vi "Text control 2 v7.4_pump-specific.vi"() -> ()   [LabVIEW 2019]
panel:
  in  "Tab Control":enum32{"Main", "Other parameters"}(tab)
  out "Vdg vs time (Bias Stress)":cluster{"Y data in":dbl[], "X data in":dbl[]}[](graph)
  out "Vp vs Vg (FPP)":cluster{"Y data in":dbl[], "X data in":dbl[]}[](graph)
  out "Vp vs time (FPP Bias Stress)":cluster{"Y data in":dbl[], "X data in":dbl[]}[](graph)
  out "Line running":i32
  out "Total lines":i32
  out "Path":path=path "C:/users/rlp38/09Apr2009LTtesting/test2.txt"
  out "I vs Vg":cluster{"Y data in":dbl[], "X data in":dbl[]}[](graph)
  out "Is max":dbl format="%.2e"
  out "Id max":dbl format="%.2e"
  out "Ig max":dbl format="%.2e"
  out "Imax vs time":cluster{"Y data in":dbl[], "X data in":dbl[]}[](graph)
  out "Imin vs time":cluster{"Y data in":dbl[], "X data in":dbl[]}[](graph)
  out "I vs Vd":cluster{"Y data in":dbl[], "X data in":dbl[]}[](graph)
  in  "Script":string
  out "Command running:":string
  out "Serial port data":string
  out "Elapsed Time":dbl caption="Elapsed Time (s)"
  in  "Time Units":u16(ring)=1 items=["Seconds", "Minutes", "Hours"]
  in  "Time Offset":dbl caption="Set Start Time (s)"
  in  "Reset":bool
  in  "Auto Reset":bool
  in  "integration time":u32(slide) max=2 step=1 scale=0.0..2.0
  in  "Interrupt scan":bool
  out "Absolute plunger position vs time":cluster{"Y data in":dbl[], "X data in":dbl[]}[](graph)
  out "Valve position vs time":cluster{"Y data in":dbl[], "X data in":dbl[]}[](graph)
  out "Is on":dbl format="%.2e"
  out "Id on":dbl format="%.2e"
  out "Ig on":dbl format="%.2e"
  out "Ion vs time":cluster{"Y data in":dbl[], "X data in":dbl[]}[](graph)
  out "Ioff vs time":cluster{"Y data in":dbl[], "X data in":dbl[]}[](graph)
  out "Ig min":dbl format="%.2e"
  out "Id min":dbl format="%.2e"
  out "Is min":dbl format="%.2e"
  out "Is off":dbl format="%.2e"
  out "Id off":dbl format="%.2e"
  out "Ig off":dbl format="%.2e"
  in  "Integration time (long)":dbl=0.32 min=0.04 max=2.0 step=0.02 format="%.2f"
  in  "Integration time (short)":dbl=0.0019 min=8e-05 max=0.0019 step=8e-05 format="%^.0e"
  in  "Gate: Compliance":dbl=0.001 format="%.8f"
  in  "Drain: Compliance":dbl=0.001 format="%.8f"
  in  "Hard stop pump":bool
  in  "Halt pump":bool
  in  "Interrupt program":bool
  in  "Suffix (script)":string="step_1_up-H2O_initial_script.txt"
  in  "Filename (variable part)":string="step_1_up-H2O_initial_"
  in  "Plot output curve extrema vs time":bool
  in  "Plot transfer curve extrema vs time":bool=TRUE
  in  "Plot sample extrema vs time":bool
  out "I vs time (Bias Stress)":cluster{"Y data in":dbl[], "X data in":dbl[]}[](graph)
  out "Vp1":dbl format="%.2e"
  out "Vp2":dbl format="%.2e"
  in  "Sample I - Probe 4 (Disabled)":u32(ring)=3 items=["SMU1  ", "SMU2  ", "SMU3  ", "SMU4  ", "SMU5  ", "SMU6  ", "VSU1  ", "VSU2  "]
  in  "Sample I - Source/Common":u32(ring) items=["SMU1  ", "SMU2  ", "SMU3  ", "SMU4  ", "SMU5  ", "SMU6  ", "VSU1  ", "VSU2  "]
  in  "Sample I - Probe 3 (Disabled)":u32(ring)=2 items=["SMU1  ", "SMU2  ", "SMU3  ", "SMU4  ", "SMU5  ", "SMU6  ", "VSU1  ", "VSU2  "]
  in  "Sample I - Drain/Gate":u32(ring)=1 items=["SMU1  ", "SMU2  ", "SMU3  ", "SMU4  ", "SMU5  ", "SMU6  ", "VSU1  ", "VSU2  "]
  in  "Sample - Probe 4":u32(ring)=3 items=["SMU1  ", "SMU2  ", "SMU3  ", "SMU4  ", "SMU5  ", "SMU6  ", "VSU1  ", "VSU2  "]
  in  "Sample - Source/Common":u32(ring) items=["SMU1  ", "SMU2  ", "SMU3  ", "SMU4  ", "SMU5  ", "SMU6  ", "VSU1  ", "VSU2  "]
  in  "Sample - Gate":u32(ring)=2 items=["SMU1  ", "SMU2  ", "SMU3  ", "SMU4  ", "SMU5  ", "SMU6  ", "VSU1  ", "VSU2  "]
  in  "Sample - Drain":u32(ring)=1 items=["SMU1  ", "SMU2  ", "SMU3  ", "SMU4  ", "SMU5  ", "SMU6  ", "VSU1  ", "VSU2  "]
  in  "VSU2 Stress - Source/Common":u32(ring) items=["SMU1  ", "SMU2  ", "SMU3  ", "SMU4  ", "SMU5  ", "SMU6  ", "VSU1  "]
  in  "Stress I - Source/Common":u32(ring) items=["SMU1  ", "SMU2  ", "SMU3  ", "SMU4  ", "SMU5  ", "SMU6  ", "VSU1  ", "VSU2  "]
  in  "Stress I - Drain/Gate":u32(ring)=1 items=["SMU1  ", "SMU2  ", "SMU3  ", "SMU4  ", "SMU5  ", "SMU6  ", "VSU1  ", "VSU2  "]
  in  "Stress V - Source/Common":u32(ring) items=["SMU1  ", "SMU2  ", "SMU3  ", "SMU4  ", "SMU5  ", "SMU6  ", "VSU1  ", "VSU2  "]
  in  "Stress V - Gate":u32(ring)=2 items=["SMU1  ", "SMU2  ", "SMU3  ", "SMU4  ", "SMU5  ", "SMU6  ", "VSU1  ", "VSU2  "]
  in  "Stress V - Drain":u32(ring)=1 items=["SMU1  ", "SMU2  ", "SMU3  ", "SMU4  ", "SMU5  ", "SMU6  ", "VSU1  ", "VSU2  "]
  in  "FPP - Source":u32(ring)=6 items=["SMU1  ", "SMU2  ", "SMU3  ", "SMU4  ", "SMU5  ", "SMU6  ", "VSU1  ", "VSU2  "]
  in  "FPP - Probe 2":u32(ring)=3 items=["SMU1  ", "SMU2  ", "SMU3  ", "SMU4  ", "SMU5  ", "SMU6  ", "VSU1  ", "VSU2  "]
  in  "FPP - Probe 1":u32(ring) items=["SMU1  ", "SMU2  ", "SMU3  ", "SMU4  ", "SMU5  ", "SMU6  ", "VSU1  ", "VSU2  "]
  in  "FPP - Gate":u32(ring)=2 items=["SMU1  ", "SMU2  ", "SMU3  ", "SMU4  ", "SMU5  ", "SMU6  ", "VSU1  ", "VSU2  "]
  in  "FPP - Drain":u32(ring)=1 items=["SMU1  ", "SMU2  ", "SMU3  ", "SMU4  ", "SMU5  ", "SMU6  ", "VSU1  ", "VSU2  "]
  in  "Pulsed Stress V - Vextra":u32(ring)=6 items=["SMU1  ", "SMU2  ", "SMU3  ", "SMU4  ", "SMU5  ", "SMU6  ", "VSU1  ", "VSU2  "]
  in  "Pulsed Stress V - Probe 4":u32(ring)=3 items=["SMU1  ", "SMU2  ", "SMU3  ", "SMU4  ", "SMU5  ", "SMU6  ", "VSU1  ", "VSU2  "]
  in  "Pulsed Stress V - Source/Common":u32(ring) items=["SMU1  ", "SMU2  ", "SMU3  ", "SMU4  ", "SMU5  ", "SMU6  ", "VSU1  ", "VSU2  "]
  in  "Pulsed Stress V - Gate":u32(ring)=2 items=["SMU1  ", "SMU2  ", "SMU3  ", "SMU4  ", "SMU5  ", "SMU6  ", "VSU1  ", "VSU2  "]
  in  "Pulsed Stress V - Drain":u32(ring)=1 items=["SMU1  ", "SMU2  ", "SMU3  ", "SMU4  ", "SMU5  ", "SMU6  ", "VSU1  ", "VSU2  "]
  in  "Transfer/Output - Probe 4":u32(ring)=3 items=["SMU1  ", "SMU2  ", "SMU3  ", "SMU4  ", "SMU5  ", "SMU6  ", "VSU1  ", "VSU2  "]
  in  "Transfer/Output - Source/Common":u32(ring) items=["SMU1  ", "SMU2  ", "SMU3  ", "SMU4  ", "SMU5  ", "SMU6  ", "VSU1  ", "VSU2  "]
  in  "Transfer/Output - Gate":u32(ring)=2 items=["SMU1  ", "SMU2  ", "SMU3  ", "SMU4  ", "SMU5  ", "SMU6  ", "VSU1  ", "VSU2  "]
  in  "Transfer/Output - Drain":u32(ring)=1 items=["SMU1  ", "SMU2  ", "SMU3  ", "SMU4  ", "SMU5  ", "SMU6  ", "VSU1  ", "VSU2  "]
  in  "Gate Range\nmode":u16(ring) items=["Auto", "Limited", "Fixed"]
  in  "Gate Range":u8(slide)=3 max=11 scale=0.0..11.0
  in  "Source/Drain\nRange mode":u16(ring) items=["Auto", "Limited", "Fixed"]
  in  "Source/Drain Range":u8(slide)=3 max=11 scale=0.0..11.0
  in  "Panel Controls":T1={"Emergency Stop"=refnum, "TransGraph Max"=1e-05, "Text/Graph (text=false)"=TRUE} {"TransGraph Max" format="%.2e"}
  in  "Panel Controls 2":T2={"Emergency Stop"=refnum, "TransGraph Max"=1e-05, "Text/Graph (text=false)"=TRUE, "TransGraph Min"=1e-11} {"TransGraph Min" format="%.2e"; "TransGraph Max" format="%.2e"}
  in  "Probe 4":cluster{"on/off":bool, "Voltage":dbl} {"Voltage" min=-100.0 max=100.0 format="%.2f"}
  in  "Full Reset":bool
  in  "Standby":T3
  out "error out":errorcluster
  in  "Delay before read (ms)":u32=1000
  in  "byte count":u32=64
  in  "Serial End Mode for Reads":u16(ring)=2 items=["None", "LastBit", "TermChar"]
  in  "Timeout (ms)":u32=10000
  in  "Enable Termination\nChar (T)":bool=TRUE
  in  "Termination char\n(0xA = '\\n' = LF)\n(0xD = '\\r' = CR)":u8=13 format="%.0x"
  in  "flow control":u16(ring) items=["None"=0, "XON/XOFF"=1, "RTS/CTS"=2, "DTR/DSR"=4]
  in  "stop bits":u16(ring)=10 items=["1.0"=10, "1.5"=15, "2.0"=20]
  in  "parity":u16(ring) items=["None", "Odd", "Even", "Mark", "Space"]
  in  "data bits":u16=8 min=5 max=8 step=1
  in  "VISA resource name":refnum<visa-resource-name>="COM6"
  in  "baud rate":u32=9600
  out "Timings Indicator":T4 {"integration time" scale=0.0..2.0}
  in  "Timings (overwritten by the Front Panel)":T5={"integration time"=0, "Short/Long integration time"=0.00064, "hold time (sec)"=0.0, "delay time (sec)"=0.0, "Step Time (0 disables)"=0.0, "sweep method"=0, "Pulse period"=0.005, "Base voltage"=0.0, "Pulse width"=0.0005} {"Pulse width" min=0.0005 max=0.1 step=0.0001 format="%.4f"; "Base voltage" format="%^.4e"; "Pulse period" min=0.005 max=1.0 step=0.0001 format="%.4f"; "sweep method" items=["Continuous", "Pulsed"]; "Step Time (0 disables)" format="%.2f"; "delay time (sec)" format="%.4f"; "hold time (sec)" format="%.4f"; "Short/Long integration time" format="%^.0e"; "integration time" scale=0.0..2.0}
  out "Probe 4 Indicator":cluster{"on/off":bool, "Voltage":dbl} {"Voltage" min=-100.0 max=100.0 format="%.2f"}
  in  "VISA resource name in":refnum<visa-resource-name>="GPIB0::14::INSTR"
  in  "Gate":T6={"Gate Start"=0.0, "Gate Stop"=2.0, "Gate Step (linear only)"=1.0, "Gate Compliance"=0.0001, "Gate PComp"=0.0, "Range mode"=0, "Range"=6} {"Range" max=11 scale=0.0..11.0; "Range mode" items=["Auto", "Limited", "Fixed"]; "Gate PComp" format="%^.2e"; "Gate Compliance" format="%^.2e"; "Gate Step (linear only)" format="%^.4e"; "Gate Stop" format="%^.4e"; "Gate Start" format="%^.4e"}
  in  "Drain 2":T7={"Drain Start"=0.0, "Drain Stop"=2.0, "Drain Compliance"=0.0001, "Drain Step"=1.0, "Drain PComp"=0.0, "Range mode"=0, "Range"=6} {"Range" max=11 scale=0.0..11.0; "Range mode" items=["Auto", "Limited", "Fixed"]; "Drain PComp" format="%^.2e"; "Drain Step" format="%^.4e"; "Drain Compliance" format="%^.2e"; "Drain Stop" format="%^.4e"; "Drain Start" format="%^.4e"}
  # "Syntax:\nitime [s|m|l] time(sec): [s|m|l] determines the integration time setting (small|medium|long) and time sets the value.\nNOTE: The value of the integration time has to be within the range allowed by its category (s|m|l), otherwise, the closest value will be used. (e.g. if the category is set to short but the time value is very long, the actual value used will be the maximum short integration time.\nIntegration times:\n    Short: Default: 640 us. Range: 8E-5 - 1.92E-3 seconds.\n    Medium: Fixed at 1 NPL cycle (0.02 seconds).\n    Long: Default: 16 NPL cycles (0.32 seconds). Range: 2-100 NPL cycles (0.04 seconds - 2 seconds).\ngaterangemode [a|l|f]\ndrainrangemode [a|l|f]\npulsed [on|off] PulsePeriod(sec) PulseBaseVoltage PulseONWidth(sec)\nstandby [on l off]\nwait NumMilliseconds\nwait-min NumMinutes\n# texthere = comment\nProbe4 [ON|OFF] Voltage\ntransfer [s|d] VgStart VgStop VgStep VdStart VdStop VdStep\noutput [s|d] VgStart VgStop VgStep VdStart VdStop VdStep\nsample Vg Vd NumSamples Time(s) SampleInterval(s)\nsamplei Idg NumSamples Time(s) SampleInterval(s) VDGcompliance\n100 samples is approximately 13 seconds with medium integration\n# If in doubt use SampleInterval(s) = 0.004\n    NOTE: When doing bias stress measurements, it is best to set the Time Units to \"Seconds\", as the \"sample\" command has been configured to give the output to seconds.\nstressV VG VD IGcompliance IDcompliance Duration(sec)\nstressI IDG VDGcompliance Duration(sec)\nvsu2pulse Bias Duration(s)\npulsedstressV [s|d] VEstop VgON VgOFF Period(s) PulseONwidth(s) Vd\nsample-fpp Vg Vd NumSamples Time\nresample-fpp Vg Vd\ntransfer-fpp [s|d] VgStart VgStop VgStep VdStart VdStop VdStep\noutput-fpp [s|d] VgStart VgStop VgStep VdStart VdStop VdStep\nserial SerialPortCommand\npump SerialPortCommand for the SPM pump\nloop(No of iterations){Code}: Iterates the code provided (including nested loops)\n\nSPM Pump Syntax (<x>: pump number, use 1 if only one pump):\nif the command syntax contains [R], then append the letter R to the command\n/<x>Q: query (a query command should follow each command)\n/<x>Z[R] or /<x>Y[R]: initialize pump\n/<x>N<n>[R] (<n>=0,1): <0> (<1>) microstep 0.01 mm (0.00125 mm) resolution\n/<x>I<n>[R] (<n>=0-6): turn to port number n (clockwise)\n/<x>O<n>[R] (<n>=0-6): turn to port number n (counterclockwise)\n/<x>X: Re-execute last command string\n/<x>G<n>[R] (<n>=0-60000): repeat command sequence (default: 0, 0=loop forever)\n/<x>g: Mark the start of a repeat sequence (max = 10)\n/<x>M<n>[R] (<n>=0-86400000): delay command execution by n milliseconds\n/<x>H: Halt; Pause the sequence after finishing the current move\n/<x>T: Hardstop; Interrupt the current move and suppress it from the sequence\n/<x>A<n>[R] (<n>=0-3000 with N=0, 0-24000 with N=1): absolute position\n/<x>P<n>[R] (<n>=0-3000 with N=0, 0-24000 with N=1): relative pickup\n/<x>D<n>[R] (<n>=0-3000 with N=0, 0-24000 with N=1): relative dispense\n/<x>V<n>[R] (<n>=1-1600 default: 150): set peak speed (pulses/sec)\nNOTE: The lowest speed limit is 1 pulse/sec, not 5, as the manual states.\n/<x>S<n>[R] (<n>=10-40 default: 22): set speed (NOT in pulses/sec, look in manual)\nNOTE: When controlled with absolute position, one does not need to pay special attention to the syringe that is mounted on the pump.\nWithdraw from lower stage (ports 3, 5), dispense from higher stage (ports 2, 4, 6).\nConnect Port 1 to waste."
  # "Time"
  # "1\n2\n3\n4\n5\n6\n7\n8\n9\n10\n11\n12\n13\n14\n15\n16\n17\n18\n19\n20"
  # "Serial port settings"
  # "SMUs"
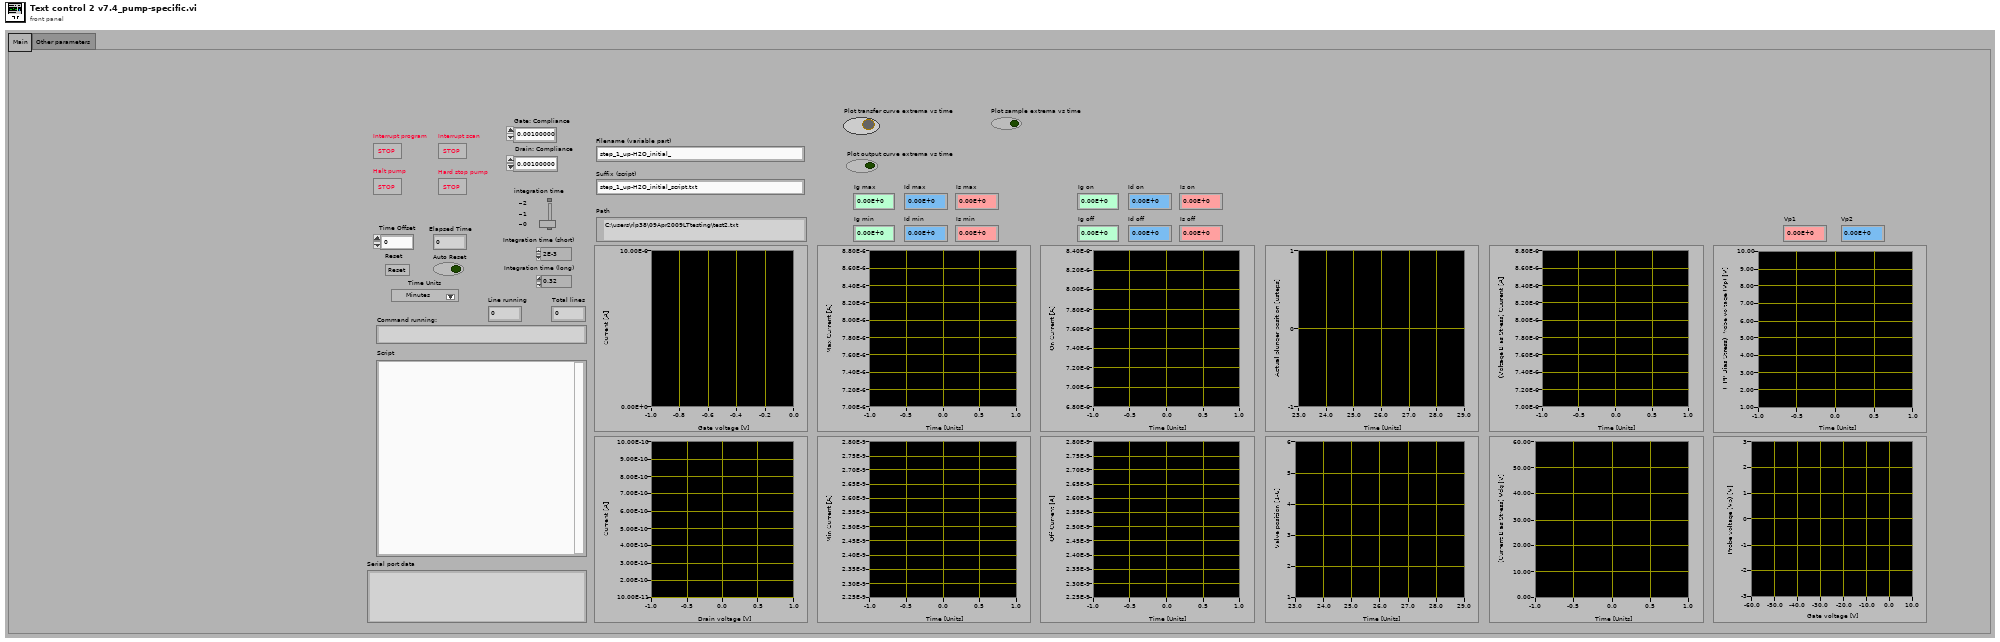
[diagram p1: front panel]
types:
  T1 = cluster{"Emergency Stop":refnum<vi>, "TransGraph Max":dbl, "Text/Graph (text=false)":bool}
  T2 = cluster{"Emergency Stop":refnum<vi>, "TransGraph Max":dbl, "Text/Graph (text=false)":bool, "TransGraph Min":dbl}
  T3 = cluster{"Gate Standby":bool, "Drain Standby":bool}
  T4 = cluster{"Short/Long integration time":dbl, "hold time (sec)":dbl, "delay time (sec)":dbl, "Step Time (0 disables)":dbl, "sweep method":u16, "Pulse period":dbl, "Base voltage":dbl, "Pulse width":dbl, "integration time":u32}
  T5 = cluster{"integration time":u32, "Short/Long integration time":dbl, "hold time (sec)":dbl, "delay time (sec)":dbl, "Step Time (0 disables)":dbl, "sweep method":u16, "Pulse period":dbl, "Base voltage":dbl, "Pulse width":dbl}
  T6 = cluster{"Gate Start":dbl, "Gate Stop":dbl, "Gate Step (linear only)":dbl, "Gate Compliance":dbl, "Gate PComp":dbl, "Range mode":u16, "Range":u8}
  T7 = cluster{"Drain Start":dbl, "Drain Stop":dbl, "Drain Compliance":dbl, "Drain Step":dbl, "Drain PComp":dbl, "Range mode":u16, "Range":u8}
  T8 = enum16{"open", "replace", "create", "open or create", "replace or create", "replace or create with confirmation"}
  T9 = cluster{"V2 Start":dbl, "V2 Step":dbl, "Number of points":i32}
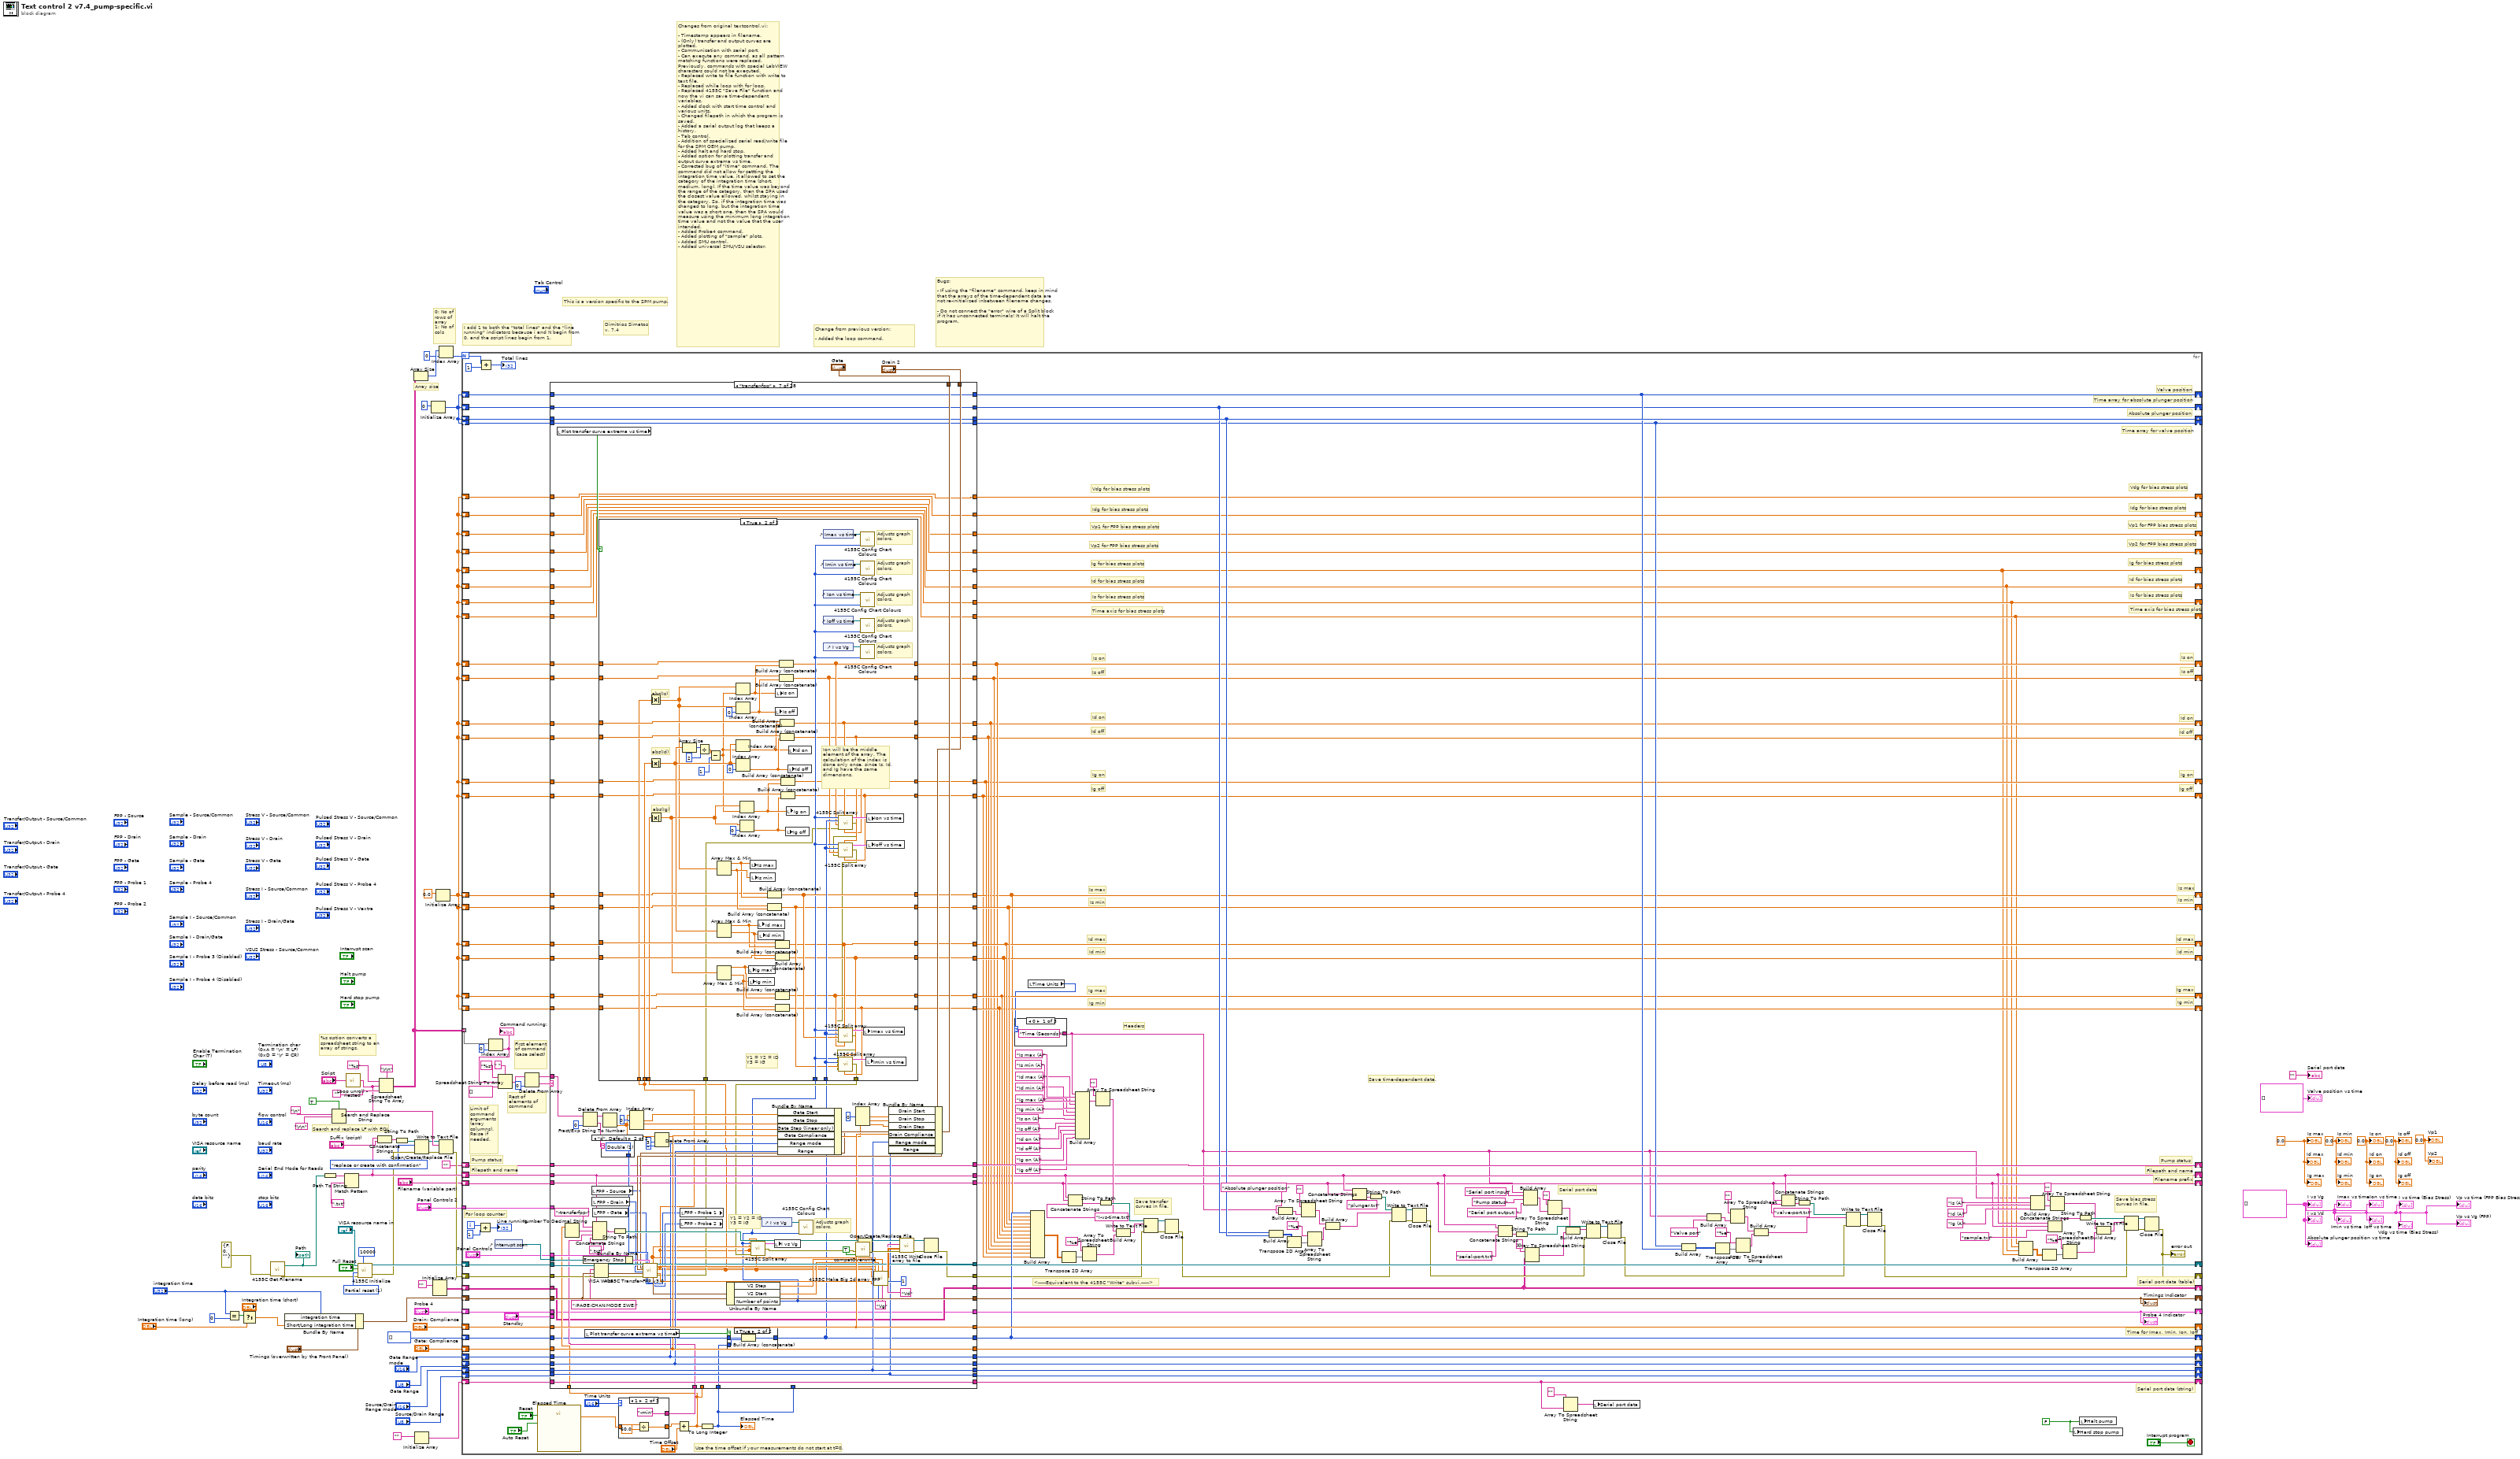
[diagram p0: block diagram]
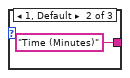
[diagram p2: hidden frame]
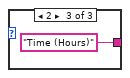
[diagram p3: hidden frame]
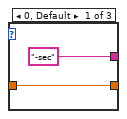
[diagram p4: hidden frame]
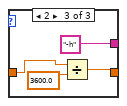
[diagram p5: hidden frame]
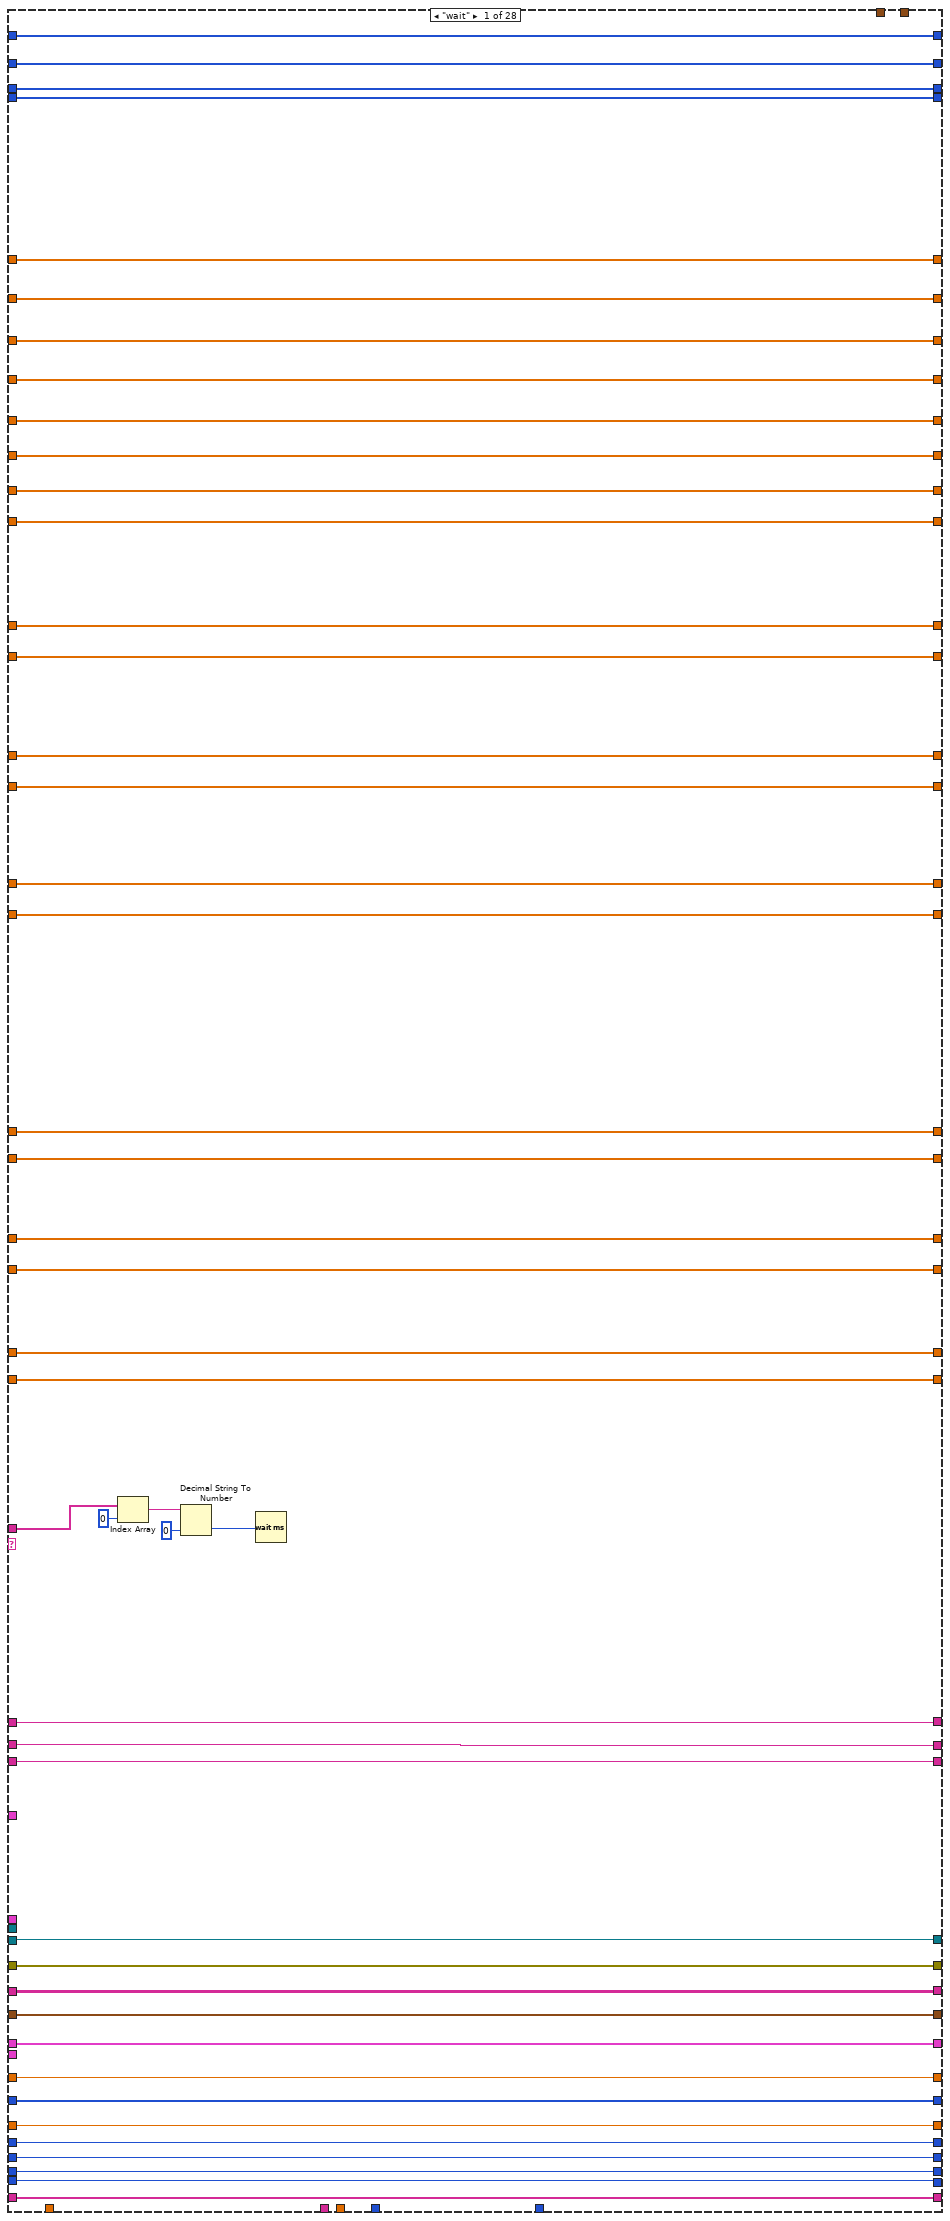
[diagram p6: hidden frame]
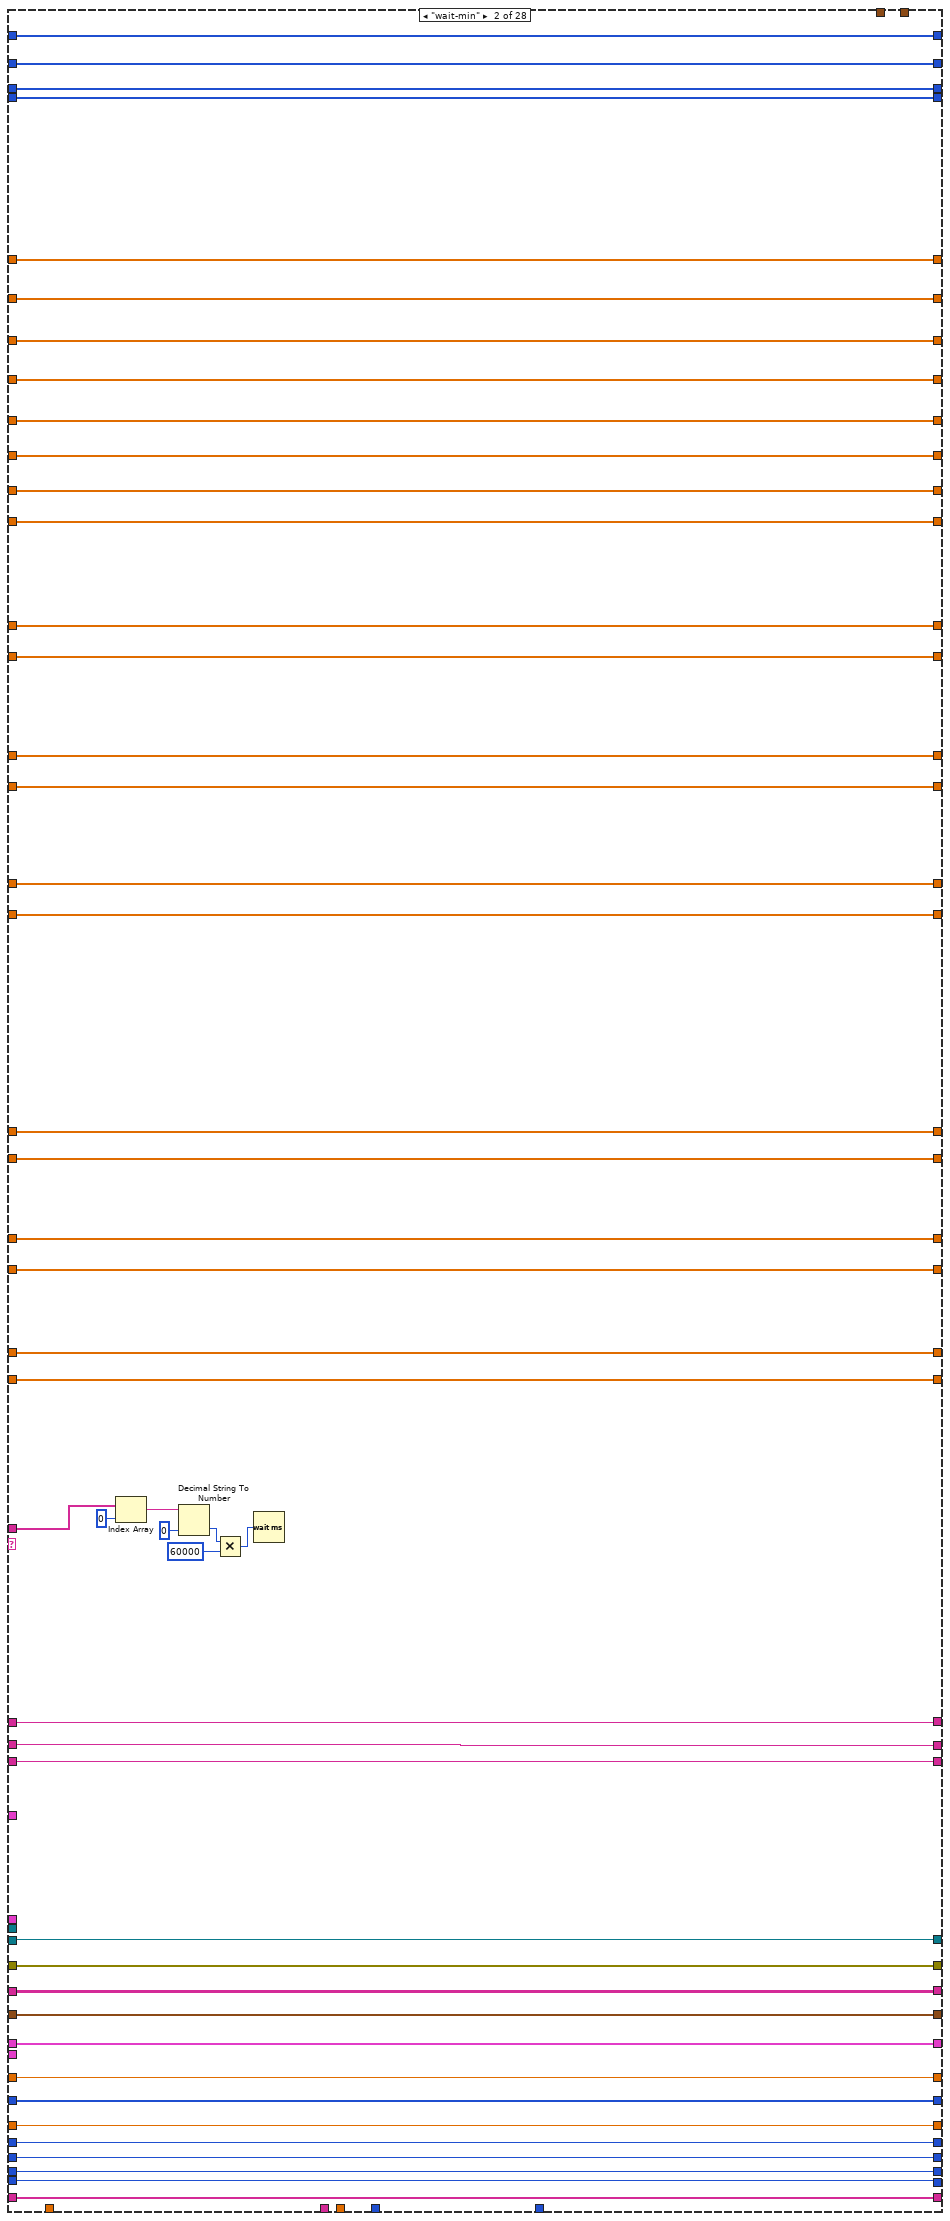
[diagram p7: hidden frame]
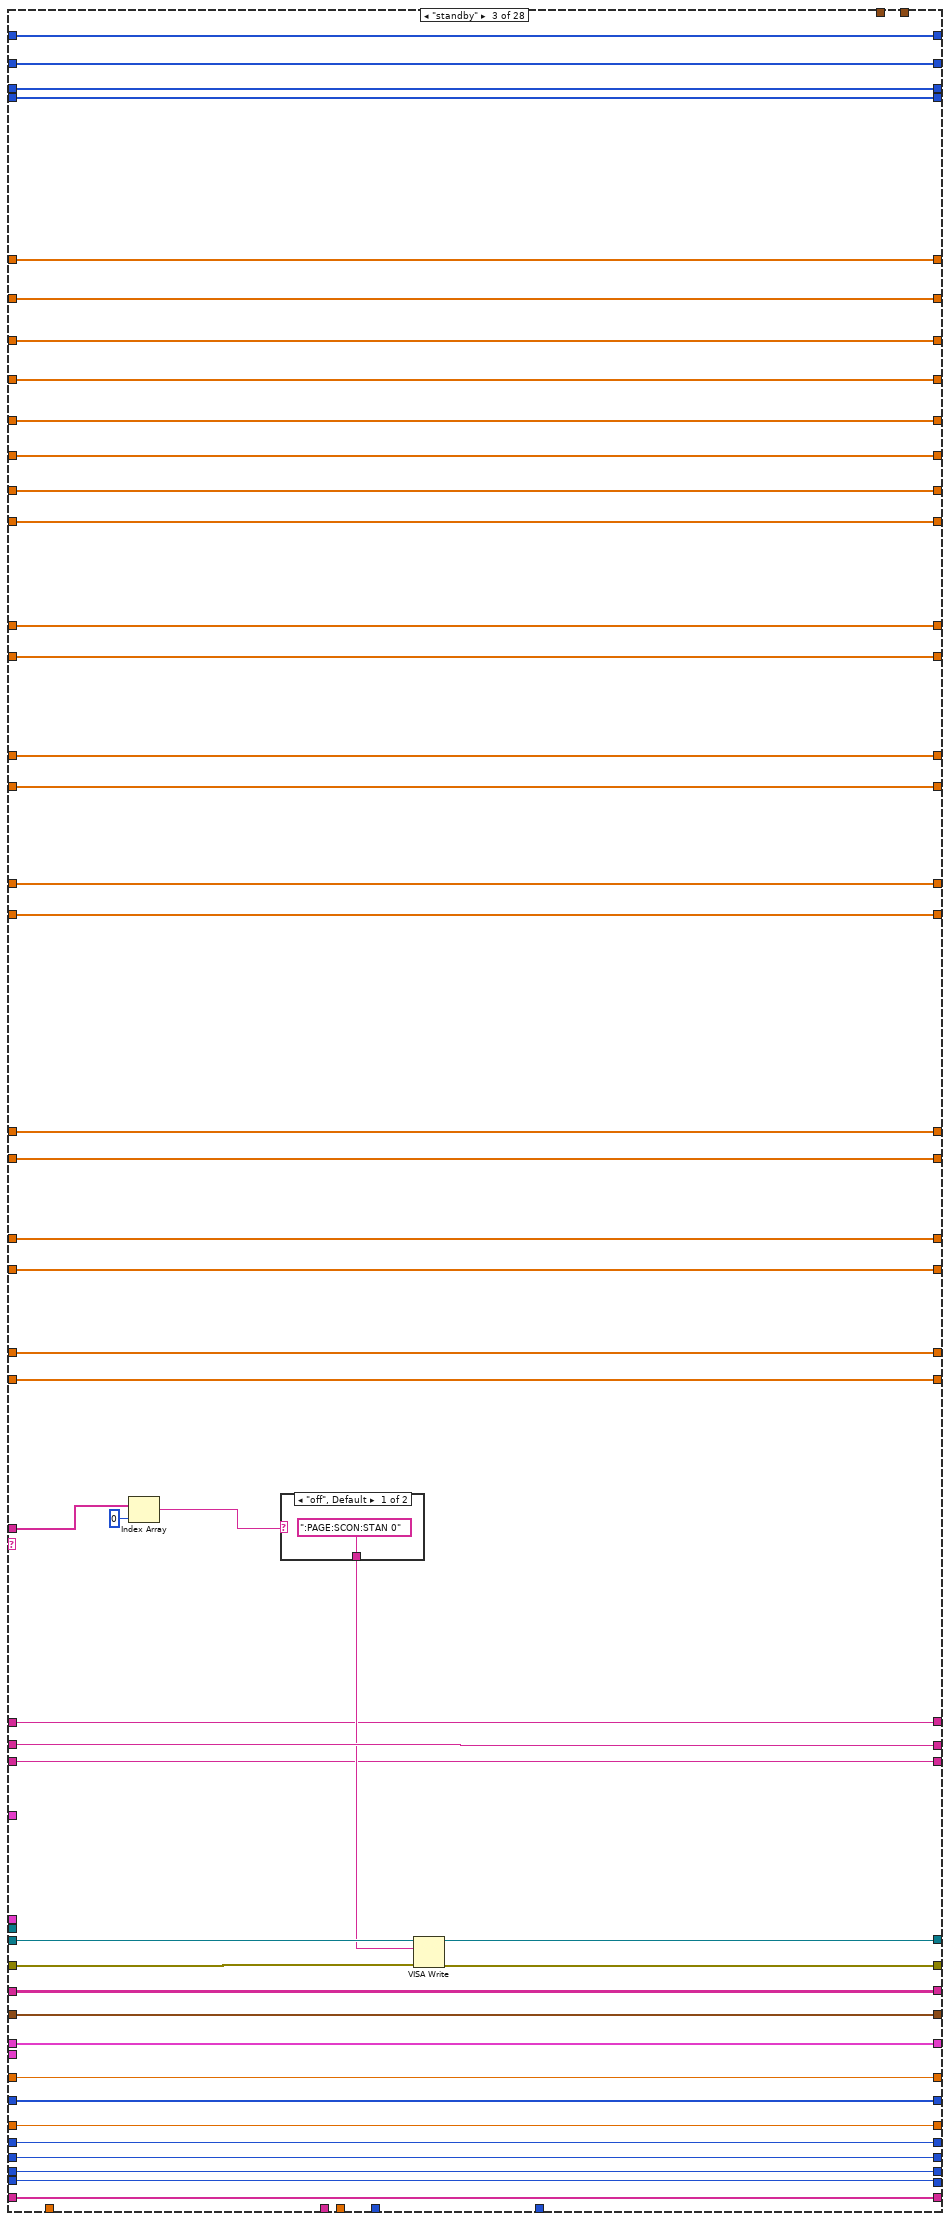
[diagram p8: hidden frame]
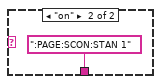
[diagram p9: hidden frame]
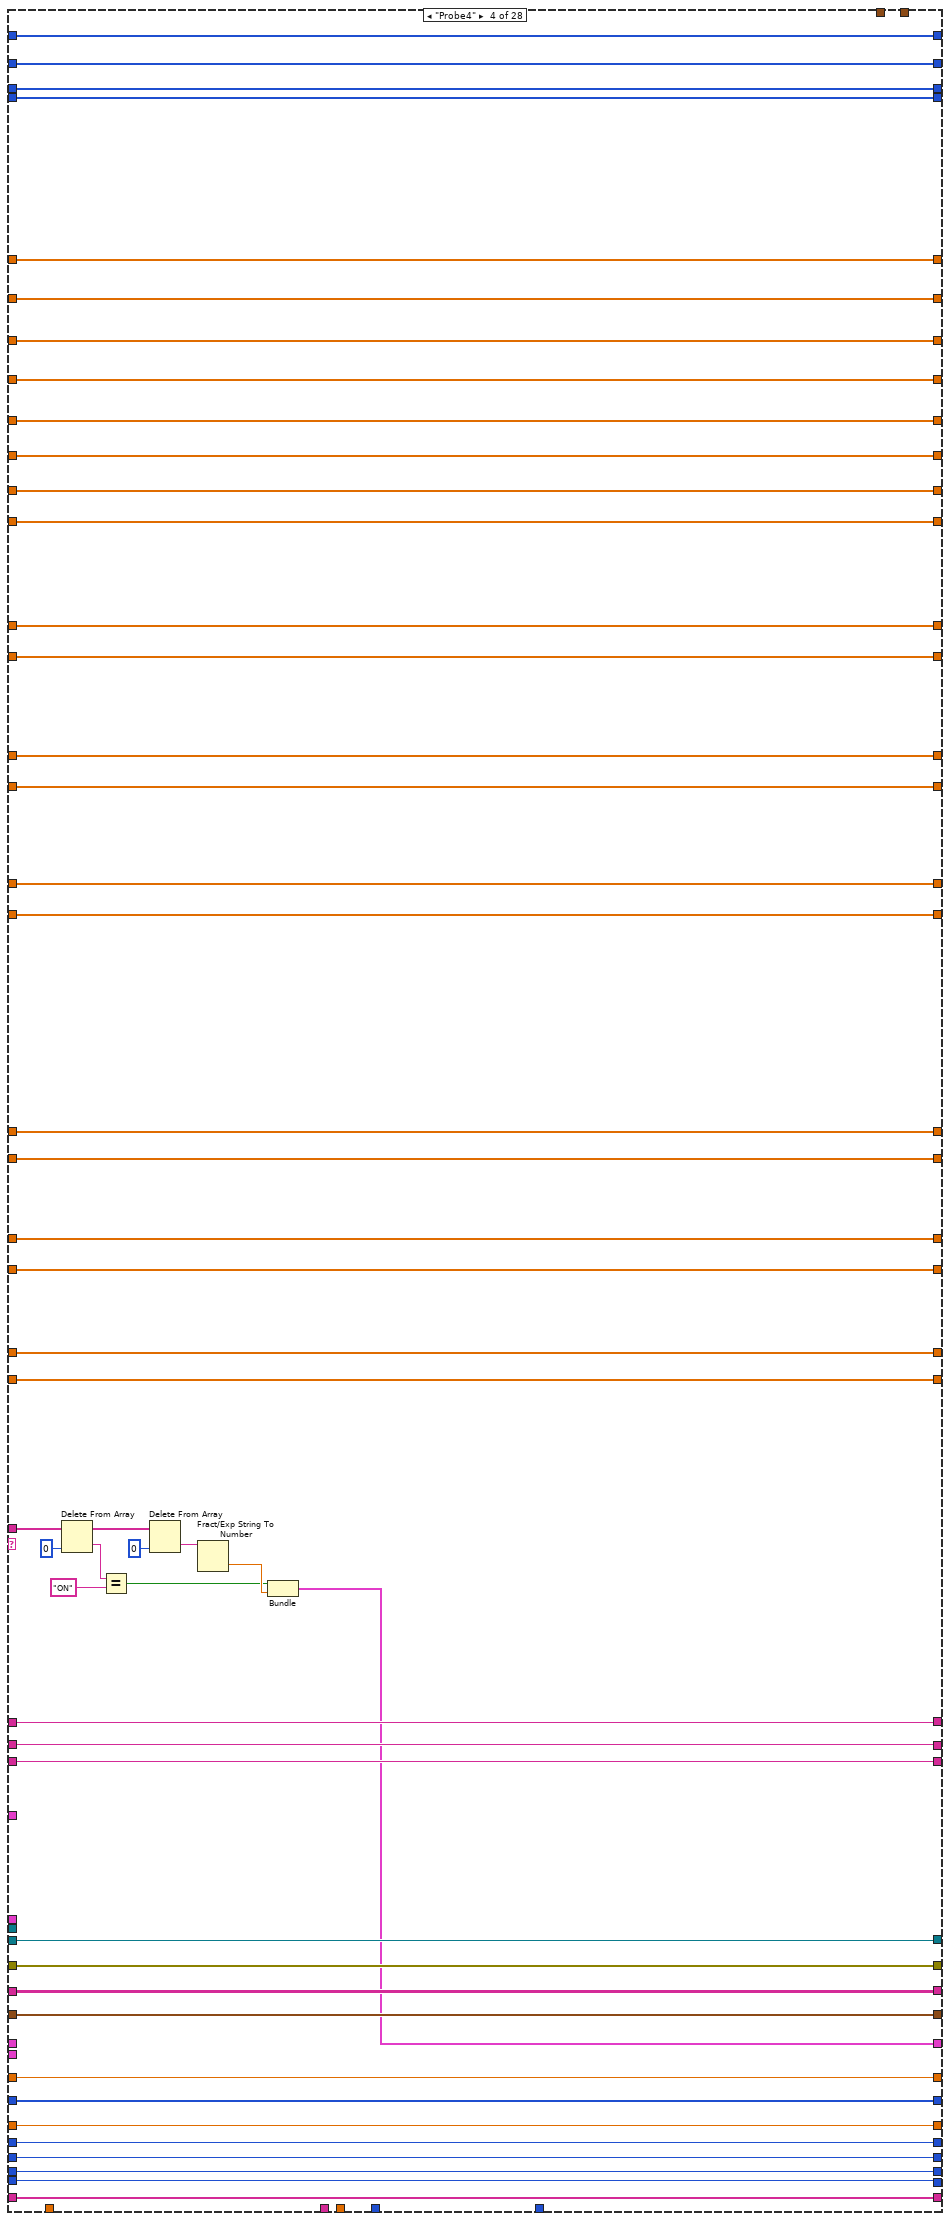
[diagram p10: hidden frame]
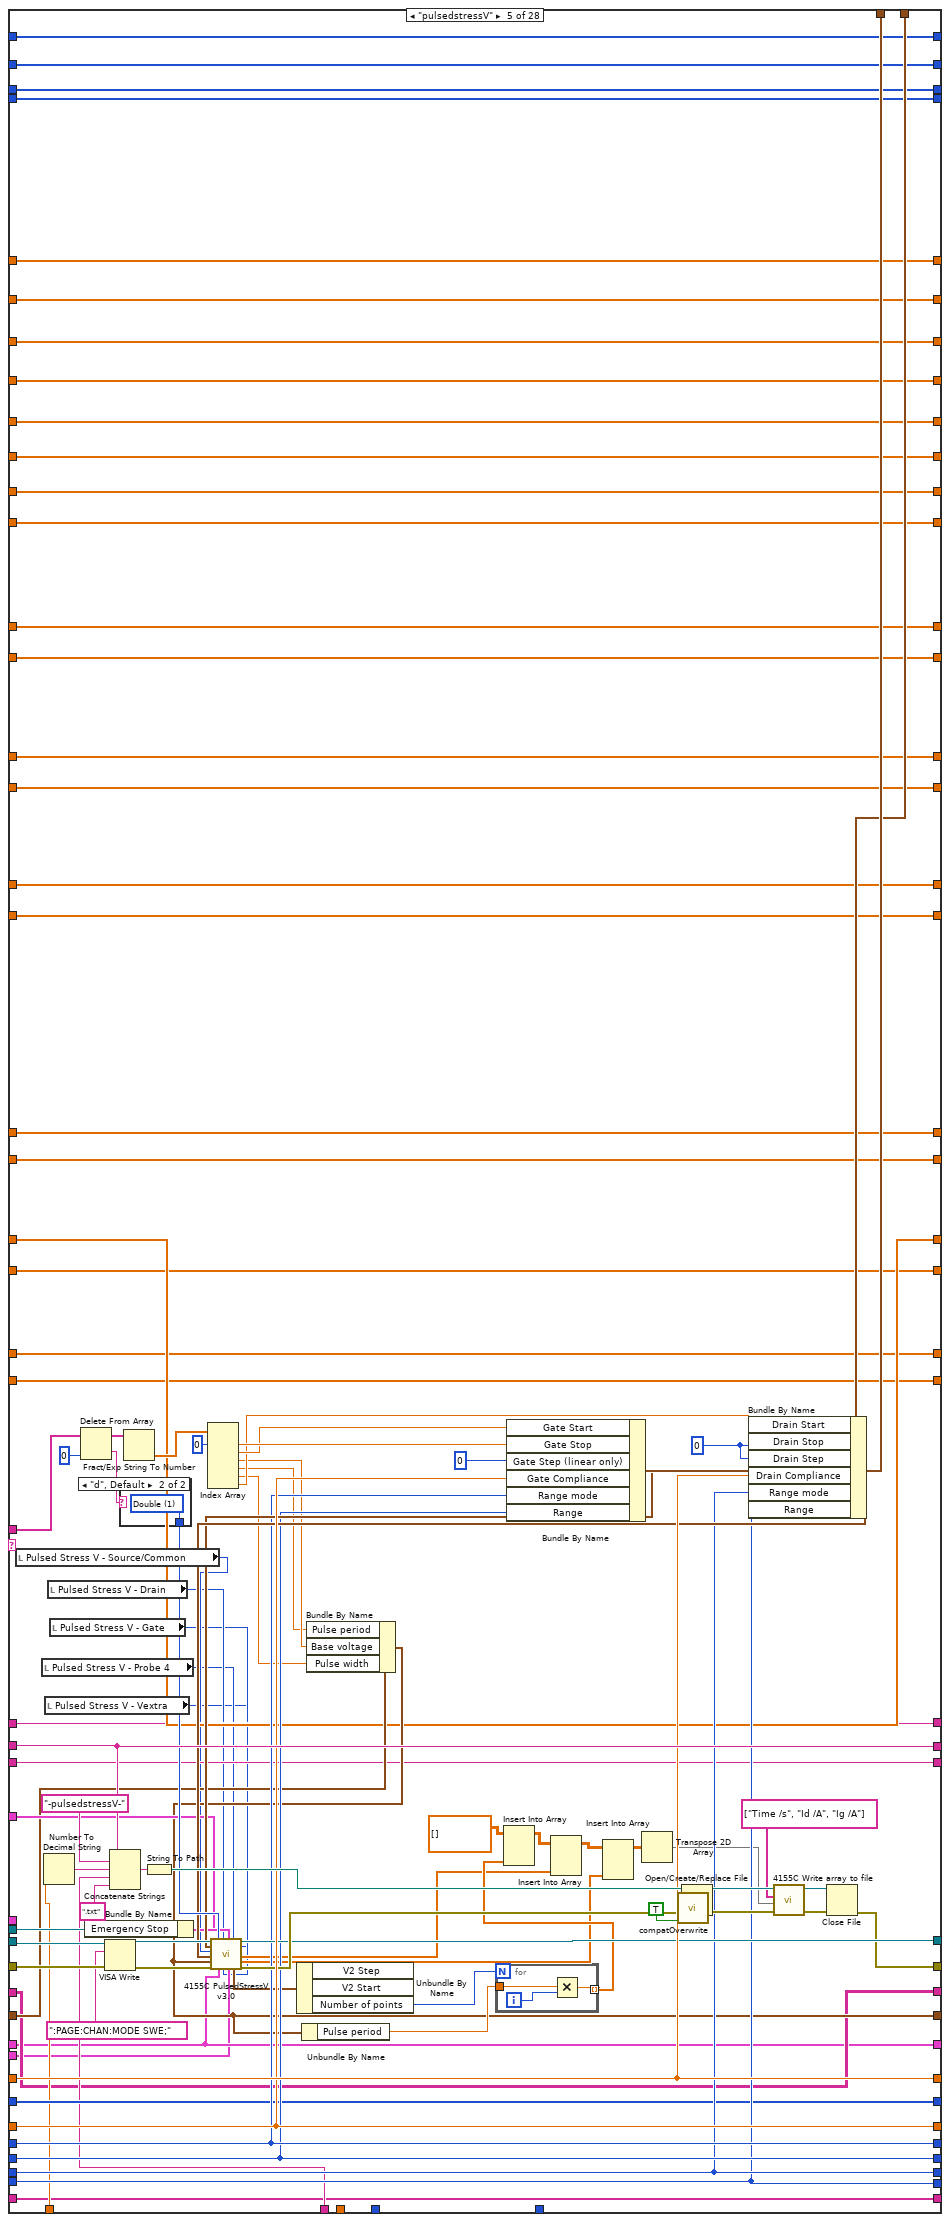
[diagram p11: hidden frame]
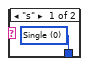
[diagram p12: hidden frame]
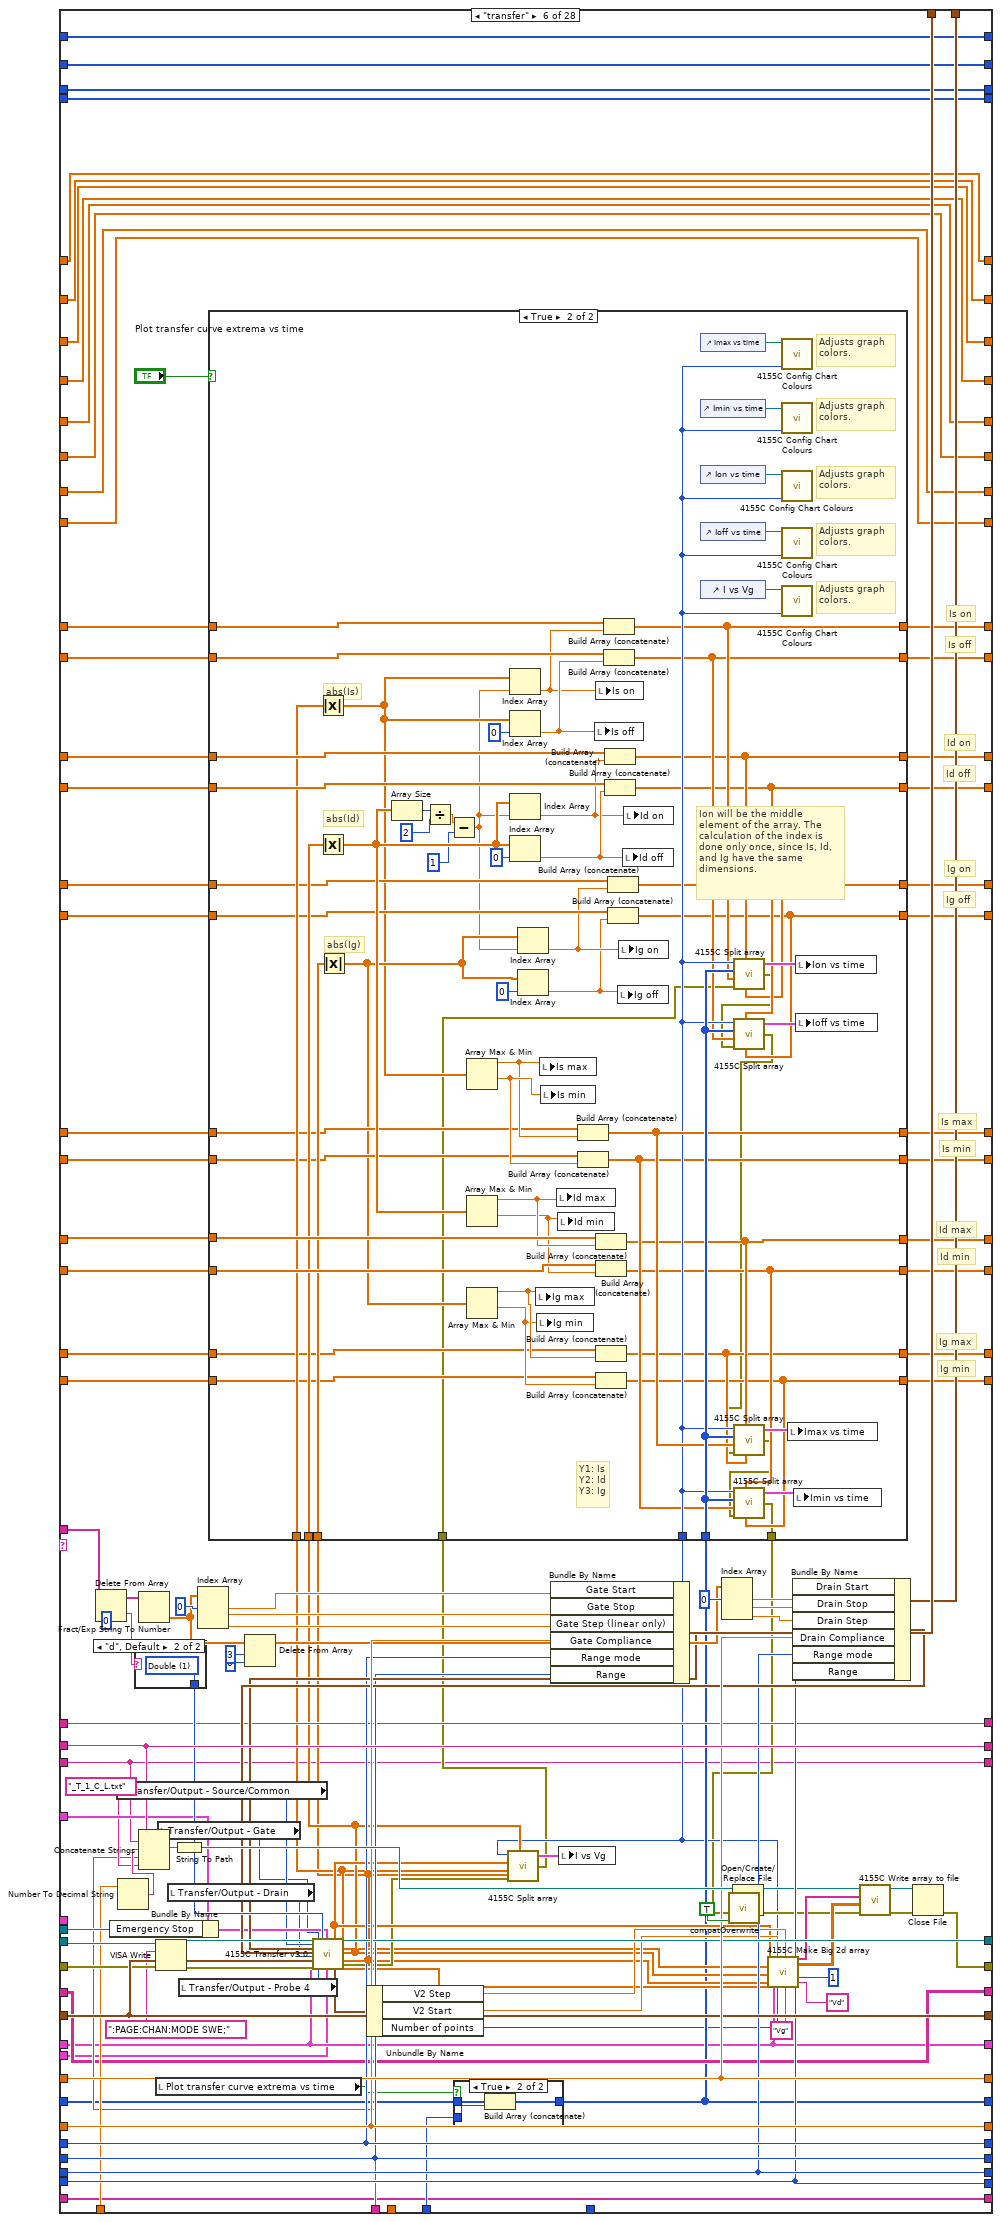
[diagram p13: hidden frame]
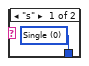
[diagram p16: hidden frame]
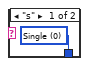
[diagram p19: hidden frame]
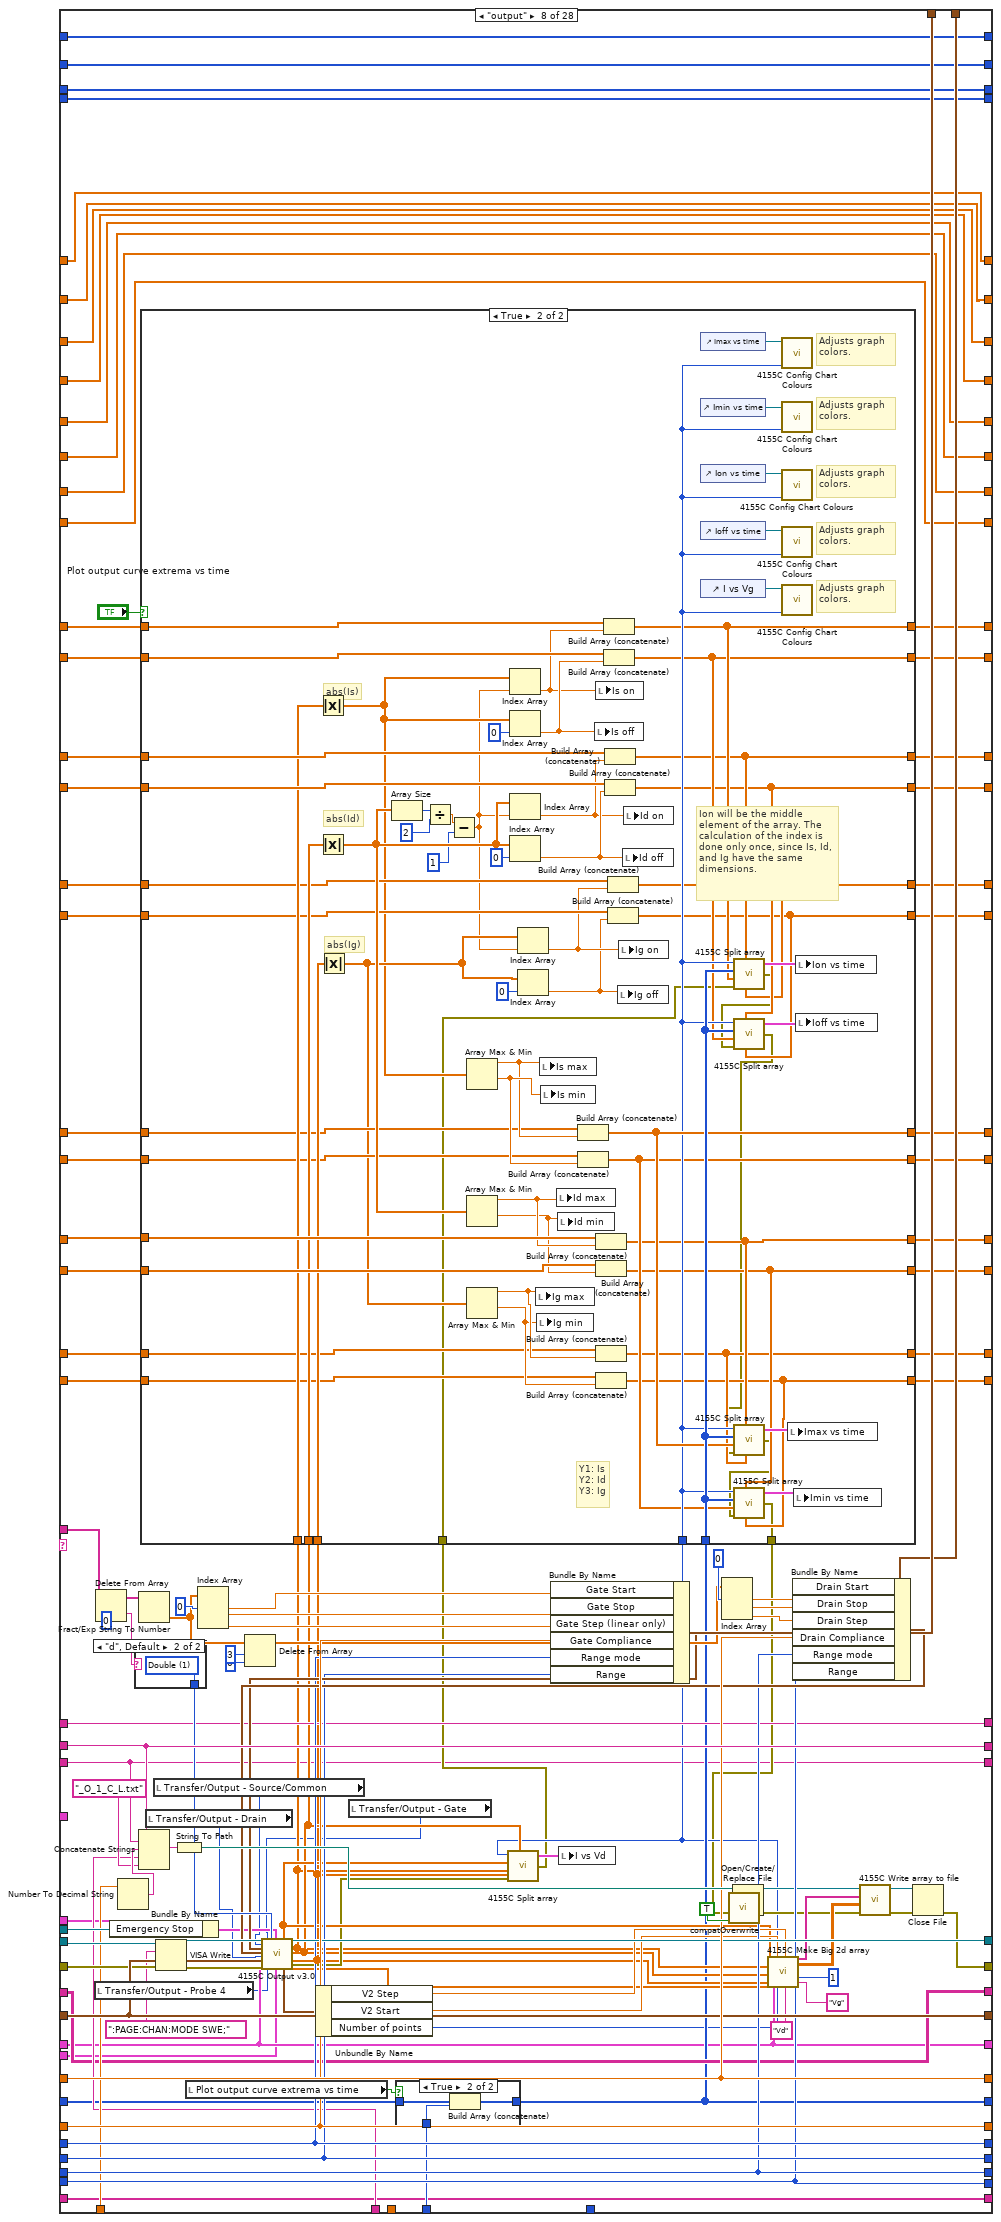
[diagram p20: hidden frame]
diagram:
  w5 = 0.0 ("Is off")
  w4 = cluster{"Y data in":dbl[], "X data in":dbl[]}[] [] ("I vs Vg")
  w14 = 0.0 ("Is off")
  w15 = 0.0 ("Is on")
  w16 = 0.0 ("Is min")
  w17 = 0.0 ("Is max")
  w62 = u16 1 items=["Reset All", "Partial reset"] ("Type of reset")
  # "Change from previous version:\n\n- Added the loop command."
  # "This is a version specific to the SPM pump."
  # "I add 1 to both the \"total lines\" and the \"line running\" indicators because i and N begin from 0, and the script lines begin from 1."
  # "Bugs:\n\n- If using the \"filename\" command, keep in mind that the arrays of the time-dependent data are not re-initialized inbetween filename changes. \n\n- Do not connect the \"error\" wire of a Split block if it has unconnected terminals! It will halt the program."
  # "Array size"
  # "%s option converts a spreadsheet string to an array of strings."
  # "0: No of rows of array\n1: No of cols"
  # "Dimitrios Simatos\nv. 7.4"
  # "Changes from original textcontrol.vi:\n\n- Timestamp appears in filename.\n- (Only) transfer and output curves are plotted.\n- Communication with serial port.\n- Can execute any command, as all pattern matching functions were replaced. Previously, commands with special LabVIEW characters could not be executed.\n- Replaced write to file function with write to text file.\n- Replaced while loop with for loop.\n- Replaced 4155C \"Save File\" function and now the vi can save time-dependent variables.\n- Added clock with start time control and various units.\n- Changed filepath in which the program is saved.\n- Added a serial output log that keeps a history.\n- Tab control.\n- Addition of specialized serial read/write file for the SPM OEM pump.\n- Added halt and hard stop.\n- Added option for plotting transfer and output curve extrema vs time.\n- Corrected bug of \"itime\" command. The command did not allow for settting the integration time value, it allowed to set the category of the integration time (short, medium, long). If the time value was beyond the range of the category, then the SPA used the closest value allowed, whilst staying in the category. So, if the integration time was changed to long, but the integration time value was a short one, then the SPA would measure using the minimum long integration time value and not the value that the user intended.\n- Added Probe4 command.\n- Added plotting of \"sample\" plots.\n- Added SMU control.\n- Added universal SMU/VSU selector."
  # "Search and replace LF with EOL"
  n1 = Equal?(x="integration time", y=u32 0) -> (x = y?=w63:bool)
  n2 = Select(t="Integration time (short)", s=w63, f="Integration time (long)") -> (s? t:f=w18:dbl)
  n3 = call "4155C Get Filename.vi"("error in (no error)"=errorcluster {"status"=FALSE, "code"=0, "source"=""}) -> ("error out"=w57:errorcluster, "path"=w33:path)  [unwired: 2 in, 1 out]
  "Path" <- w33
  n4 = Bundle By Name(cluster="Timings (overwritten by the Front Panel)", "integration time"="integration time", "Short/Long integration time"=w18) -> (w55:T5)
  n5 = Path To String(path=w33) -> (string=w34:string)
  n6 = Match Pattern(string=w34, regular expression=".txt") -> (before substring=w30:string)  [unwired: 1 in, 3 out]
  n7 = call "Loop unroll - nested.vi"("Script"="Script") -> ("Output"=w2:string)
  n8 = Search and Replace String(replace all?=TRUE ("replace all? (F)"), input string=w2, search string="\n", replace string="\r\n") -> (result string=w45:string)  [unwired: 4 in, 3 out]
  n9 = call "4155C Initialise.vi"("VISA resource name in"="VISA resource name in", "Reset"="Full Reset", "Type of reset"=w62, "error in (no error)"=w57, "VISA Timeout Value"=u32 10000) -> ("VISA Resource Name out"=w56:refnum<visa-resource-name>, "error out"=w7:errorcluster)
  n10 = Concatenate Strings(w30, "Suffix (script)") -> (w29:string)
  n11 = Spreadsheet String To Array(delimiter (Tab)="\r\n", format string="%s", spreadsheet string=w2, array type (2D Dbl)="") -> (array=w36:string[][])
  n12 = String To Path(string=w29) -> (path=w10:path)
  n13 = Array Size(array=w36) -> (size(s)=w40:i32[])
  n14 = Initialize Array("") -> (w22:string[])  [unwired: 1 in]
  n15 = Open/Create/Replace File(file path (use dialog)=w10, error in=w7, operation (0:open)=T8."replace or create with confirmation") -> (refnum out=w9:refnum<file>, error out=w8:errorcluster)  [unwired: 3 in, 1 out]
  n16 = Initialize Array(0 ("element")) -> (w24:i32[])  [unwired: 1 in]
  n17 = Initialize Array("") -> (w20:string[][])  [unwired: 2 in]
  n18 = Initialize Array(0.0 ("element")) -> (w3:dbl[])  [unwired: 1 in]
  n19 = Index Array(array=w40, index=0) -> (element=w38:i32)
  n20 = Write to Text File(file (use dialog)=w9, text=w45, error in=w8) -> (error out=w28:errorcluster)  [unwired: 1 in, 2 out]
  n21 = for {
    N: w38 -> [w216]
    shift-left: "Source/Drain Range" -> [w256]
    shift-right: [w252] -> _
    shift-left: "Source/Drain\nRange mode" -> [w257]
    shift-right: [w253] -> _
    shift-left: "Gate Range" -> [w258]
    shift-right: [w254] -> _
    shift-left: "Gate Range\nmode" -> [w259]
    shift-right: [w255] -> _
    shift-left: "Gate: Compliance" -> [w267]
    shift-right: [w264] -> _
    shift-left: "Drain: Compliance" -> [w268]
    shift-right: [w265] -> _
    shift-left: w55 -> [w269]
    shift-right: [w78] -> _
    shift-left: w28 -> [w270]
    shift-right: [w77] -> _
    shift-left: w56 -> [w271]
    shift-right: [w266] -> _
    shift-left: w30 -> [w272]
    shift-right: [w87] -> _
    tunnel: "Panel Controls 2" -> [w250]
    shift-right: [w128] -> _
    shift-left: w3 -> [w249]
    shift-right: [w186] -> _
    shift-left: i32[] [] -> [w245]
    tunnel: w36 -> [w244] mode=indexing
    shift-right: [w127] -> _
    shift-left: w3 -> [w221]
    shift-right: [w159] -> _
    shift-left: w22 -> [w208]
    shift-right: [w187] -> _
    shift-left: w24 -> [w203]
    shift-right: [w169] -> _
    shift-left: w24 -> [w202]
    shift-right: [w201] -> _
    shift-left: "" -> [w200]
    shift-right: [w164] -> _
    shift-left: w24 -> [w184]
    shift-right: [w163] -> _
    shift-left: w24 -> [w168]
    shift-right: [w160] -> _
    shift-left: w20 -> [w162]
    shift-right: [w121] -> _
    shift-left: w3 -> [w149]
    shift-right: [w122] -> _
    shift-left: w3 -> [w148]
    shift-right: [w126] -> _
    shift-left: w3 -> [w137]
    shift-right: [w125] -> _
    shift-left: w3 -> [w136]
    shift-right: [w119] -> _
    shift-left: w3 -> [w135]
    shift-right: [w129] -> _
    shift-left: w3 -> [w134]
    shift-right: [w120] -> _
    shift-left: w3 -> [w133]
    shift-right: [w118] -> _
    shift-left: w3 -> [w132]
    shift-right: [w124] -> _
    shift-left: w3 -> [w131]
    shift-right: [w123] -> _
    shift-left: w3 -> [w130]
    shift-right: [w86] -> _
    shift-left: "Filename (variable part)" -> [w113]
    shift-right: [w79] -> _
    shift-left: "Probe 4" -> [w251]
    shift-right: [w82] -> _
    shift-left: w3 -> [w108]
    shift-right: [w83] -> _
    shift-left: w3 -> [w107]
    shift-right: [w84] -> _
    shift-left: w3 -> [w106]
    shift-right: [w85] -> _
    shift-left: w3 -> [w105]
    shift-right: [w73] -> _
    shift-left: w3 -> [w76]
    shift-right: [w74] -> _
    shift-left: w3 -> [w75]
    shift-right: [w69] -> _
    shift-left: w3 -> [w70]
    shift-right: [w68] -> _
    shift-left: w3 -> [w71]
    i -> [w211]
    stop <- "Interrupt program" stop-if-true
    w72 = FALSE
    # "Vdg for bias stress plots"
    # "Idg for bias stress plots"
    # "Vp2 for FPP bias stress plots"
    # "Vp1 for FPP bias stress plots"
    # "Ig for bias stress plots"
    # "Id for bias stress plots"
    # "Is for bias stress plots"
    # "Time axis for bias stress plots"
    # "Is off"
    # "Is on"
    # "Ig off"
    # "Ig on"
    # "Is min"
    # "Is max"
    # "Ig min"
    # "Ig max"
    # "Id min"
    # "Id max"
    # "Id off"
    # "Id on"
    # "Vdg for bias stress plots"
    # "Idg for bias stress plots"
    # "Vp2 for FPP bias stress plots"
    # "Vp1 for FPP bias stress plots"
    # "Ig for bias stress plots"
    # "Id for bias stress plots"
    # "Is for bias stress plots"
    # "Time axis for bias stress plots"
    # "Save bias stress curves in file."
    # "Filename prefix"
    # "Is off"
    # "Is on"
    # "Ig off"
    # "Ig on"
    # "Is min"
    # "Is max"
    # "Ig min"
    # "Ig max"
    # "Id min"
    # "Id max"
    # "Id off"
    # "Id on"
    # "Pump status"
    # "Filepath and name"
    # "Pump status"
    # "Limit of command arguments (array columns). Raise if needed."
    # "Serial port data (string)"
    # "Serial port data (table)"
    # "Time array for valve position"
    # "Time array for absolute plunger position"
    # "Valve position"
    # "Absolute plunger position"
    # "Serial port data"
    # "For loop counter"
    # "<-----Equivalent to the 4155C \"Write\" subvi.----->"
    # "Headers"
    # "Save transfer curves in file."
    # "Filepath and name"
    # "Save time-dependent data."
    # "Use the time offset if your measurements do not start at t=0."
    # "Time for Imax, Imin, Ion, Ioff"
    # "Rest of elements of command"
    # "First element of command\n(case select)"
    n22 = Add(x=w211, y=1) -> (x+y=→"Line running":i32)
    n23 = Add(x=w216, y=1) -> (x+y=→"Total lines":i32)
    n24 = Index Array(array=w244, index=0 ("line index")) -> (element=w239:string)
    "Command running:" <- w239
    n25 = control-ref of="Interrupt scan"() -> (w263:refnum<vi>)
    n26 = Spreadsheet String To Array(delimiter (Tab)=" ", format string="%s", spreadsheet string=w239, array type (2D Dbl)=string[] []) -> (array=w237:string[])
    n27 = Delete From Array(array=w237, index=0) -> (deleted portion=w150:string, array with subset deleted=w236:string[])  [unwired: 1 in]
    n28 = call "Elapsed Time"("Reset"="Reset", "Auto Reset"="Auto Reset") -> ("Elapsed Time (s)"=w246:dbl)  [unwired: 10 in, 7 out]
    n29 = case shown="1" "Time Units" {
      tunnel: ["-sec" "-min" "-h"] -> w247
      tunnel: [w276 w280 w283] -> w217
      tunnel: w246 -> [w276 w279 w284]
      frame 0, Default {
      }
      frame 1 {
        n30 = Divide(x=w279, y=60.0) -> (x/y=w280:dbl)
      }
      frame 2 {
        n31 = Divide(x=w284, y=3600.0) -> (x/y=w283:dbl)
      }
    }
    n32 = Add(x=w217, y="Time Offset") -> (x+y=w109:dbl)
    n33 = To Long Integer(number=w109) -> (32bit integer=w110:i32)
    "Elapsed Time" <- w110
    n34 = case shown="\"transfer-fpp\"" w150 {
      tunnel: w236 -> [w330 w377 w423 w435 w501 w689 w824 w1101 w1237 w1418 w1507 w1562 w1615 w1664 w1706 _ _ w1929 w2085 _ w2218 w2292 w2363 w2490 w2648 w2740 w2817 w2874]
      tunnel: w272 -> [w325 w373 w421 w457 w565 w696 w894 w1108 w1307 w1441 w1496 w1554 w1608 w1658 w1699 w1746 w1816 w1856 w2069 w2135 w2205 w2279 w2351 w2484 w2644 w2742 w2819 w2876]
      tunnel: w271 -> [w324 w372 w412 w455 w550 w667 w865 w1079 w1277 w1442 w1497 w1555 w1609 w1659 w1700 w1751 w1818 w1934 w2091 w2139 w2224 w2298 w2369 w2496 w2608 w2746 w2823 w2878]
      tunnel: w270 -> [w323 w371 w411 w454 w549 w666 w864 w1078 w1274 w1443 w1498 w1556 w1610 w1660 w1701 w1750 w1789 w1933 w2090 w2138 w2223 w2297 w2368 w2495 w2607 w2745 w2822 w2879]
      tunnel: w269 -> [w322 w370 w420 w452 w526 w692 w890 w1104 w1303 w1451 w1506 w1553 w1607 w1657 w1698 w1749 w1813 w1904 w2061 w2144 w2198 w2272 w2344 w2483 w2643 w2747 w2824 w2881]
      tunnel: w268 -> [w321 w369 w419 w451 w563 w694 w892 w1106 w1305 w1450 w1505 w1561 w1614 w1663 w1705 w1748 w1798 w1932 w2089 w2147 w2222 w2296 w2367 w2494 w2652 w2748 w2825 w2882]
      tunnel: w267 -> [w320 w368 w418 w449 w562 w693 w891 w1105 w1304 w1449 w1504 w1560 w1613 w1662 w1704 w1747 w1799 w1912 w2070 w2146 w2206 w2280 w2352 w2485 w2645 w2750 w2826 w2884]
      tunnel: [w324 w372 w410 w455 w560 w691 w889 w1103 w1302 w1442 w1497 w1555 w1609 w1659 w1700 w1751 w1818 w1905 w2043 w2137 w2199 w2273 w2345 w2443 w2610 w2746 w2823 w2878] -> w266
      tunnel: [w323 w371 w409 w454 w559 w690 w888 w1102 w1301 w1443 w1498 w1556 w1610 w1660 w1701 w1750 w1788 w1913 w2044 w2136 w2207 w2281 w2353 w2442 w2609 w2744 w2821 w2879] -> w183
      tunnel: [w322 w370 w420 w452 w522 w692 w890 w1104 w1303 w1444 w1499 w1553 w1607 w1657 w1698 w1749 w1813 w1904 w2061 w2144 w2198 w2272 w2344 w2483 w2643 w2747 w2824 w2881] -> w78
      tunnel: [w321 w369 w419 w451 w563 w694 w892 w1106 w1305 w1450 w1505 w1561 w1614 w1663 w1705 w1748 w1798 w1932 w2089 w2147 w2222 w2296 w2367 w2494 w2652 w2748 w2825 w2882] -> w265
      tunnel: [w320 w368 w418 w449 w562 w693 w891 w1105 w1304 w1449 w1504 w1560 w1613 w1662 w1704 w1747 w1799 w1912 w2070 w2146 w2206 w2280 w2352 w2485 w2645 w2750 w2826 w2884] -> w264
      tunnel: [w325 w373 w421 w457 w565 w696 w894 w1108 w1307 w1441 w1496 w1554 w1608 w1658 w1699 w1746 w1816 w1856 w2069 w2135 w2205 w2279 w2351 w2484 w2644 w2742 w2819 w2876] -> w87
      tunnel: w263 -> [_ _ _ _ w569 w698 w898 w1110 w1311 _ _ _ _ _ _ _ _ w1909 w2066 _ w2204 w2278 w2350 w2462 w2626 _ _ _]
      tunnel: "Gate" -> [_ _ _ _ w553 w676 w875 w1088 w1288 _ _ _ _ _ _ _ _ _ _ _ _ _ _ _ _ _ _ _]
      tunnel: "Drain 2" -> [_ _ _ _ w552 w675 w874 w1087 w1287 _ _ _ _ _ _ _ _ _ _ _ _ _ _ _ _ _ _ _]
      tunnel: "Panel Controls" -> [_ _ _ _ _ _ w873 w1008 w1286 _ _ _ _ _ _ _ _ _ _ _ _ _ _ _ _ _ _ _]
      tunnel: w259 -> [w319 w367 w417 w448 w543 w660 w858 w1072 w1272 w1448 w1503 _ w1606 w1656 w1697 w1745 w1800 w1900 w2057 w2140 w2194 w2268 w2340 w2479 w2639 w2751 w2827 w2885]
      tunnel: w258 -> [w318 w366 w416 w447 w542 w659 w857 w1071 w1271 w1447 w1502 w1559 _ w1647 w1703 w1744 w1801 w1901 w2058 w2141 w2195 w2269 w2341 w2480 w2640 w2752 w2828 w2886]
      tunnel: w257 -> [w317 w365 w415 w446 w541 w658 w856 w1070 w1270 w1446 w1501 w1558 w1612 w1661 _ w1743 w1802 w1902 w2059 w2142 w2196 w2270 w2342 w2481 w2641 w2753 w2829 w2887]
      tunnel: w256 -> [w316 w364 w414 w445 w540 w657 w855 w1069 w1273 w1445 w1500 w1557 w1611 _ w1702 w1742 w1803 w1903 w2060 w2143 w2197 w2271 w2343 w2482 w2642 w2754 w2830 w2888]
      tunnel: [w319 w367 w417 w448 w543 w660 w858 w1072 w1272 w1448 w1503 w1552 w1606 w1656 w1697 w1745 w1800 w1900 w2057 w2140 w2194 w2268 w2340 w2479 w2639 w2751 w2827 w2885] -> w255
      tunnel: [w318 w366 w416 w447 w542 w659 w857 w1071 w1271 w1447 w1502 w1559 w1598 w1647 w1703 w1744 w1801 w1901 w2058 w2141 w2195 w2269 w2341 w2480 w2640 w2752 w2828 w2886] -> w254
      tunnel: [w317 w365 w415 w446 w541 w658 w856 w1070 w1270 w1446 w1501 w1558 w1612 w1661 w1696 w1743 w1802 w1902 w2059 w2142 w2196 w2270 w2342 w2481 w2641 w2753 w2829 w2887] -> w253
      tunnel: [w316 w364 w414 w445 w540 w657 w855 w1069 w1273 w1445 w1500 w1557 w1611 w1648 w1702 w1742 w1803 w1903 w2060 w2143 w2197 w2271 w2343 w2482 w2642 w2754 w2830 w2888] -> w252
      tunnel: w251 -> [w294 w339 w386 _ w489 w593 w837 w1005 w1254 w1415 w1473 w1530 w1576 w1625 w1674 w1720 w1760 w1877 w2018 w2113 w2159 w2237 w2310 w2423 w2586 w2705 w2766 w2872]
      tunnel: w250 -> [_ _ _ _ w537 w651 _ _ _ _ _ _ _ _ _ _ _ _ _ _ _ _ _ _ _ _ _ _]
      tunnel: [w315 w360 w407 w462 w514 w608 w808 w1021 w1231 w1440 w1494 w1551 w1597 w1646 w1695 w1741 w1784 w1866 w2023 w2134 w2183 w2261 w2334 w2398 w2567 w2743 w2820 w2893] -> w128
      tunnel: w249 -> [w315 w360 w407 w462 w514 w648 w815 w1061 w1197 w1440 w1494 w1551 w1597 w1646 w1695 w1741 w1784 w1873 w2023 w2134 w2183 w2261 w2334 w2404 w2571 w2743 w2820 w2893]
      tunnel: w109 -> [_ _ _ _ w511 w647 w848 w1060 w1264 _ _ _ _ _ _ _ w1782 w1893 w2040 _ w2180 w2258 w2331 w2439 w2601 _ _ _]
      tunnel: w247 -> [_ _ _ _ w510 w644 w846 w1057 w1263 _ _ _ _ _ _ _ w1780 w1891 w2039 _ w2179 w2257 w2330 w2438 w2602 _ w2793 _]
      tunnel: w110 -> [_ _ _ _ _ w640 w827 w1053 w1240 _ _ _ _ _ _ _ _ _ _ _ _ _ _ _ _ _ w2796 _]
      tunnel: [w314 w359 w406 w450 w513 w612 w787 w1025 w1200 w1439 w1493 w1550 w1596 w1645 w1694 w1740 w1783 w1858 w2006 w2133 w2182 w2260 w2333 w2392 w2561 w2749 w2800 w2883] -> w186
      tunnel: w245 -> [w314 w359 w406 w450 w513 w643 w826 w1056 w1239 w1439 w1493 w1550 w1596 w1645 w1694 w1740 w1783 w1862 w2007 w2133 w2182 w2260 w2333 w2393 w2562 w2749 w2800 w2883]
      tunnel: [w313 w358 w405 w461 w509 w607 w809 w1020 w1232 w1438 w1492 w1549 w1595 w1644 w1693 w1739 w1779 w1865 w2022 w2132 w2178 w2256 w2329 w2397 w2566 w2738 w2816 w2892] -> w127
      tunnel: w221 -> [w313 w358 w405 w461 w509 w639 w814 w1052 w1230 w1438 w1492 w1549 w1595 w1644 w1693 w1739 w1779 w1872 w2022 w2132 w2178 w2256 w2329 w2403 w2570 w2738 w2816 w2892]
      tunnel: [w312 w357 w404 w444 w508 w632 w845 w1045 w1262 w1437 w1491 w1548 w1594 w1643 w1692 w1738 w1778 w1890 w2038 w2131 w2177 w2255 w2328 w2437 w2600 w2737 w2815 w2889] -> w159
      tunnel: w208 -> [w312 w357 w404 w444 w508 w632 w845 w1045 w1262 w1437 w1491 w1548 w1594 w1643 w1692 w1738 w1778 w1890 w2038 w2131 w2177 w2255 w2328 w2437 w2600 w2736 w2794 w2889]
      tunnel: [w311 w356 w403 w472 w507 w631 w844 w1044 w1261 w1436 w1490 w1547 w1593 w1642 w1691 w1737 w1777 w1889 w2037 w2130 w2176 w2254 w2327 w2436 w2599 w2722 w2802 w2903] -> w187
      tunnel: w203 -> [w311 w356 w403 w472 w507 w631 w844 w1044 w1261 w1436 w1490 w1547 w1593 w1642 w1691 w1737 w1777 w1889 w2037 w2130 w2176 w2254 w2327 w2436 w2599 w2722 w2801 w2903]
      tunnel: [w310 w355 w402 w474 w506 w630 w843 w1043 w1260 w1435 w1489 w1546 w1592 w1641 w1690 w1736 w1776 w1888 w2036 w2129 w2175 w2253 w2326 w2435 w2598 w2721 w2789 w2905] -> w169
      tunnel: w202 -> [w310 w355 w402 w474 w506 w630 w843 w1043 w1260 w1435 w1489 w1546 w1592 w1641 w1690 w1736 w1776 w1888 w2036 w2129 w2175 w2253 w2326 w2435 w2598 w2721 w2787 w2905]
      tunnel: [w309 w354 w401 w458 w505 w629 w842 w1042 w1259 w1434 w1488 w1545 w1591 w1640 w1689 w1735 w1775 w1887 w2035 w2128 w2174 w2252 w2325 w2434 w2597 w2720 w2786 w2877] -> w201
      tunnel: w200 -> [w309 w354 w401 w458 w505 w629 w842 w1042 w1259 w1434 w1488 w1545 w1591 w1640 w1689 w1735 w1775 w1887 w2035 w2128 w2174 w2252 w2325 w2434 w2597 w2720 w2797 w2877]
      tunnel: w110 -> [_ _ _ _ _ _ _ _ _ _ _ _ _ _ _ _ _ _ _ _ _ _ _ _ _ _ w2785 _]
      tunnel: w184 -> [w308 w353 w400 w473 w504 w628 w841 w1041 w1258 w1433 w1487 w1544 w1590 w1639 w1688 w1734 w1774 w1886 w2034 w2127 w2173 w2251 w2324 w2433 w2596 w2719 w2784 w2904]
      tunnel: [w308 w353 w400 w473 w504 w628 w841 w1041 w1258 w1433 w1487 w1544 w1590 w1639 w1688 w1734 w1774 w1886 w2034 w2127 w2173 w2251 w2324 w2433 w2596 w2719 w2783 w2904] -> w164
      tunnel: [w307 w352 w399 w471 w503 w627 w840 w1040 w1257 w1432 w1486 w1543 w1589 w1638 w1687 w1733 w1773 w1885 w2033 w2126 w2172 w2250 w2323 w2432 w2595 w2718 w2782 w2902] -> w163
      tunnel: w168 -> [w307 w352 w399 w471 w503 w627 w840 w1040 w1257 w1432 w1486 w1543 w1589 w1638 w1687 w1733 w1773 w1885 w2033 w2126 w2172 w2250 w2323 w2432 w2595 w2718 w2781 w2902]
      tunnel: [w306 w351 w398 w453 w502 w626 w839 w1039 w1256 w1431 w1485 w1542 w1588 w1637 w1686 w1732 w1772 w1884 w2032 w2125 w2171 w2249 w2322 w2431 w2594 w2717 w2779 w2880] -> w160
      tunnel: w162 -> [w306 w351 w398 w453 w502 w626 w839 w1039 w1256 w1431 w1485 w1542 w1588 w1637 w1686 w1732 w1772 w1884 w2032 w2125 w2171 w2249 w2322 w2431 w2594 w2717 w2778 w2880]
      tunnel: [w304 w349 w396 w467 w499 w601 w803 w1014 w1217 w1429 w1484 w1541 w1586 w1635 w1684 w1730 w1770 w1883 w2031 w2124 w2170 w2248 w2320 w2430 w2593 w2716 w2777 w2898] -> w121
      tunnel: w149 -> [w304 w349 w396 w467 w499 w625 w820 w1038 w1220 w1429 w1484 w1541 w1586 w1635 w1684 w1730 w1770 w1883 w2031 w2124 w2170 w2248 w2320 w2430 w2593 w2716 w2777 w2898]
      tunnel: [w305 w350 w397 w468 w500 w602 w802 w1015 w1216 w1430 w1483 w1540 w1587 w1636 w1685 w1731 w1771 w1882 w2030 w2123 w2169 w2247 w2321 w2429 w2592 w2715 w2776 w2899] -> w122
      tunnel: w148 -> [w305 w350 w397 w468 w500 w624 w821 w1037 w1221 w1430 w1483 w1540 w1587 w1636 w1685 w1731 w1771 w1882 w2030 w2123 w2169 w2247 w2321 w2429 w2592 w2715 w2776 w2899]
      tunnel: [w297 w342 w389 w460 w496 w606 w810 w1019 w1233 w1422 w1481 w1538 w1584 w1633 w1682 w1728 w1763 w1864 w2021 w2122 w2162 w2240 w2313 w2396 w2565 w2708 w2775 w2891] -> w126
      tunnel: w137 -> [w297 w342 w389 w460 w496 w620 w813 w1033 w1236 w1422 w1481 w1538 w1584 w1633 w1682 w1728 w1763 w1871 w2021 w2122 w2162 w2240 w2313 w2402 w2569 w2708 w2775 w2891]
      tunnel: [w296 w341 w388 w459 w497 w605 w811 w1018 w1234 w1421 w1482 w1539 w1585 w1634 w1683 w1729 w1762 w1863 w2020 w2121 w2161 w2239 w2312 w2395 w2564 w2707 w2774 w2890] -> w125
      tunnel: w136 -> [w296 w341 w388 w459 w497 w619 w812 w1032 w1235 w1421 w1482 w1539 w1585 w1634 w1683 w1729 w1762 w1870 w2020 w2121 w2161 w2239 w2312 w2401 w2568 w2707 w2774 w2890]
      tunnel: [w299 w344 w391 w464 w495 w611 w806 w1024 w1227 w1427 w1479 w1536 w1582 w1631 w1680 w1726 w1765 w1868 w2025 w2116 w2164 w2242 w2315 w2400 w2574 w2712 w2772 w2895] -> w119
      tunnel: w135 -> [w299 w344 w391 w464 w495 w618 w817 w1031 w1228 w1427 w1479 w1536 w1582 w1631 w1680 w1726 w1765 w1875 w2025 w2116 w2164 w2242 w2315 w2406 w2575 w2712 w2772 w2895]
      tunnel: [w298 w343 w390 w463 w498 w609 w807 w1022 w1226 w1428 w1480 w1537 w1583 w1632 w1681 w1727 w1764 w1867 w2024 w2115 w2163 w2241 w2314 w2399 w2572 w2711 w2773 w2894] -> w129
      tunnel: w134 -> [w298 w343 w390 w463 w498 w617 w816 w1030 w1229 w1428 w1480 w1537 w1583 w1632 w1681 w1727 w1764 w1874 w2024 w2115 w2163 w2241 w2314 w2405 w2573 w2711 w2773 w2894]
      tunnel: [w301 w346 w393 w466 w494 w600 w805 w1013 w1225 w1425 w1477 w1534 w1580 w1629 w1678 w1724 w1767 w1879 w2027 w2118 w2166 w2244 w2317 w2426 w2589 w2714 w2770 w2897] -> w120
      tunnel: w133 -> [w301 w346 w393 w466 w494 w616 w819 w1029 w1222 w1425 w1477 w1534 w1580 w1629 w1678 w1724 w1767 w1879 w2027 w2118 w2166 w2244 w2317 w2426 w2589 w2714 w2770 w2897]
      tunnel: [w300 w345 w392 w465 w493 w599 w804 w1012 w1224 w1426 w1478 w1535 w1581 w1630 w1679 w1725 w1766 w1878 w2026 w2117 w2165 w2243 w2316 w2425 w2588 w2713 w2771 w2896] -> w118
      tunnel: w132 -> [w300 w345 w392 w465 w493 w615 w818 w1028 w1223 w1426 w1478 w1535 w1581 w1630 w1679 w1725 w1766 w1878 w2026 w2117 w2165 w2243 w2316 w2425 w2588 w2713 w2771 w2896]
      tunnel: [w303 w348 w395 w470 w492 w604 w800 w1017 w1214 w1423 w1475 w1532 w1578 w1627 w1676 w1722 w1769 w1881 w2029 w2120 w2168 w2246 w2319 w2428 w2591 w2710 w2768 w2901] -> w124
      tunnel: w131 -> [w303 w348 w395 w470 w492 w614 w823 w1027 w1218 w1423 w1475 w1532 w1578 w1627 w1676 w1722 w1769 w1881 w2029 w2120 w2168 w2246 w2319 w2428 w2591 w2710 w2768 w2901]
      tunnel: [w302 w347 w394 w469 w491 w603 w801 w1016 w1215 w1424 w1476 w1533 w1579 w1628 w1677 w1723 w1768 w1880 w2028 w2119 w2167 w2245 w2318 w2427 w2590 w2709 w2769 w2900] -> w123
      tunnel: w130 -> [w302 w347 w394 w469 w491 w613 w822 w1026 w1219 w1424 w1476 w1533 w1579 w1628 w1677 w1723 w1768 w1880 w2028 w2119 w2167 w2245 w2318 w2427 w2590 w2709 w2769 w2900]
      tunnel: w113 -> [w295 w340 w387 w456 w490 w596 w838 w1009 w1255 w1420 w1474 w1531 w1577 w1626 w1675 w1721 w1761 w1855 w2019 w2114 w2160 w2238 w2311 w2424 w2587 w2706 w2767 _]
      tunnel: [w295 w340 w387 w456 w490 w596 w838 w1009 w1255 w1420 w1474 w1531 w1577 w1626 w1675 w1721 w1761 w1855 w2019 w2114 w2160 w2238 w2311 w2424 w2587 w2706 w2767 w2873] -> w86
      tunnel: [w294 w339 w386 w434 w489 w593 w837 w1005 w1254 w1415 w1473 w1530 w1576 w1625 w1674 w1720 w1760 w1877 w2018 w2113 w2159 w2237 w2310 w2423 w2586 w2705 w2766 w2872] -> w79
      tunnel: w109 -> [_ _ _ _ _ _ _ _ _ _ _ _ _ _ _ _ _ w1825 w2002 _ _ _ _ w2408 w2578 _ _ _]
      tunnel: [w293 w338 w385 w433 w488 w592 w795 w1004 w1206 w1414 w1472 w1529 w1575 w1624 w1673 w1719 w1759 w1839 w2017 w2112 w2158 w2236 w2309 w2413 w2582 w2704 w2765 w2871] -> w82
      tunnel: [w292 w337 w384 w432 w487 w591 w796 w1003 w1207 w1413 w1471 w1528 w1574 w1623 w1672 w1718 w1758 w1838 w2016 w2111 w2157 w2235 w2308 w2374 w2543 w2703 w2764 w2870] -> w83
      tunnel: [w291 w336 w383 w431 w486 w590 w797 w1002 w1208 w1412 w1470 w1527 w1573 w1622 w1671 w1717 w1757 w1840 w1989 w2110 w2156 w2234 w2307 w2386 w2555 w2702 w2763 w2869] -> w84
      tunnel: [w290 w335 w382 w430 w485 w589 w798 w1001 w1209 w1411 w1469 w1526 w1572 w1621 w1670 w1716 w1756 w1837 w1996 w2109 w2155 w2233 w2306 w2383 w2552 w2701 w2762 w2868] -> w85
      tunnel: w108 -> [w293 w338 w385 w433 w488 w592 w795 w1004 w1206 w1414 w1472 w1529 w1575 w1624 w1673 w1719 w1759 w1836 w2017 w2112 w2158 w2236 w2309 w2416 w2585 w2704 w2765 w2871]
      tunnel: w107 -> [w292 w337 w384 w432 w487 w591 w796 w1003 w1207 w1413 w1471 w1528 w1574 w1623 w1672 w1718 w1758 w1835 w2016 w2111 w2157 w2235 w2308 w2415 w2584 w2703 w2764 w2870]
      tunnel: w106 -> [w291 w336 w383 w431 w486 w590 w797 w1002 w1208 w1412 w1470 w1527 w1573 w1622 w1671 w1717 w1757 w1834 w1990 w2110 w2156 w2234 w2307 w2386 w2555 w2702 w2763 w2869]
      tunnel: w105 -> [w290 w335 w382 w430 w485 w589 w798 w1001 w1209 w1411 w1469 w1526 w1572 w1621 w1670 w1716 w1756 w1833 w1998 w2109 w2155 w2233 w2306 w2414 w2583 w2701 w2762 w2868]
      tunnel: "Standby" -> [_ _ _ _ w484 w588 _ w1000 _ _ _ _ _ _ _ _ _ w1831 w2015 _ _ _ _ w2422 _ _ _ _]
      tunnel: w76 -> [w289 w334 w381 w429 w478 w582 w793 w994 w1204 w1410 w1468 w1525 w1571 w1620 w1669 w1715 w1755 w1822 w2010 w2108 w2151 w2230 w2304 w2380 w2549 w2700 w2761 w2867]
      tunnel: [w289 w334 w381 w429 w478 w582 w793 w994 w1204 w1410 w1468 w1525 w1571 w1620 w1669 w1715 w1755 w1822 w2010 w2108 w2151 w2230 w2304 w2375 w2544 w2700 w2761 w2867] -> w73
      tunnel: w75 -> [w288 w333 w380 w428 w477 w583 w794 w995 w1205 w1409 w1467 w1524 w1570 w1619 w1668 w1714 w1754 w1821 w2009 w2107 w2150 w2229 w2303 w2379 w2548 w2699 w2760 w2866]
      tunnel: [w288 w333 w380 w428 w477 w583 w794 w995 w1205 w1409 w1467 w1524 w1570 w1619 w1668 w1714 w1754 w1821 w2009 w2107 w2150 w2229 w2303 w2378 w2547 w2699 w2760 w2866] -> w74
      tunnel: w71 -> [w286 w331 w378 w426 w476 w581 w792 w993 w1203 w1408 w1466 w1523 w1569 w1617 w1666 w1712 w1752 w1819 w1995 w2105 w2148 w2227 w2301 w2372 w2541 w2697 w2755 w2864]
      tunnel: w70 -> [w287 w332 w379 w427 w475 w580 w791 w992 w1202 w1407 w1465 w1522 w1568 w1618 w1667 w1713 w1753 w1820 w1993 w2106 w2149 w2228 w2302 w2373 w2542 w2698 w2756 w2865]
      tunnel: [w287 w332 w379 w427 w475 w580 w791 w992 w1202 w1407 w1465 w1522 w1568 w1618 w1667 w1713 w1753 w1820 w1987 w2106 w2149 w2228 w2302 w2373 w2542 w2698 w2756 w2865] -> w69
      tunnel: [w286 w331 w378 w426 w476 w581 w792 w993 w1203 w1408 w1466 w1523 w1569 w1617 w1666 w1712 w1752 w1819 w1994 w2105 w2148 w2227 w2301 w2372 w2541 w2697 w2755 w2864] -> w68
      frame "wait" {
        n35 = Index Array(array=w330, index=0 ("Index")) -> (element=w328:string)
        n36 = Decimal String To Number(string=w328, default (0L)=u32 0) -> (number=w327:u32)  [unwired: 1 in, 1 out]
        n37 = Wait (ms)(milliseconds to wait=w327) -> ()  [unwired: 1 out]
      }
      frame "wait-min" {
        n38 = Index Array(array=w377, index=0 ("Index")) -> (element=w375:string)
        n39 = Decimal String To Number(string=w375, default (0L)=u32 0) -> (number=w363:u32)  [unwired: 1 in, 1 out]
        n40 = Multiply(x=w363, y=u32 60000) -> (x*y=w362:u32)
        n41 = Wait (ms)(milliseconds to wait=w362) -> ()  [unwired: 1 out]
      }
      frame "standby" {
        n42 = Index Array(array=w423, index=0 ("Index")) -> (element=w413:string)
        n43 = case shown="\"off\", Default" w413 {
          tunnel: [":PAGE:SCON:STAN 0" ":PAGE:SCON:STAN 1"] -> w408
          frame "off", Default {
          }
          frame "on" {
          }
        }
        n44 = VISA Write(VISA resource name=w412, write buffer=w408, error in (no error)=w411) -> (VISA resource name out=w410:refnum<visa-resource-name>, error out=w409:errorcluster)  [unwired: 1 out]
      }
      frame "Probe4" {
        n45 = Delete From Array(array=w435, index=0) -> (deleted portion=w438:string, array with subset deleted=w441:string[])  [unwired: 1 in]
        n46 = Equal?(x=w438, y="ON") -> (x = y?=w436:bool)
        n47 = Delete From Array(array=w441, index=0) -> (deleted portion=w440:string)  [unwired: 1 in, 1 out]
        n48 = Fract/Exp String To Number(string=w440) -> (number=w437:dbl)  [unwired: 3 in, 1 out]
        n49 = Bundle(w436, w437) -> (w434:cluster{bool, dbl})  [unwired: 1 in]
      }
      frame "pulsedstressV" {
        w520 = 0
        n50 = local read "Pulsed Stress V - Source/Common"() -> (w483:u32)
        n51 = local read "Pulsed Stress V - Probe 4"() -> (w480:u32)
        n52 = Number To Decimal String(number=w511) -> (decimal integer string=w566:string)  [unwired: 1 in]
        n53 = local read "Pulsed Stress V - Vextra"() -> (w479:u32)
        n54 = local read "Pulsed Stress V - Drain"() -> (w482:u32)
        n55 = local read "Pulsed Stress V - Gate"() -> (w481:u32)
        n56 = Delete From Array(array=w501, index=0 ("Index")) -> (deleted portion=w557:string, array with subset deleted=w556:string[])  [unwired: 1 in]
        n57 = Bundle By Name(cluster=w537, "Emergency Stop"=w569) -> (w538:T2)
        n58 = VISA Write(VISA resource name=w550, write buffer=":PAGE:CHAN:MODE SWE;" ("write buffer (\"\")"), error in (no error)=w549) -> (VISA resource name out=w547:refnum<visa-resource-name>, error out=w548:errorcluster)  [unwired: 1 out]
        n59 = Concatenate Strings(w565, "-pulsedstressV-" ("Substring"), w566, w510, ".txt" ("Substring")) -> (w568:string)
        n60 = case shown="\"d\", Default" w557 {
          tunnel: [w578 w579] -> w555
          frame "s" {
            w578 = u16 0 items=["Single", "Double"] ("sweep mode")
          }
          frame "d", Default {
            w579 = u16 1 items=["Single", "Double"] ("sweep mode")
          }
        }
        n61 = Fract/Exp String To Number(string=w556) -> (number=w551:dbl[])  [unwired: 3 in, 1 out]
        n62 = String To Path(string=w568) -> (path=w564:path)
        n63 = Index Array(array=w551, index #1=0 ("Index")) -> (element #1=w529:dbl, element #2=w528:dbl, element #3=w525:dbl, element #4=w524:dbl, element #5=w523:dbl, element #6=w527:dbl)  [unwired: 5 in]
        n64 = Bundle By Name(cluster=w526, "Pulse period"=w524, "Base voltage"=w525, "Pulse width"=w523) -> (w522:T5)
        n65 = Unbundle By Name(w522) -> ("Pulse period"=w530:dbl)
        n66 = Bundle By Name(cluster=w553, "Gate Start"=w528, "Gate Stop"=w529, "Gate Step (linear only)"=0, "Gate Compliance"=w562, "Range mode"=w543, "Range"=w542) -> (w544:T6)
        n67 = call <vilib>:"compatOverwrite.vi"("overwrite (F)"=TRUE) -> ("overwrite?"=w515:T8)
        n68 = Bundle By Name(cluster=w552, "Drain Start"=w527, "Drain Stop"=w520, "Drain Step"=w520, "Drain Compliance"=w563, "Range mode"=w541, "Range"=w540) -> (w545:T7)
        n69 = call "4155C PulsedStressV v3.0.vi"("VISA resource name in"=w547, "Gate"=w544, "Pulsed Stress V - Source/Common"=w483, "Drain"=w545, "Timings"=w522, "error in (no error)"=w548, "sweep mode"=w555, "Probe 4"=w489, "Pulsed Stress V - Drain"=w482, "Pulsed Stress V - Gate"=w481, "Panel Controls"=w538, "Standby"=w484, "Pulsed Stress V - Probe 4"=w480, "Pulsed Stress V - Vextra"=w479) -> ("Outparams"=w539:T9, "VISA Resource Name out"=w560:refnum<visa-resource-name>, "ID"=w518:dbl[], "IG"=w516:dbl[], "error out"=w561:errorcluster)  [unwired: 1 in]
        n70 = Unbundle By Name(w539) -> ("Number of points"=w517:i32)  [unwired: 2 out]
        n71 = for {
          N: w517 -> [_]
          tunnel: [w575] -> w519 mode=indexing
          tunnel: w530 -> [w577]
          i -> [w576]
          n72 = Multiply(x=w577, y=w576) -> (x*y=w575:dbl)
        }
        n73 = Insert Into Array(array=dbl[][] [] ("Input Array"), new element=w519) -> (w531:dbl[][])  [unwired: 2 in]
        n74 = Insert Into Array(array=w531, new element=w518) -> (w536:dbl[][])  [unwired: 2 in]
        n75 = Insert Into Array(array=w536, new element=w516) -> (w535:dbl[][])  [unwired: 2 in]
        n76 = Transpose 2D Array(2D array=w535) -> (transposed array=w534:dbl[][])
        n77 = Open/Create/Replace File(file path (use dialog)=w564, error in=w561, operation (0:open)=w515) -> (refnum out=w572:refnum<file>, error out=w573:errorcluster)  [unwired: 3 in, 1 out]
        n78 = call "4155C Write array to file.vi"("Byte Stream File Refnum"=w572, "Header"=string[] ["Time /s", "Id /A", "Ig /A"], "Data Array"=w534, "error in (no error)"=w573) -> ("dup refnum"=w570:refnum<file>, "error out"=w571:errorcluster)  [unwired: 1 in]
        n79 = Close File(refnum=w570, error in=w571) -> (error out=w559:errorcluster)  [unwired: 1 out]
      }
      frame "transfer" {
        # "Is off"
        # "Is on"
        # "Ig off"
        # "Ig on"
        # "Is min"
        # "Is max"
        # "Ig min"
        # "Ig max"
        # "Id min"
        # "Id max"
        # "Id off"
        # "Id on"
        n80 = Delete From Array(array=w689, index=0 ("Index")) -> (deleted portion=w687:string, array with subset deleted=w686:string[])  [unwired: 1 in]
        n81 = Bundle By Name(cluster=w651, "Emergency Stop"=w698) -> (w652:T2)
        n82 = local read "Transfer/Output - Source/Common"() -> (w587:u32)
        n83 = Number To Decimal String(number=w647) -> (decimal integer string=w646:string)  [unwired: 1 in]
        n84 = case shown="\"d\", Default" w687 {
          tunnel: [w783 w784] -> w685
          frame "s" {
            w783 = u16 0 items=["Single", "Double"] ("sweep mode")
          }
          frame "d", Default {
            w784 = u16 1 items=["Single", "Double"] ("sweep mode")
          }
        }
        n85 = Fract/Exp String To Number(string=w686) -> (number=w671:dbl[])  [unwired: 3 in, 1 out]
        n86 = Concatenate Strings(w696, w596, w646, w644, "_T_1_C_L.txt" ("Suffix (transfer)")) -> (w697:string)
        n87 = VISA Write(VISA resource name=w667, write buffer=":PAGE:CHAN:MODE SWE;" ("write buffer (\"\")"), error in (no error)=w666) -> (VISA resource name out=w664:refnum<visa-resource-name>, error out=w665:errorcluster)  [unwired: 1 out]
        n88 = local read "Plot transfer curve extrema vs time"() -> (w594:bool)
        n89 = local read "Transfer/Output - Gate"() -> (w585:u32)
        n90 = local read "Transfer/Output - Drain"() -> (w586:u32)
        n91 = String To Path(string=w697) -> (path=w695:path)
        n92 = local read "Transfer/Output - Probe 4"() -> (w584:u32)
        n93 = Index Array(array=w671, index #1=0 ("Index")) -> (element #1=w684:dbl, element #2=w683:dbl, element #3=w682:dbl)  [unwired: 2 in]
        n94 = Delete From Array(array=w671, length=3 ("Length"), index=0 ("Index")) -> (array with subset deleted=w669:dbl[])  [unwired: 1 out]
        n95 = case shown="True" w594 {
          tunnel: w643 -> [w700 w703]
          tunnel: w640 -> [_ w702]
          tunnel: [w700 w701] -> w612
          frame False {
          }
          frame True {
            n96 = Build Array (concatenate)(w703, w702) -> (w701:i32[])
          }
        }
        n97 = Bundle By Name(cluster=w676, "Gate Start"=w684, "Gate Stop"=w683, "Gate Step (linear only)"=w682, "Gate Compliance"=w693, "Range mode"=w660, "Range"=w659) -> (w661:T6)
        n98 = Index Array(array=w669, index #1=0 ("Index")) -> (element #1=w679:dbl, element #2=w678:dbl, element #3=w677:dbl)  [unwired: 2 in]
        n99 = call <vilib>:"compatOverwrite.vi"("overwrite (F)"=TRUE) -> ("overwrite?"=w650:T8)
        n100 = Bundle By Name(cluster=w675, "Drain Start"=w679, "Drain Stop"=w678, "Drain Step"=w677, "Drain Compliance"=w694, "Range mode"=w658, "Range"=w657) -> (w662:T7)
        n101 = call "4155C Transfer v3.0.vi"("VISA resource name in"=w664, "Source/Common"=w587, 2:"Gate"=w661, 3:"Drain"=w662, 4:"Drain"=w586, "Timings"=w692, "error in (no error)"=w665, 7:"Probe 4"=w593, 8:"Gate"=w585, 9:"Probe 4"=w584, "sweep mode"=w685, "Panel Controls"=w652, "Standby"=w588) -> ("VG"=w649:dbl[], "Outparams"=w656:T9, "VISA Resource Name out"=w691:refnum<visa-resource-name>, "IS"=w622:dbl[], "ID"=w623:dbl[], "IG"=w621:dbl[], "error out"=w641:errorcluster, "Probe 4"=w653:dbl[])  [unwired: 7 in]
        n102 = Unbundle By Name(w656) -> ("V2 Step"=w655:dbl, "V2 Start"=w654:dbl, "Number of points"=w610:i32)
        n103 = call "4155C Split array.vi"("Number of VAR2 steps"=w610, "Y2 data in"=w623, "X data in"=w649, "Y1 data in"=w622, "Y3 data in"=w621, "error in (no error)"=w641) -> ("Array of clusters"=w642:cluster{"Y data in":dbl[], "X data in":dbl[]}[], "error out"=w598:errorcluster)  [unwired: 1 in]
        n104 = case shown="True" "Plot transfer curve extrema vs time" {
          tunnel: w648 -> [w712 w782]
          tunnel: w639 -> [w713 w777]
          tunnel: w625 -> [w706 w773]
          tunnel: w624 -> [w707 w772]
          tunnel: w623 -> [_ w769]
          tunnel: w622 -> [_ w767]
          tunnel: w621 -> [_ w766]
          tunnel: w620 -> [w714 w762]
          tunnel: w619 -> [w715 w761]
          tunnel: w618 -> [w710 w758]
          tunnel: w617 -> [w711 w757]
          tunnel: w616 -> [w705 w754]
          tunnel: w615 -> [w704 w753]
          tunnel: w614 -> [w709 w750]
          tunnel: w613 -> [w708 w749]
          tunnel: w612 -> [_ w742]
          tunnel: [w710 w737] -> w611
          tunnel: w610 -> [_ w736]
          tunnel: [w711 w735] -> w609
          tunnel: [w712 w734] -> w608
          tunnel: [w713 w733] -> w607
          tunnel: [w714 w732] -> w606
          tunnel: [w715 w731] -> w605
          tunnel: [w709 w730] -> w604
          tunnel: [w708 w729] -> w603
          tunnel: [w707 w728] -> w602
          tunnel: [w706 w727] -> w601
          tunnel: [w705 w726] -> w600
          tunnel: [w704 w725] -> w599
          tunnel: w598 -> [w716 w724]
          tunnel: [w716 w720] -> w597
          frame False {
          }
          frame True {
            # "Adjusts graph colors."
            # "Adjusts graph colors."
            # "Ion will be the middle element of the array. The calculation of the index is done only once, since Is, Id, and Ig have the same dimensions."
            # "abs(Ig)"
            # "abs(Is)"
            # "Y1: Is\nY2: Id\nY3: Ig"
            # "abs(Id)"
            # "Adjusts graph colors."
            # "Adjusts graph colors."
            # "Adjusts graph colors."
            n105 = Absolute Value(x=w767) -> (abs(x)=w752:dbl[])
            n106 = Absolute Value(x=w769) -> (abs(x)=w768:dbl[])
            n107 = Absolute Value(x=w766) -> (abs(x)=w755:dbl[])
            n108 = Array Size(array=w768) -> (size(s)=w776:i32)
            n109 = Divide(x=w776, y=2) -> (x/y=w719:dbl)
            n110 = Subtract(x=w719, y=1) -> (x-y=w718:dbl)
            n111 = Array Max & Min(array=w752) -> (max value=w759:dbl, min value=w760:dbl)  [unwired: 2 out]
            n112 = Array Max & Min(array=w768) -> (max value=w781:dbl, min value=w765:dbl)  [unwired: 2 out]
            n113 = Array Max & Min(array=w755) -> (max value=w764:dbl, min value=w763:dbl)  [unwired: 2 out]
            n114 = Index Array(array=w752, index=w718) -> (element=w743:dbl)
            n115 = Index Array(array=w752, index=0) -> (element=w744:dbl)
            n116 = Index Array(array=w768, index=w718) -> (element=w745:dbl)
            n117 = Index Array(array=w768, index=0) -> (element=w746:dbl)
            n118 = Index Array(array=w755, index=w718) -> (element=w748:dbl)
            n119 = Index Array(array=w755, index=0) -> (element=w747:dbl)
            n120 = local write "Ig max"(w764) -> ()
            n121 = local write "Ig min"(w763) -> ()
            n122 = local write "Is max"(w759) -> ()
            n123 = local write "Is min"(w760) -> ()
            n124 = local write "Id max"(w781) -> ()
            n125 = local write "Id min"(w765) -> ()
            n126 = Build Array (concatenate)(w758, w759) -> (w737:dbl[])
            n127 = Build Array (concatenate)(w757, w760) -> (w735:dbl[])
            n128 = local write "Is off"(w744) -> ()
            n129 = local write "Is on"(w743) -> ()
            n130 = Build Array (concatenate)(w782, w781) -> (w734:dbl[])
            n131 = Build Array (concatenate)(w777, w765) -> (w733:dbl[])
            n132 = Build Array (concatenate)(w762, w764) -> (w732:dbl[])
            n133 = Build Array (concatenate)(w761, w763) -> (w731:dbl[])
            n134 = Build Array (concatenate)(w750, w743) -> (w730:dbl[])
            n135 = Build Array (concatenate)(w749, w744) -> (w729:dbl[])
            n136 = Build Array (concatenate)(w772, w745) -> (w728:dbl[])
            n137 = Build Array (concatenate)(w773, w746) -> (w727:dbl[])
            n138 = Build Array (concatenate)(w754, w748) -> (w726:dbl[])
            n139 = Build Array (concatenate)(w753, w747) -> (w725:dbl[])
            n140 = local write "Ig off"(w747) -> ()
            n141 = local write "Ig on"(w748) -> ()
            n142 = local write "Id off"(w746) -> ()
            n143 = local write "Id on"(w745) -> ()
            n144 = control-ref of="Imax vs time"() -> (w771:refnum<vi>)
            n145 = control-ref of="Imin vs time"() -> (w770:refnum<vi>)
            n146 = control-ref of="Ion vs time"() -> (w739:refnum<vi>)
            n147 = control-ref of="Ioff vs time"() -> (w738:refnum<vi>)
            n148 = control-ref of="I vs Vg"() -> (w780:refnum<vi>)
            n149 = call "4155C Split array.vi"("Number of VAR2 steps"=w736, "Y2 data in"=w728, "X data in"=w742, "Y1 data in"=w730, "Y3 data in"=w726, "error in (no error)"=w724) -> ("Array of clusters"=w740:cluster{"Y data in":dbl[], "X data in":dbl[]}[], "error out"=w723:errorcluster)  [unwired: 1 in]
            n150 = call "4155C Split array.vi"("Number of VAR2 steps"=w736, "Y2 data in"=w727, "X data in"=w742, "Y1 data in"=w729, "Y3 data in"=w725, "error in (no error)"=w723) -> ("Array of clusters"=w741:cluster{"Y data in":dbl[], "X data in":dbl[]}[], "error out"=w722:errorcluster)  [unwired: 1 in]
            n151 = call "4155C Split array.vi"("Number of VAR2 steps"=w736, "Y2 data in"=w734, "X data in"=w742, "Y1 data in"=w737, "Y3 data in"=w732, "error in (no error)"=w722) -> ("Array of clusters"=w779:cluster{"Y data in":dbl[], "X data in":dbl[]}[], "error out"=w721:errorcluster)  [unwired: 1 in]
            n152 = call "4155C Split array.vi"("Number of VAR2 steps"=w736, "Y2 data in"=w733, "X data in"=w742, "Y1 data in"=w735, "Y3 data in"=w731, "error in (no error)"=w721) -> ("Array of clusters"=w778:cluster{"Y data in":dbl[], "X data in":dbl[]}[], "error out"=w720:errorcluster)  [unwired: 1 in]
            n153 = call "4155C Config Chart Colours.vi"("Numeric"=w736, "XY Graph 2"=w771) -> ()  [unwired: 6 in]
            n154 = call "4155C Config Chart Colours.vi"("Numeric"=w736, "XY Graph 2"=w770) -> ()  [unwired: 6 in]
            n155 = call "4155C Config Chart Colours.vi"("Numeric"=w736, "XY Graph 2"=w739) -> ()  [unwired: 6 in]
            n156 = call "4155C Config Chart Colours.vi"("Numeric"=w736, "XY Graph 2"=w738) -> ()  [unwired: 6 in]
            n157 = call "4155C Config Chart Colours.vi"("Numeric"=w736, "XY Graph 2"=w780) -> ()  [unwired: 6 in]
            n158 = local write "Imax vs time"(w779) -> ()
            n159 = local write "Imin vs time"(w778) -> ()
            n160 = local write "Ion vs time"(w740) -> ()
            n161 = local write "Ioff vs time"(w741) -> ()
          }
        }
        n162 = local write "I vs Vg"(w642) -> ()
        n163 = Open/Create/Replace File(file path (use dialog)=w695, error in=w597, operation (0:open)=w650) -> (refnum out=w637:refnum<file>, error out=w635:errorcluster)  [unwired: 3 in, 1 out]
        n164 = call "4155C Make Big 2d array.vi"("1D Var1"=w649, "1d IS"=w622, "1d ID"=w623, "1d IG"=w621, "1d SMU4"=w653, "SMU4"=w593, "VAR2 START"=w654, "Number of VAR2 steps"=w610, "VAR2 STEP"=w655, "VAR1 Name"="Vg", "Decimal places in header"=i8 1, "VAR2 Name"="Vd") -> ("Header array"=w638:string[], "Data array"=w636:dbl[][])  [unwired: 14 in]
        n165 = call "4155C Write array to file.vi"("Byte Stream File Refnum"=w637, "Header"=w638, "Data Array"=w636, "error in (no error)"=w635) -> ("dup refnum"=w634:refnum<file>, "error out"=w633:errorcluster)  [unwired: 1 in]
        n166 = Close File(refnum=w634, error in=w633) -> (error out=w690:errorcluster)  [unwired: 1 out]
      }
      frame "transfer-fpp" {
        # "Adjusts graph colors."
        # "Y1 = Y2 = ID\nY3 = IG"
        n167 = local read "Plot transfer curve extrema vs time"() -> (w799:bool)
        n168 = Number To Decimal String(number=w848) -> (decimal integer string=w895:string)  [unwired: 1 in]
        n169 = Bundle By Name(cluster=w873, "Emergency Stop"=w898) -> (w906:T1)
        n170 = Delete From Array(array=w824, index=0 ("Index")) -> (deleted portion=w886:string, array with subset deleted=w885:string[])  [unwired: 1 in]
        n171 = local read "Plot transfer curve extrema vs time"() -> (w825:bool)
        n172 = local read "FPP - Source"() -> (w836:u32)
        n173 = local read "FPP - Drain"() -> (w834:u32)
        n174 = local read "FPP - Gate"() -> (w835:u32)
        n175 = Concatenate Strings(w894, "-transferfpp-" ("Substring"), w895, w846, ".txt" ("Substring")) -> (w897:string)
        n176 = VISA Write(VISA resource name=w865, write buffer=":PAGE:CHAN:MODE SWE;" ("write buffer (\"\")"), error in (no error)=w864) -> (VISA resource name out=w862:refnum<visa-resource-name>, error out=w863:errorcluster)  [unwired: 1 out]
        n177 = case shown="\"d\", Default" w886 {
          tunnel: [w990 w991] -> w884
          frame "s" {
            w990 = u16 0 items=["Single", "Double"] ("sweep mode")
          }
          frame "d", Default {
            w991 = u16 1 items=["Single", "Double"] ("sweep mode")
          }
        }
        n178 = Fract/Exp String To Number(string=w885) -> (number=w869:dbl[])  [unwired: 3 in, 1 out]
        n179 = String To Path(string=w897) -> (path=w893:path)
        n180 = Index Array(array=w869, index #1=0 ("Index")) -> (element #1=w883:dbl, element #2=w882:dbl, element #3=w881:dbl)  [unwired: 2 in]
        n181 = Delete From Array(array=w869, length=3 ("Length"), index=0 ("Index")) -> (array with subset deleted=w867:dbl[])  [unwired: 1 out]
        n182 = local read "FPP - Probe 2"() -> (w832:u32)
        n183 = local read "FPP - Probe 1"() -> (w833:u32)
        n184 = case shown="True" w825 {
          tunnel: w826 -> [w986 w989]
          tunnel: w827 -> [_ w988]
          tunnel: [w986 w987] -> w787
          frame False {
          }
          frame True {
            n185 = Build Array (concatenate)(w989, w988) -> (w987:i32[])
          }
        }
        n186 = control-ref of="I vs Vg"() -> (w828:refnum<vi>)
        n187 = Bundle By Name(cluster=w875, "Gate Start"=w883, "Gate Stop"=w882, "Gate Step (linear only)"=w881, "Gate Compliance"=w891, "Range mode"=w858, "Range"=w857) -> (w859:T6)
        n188 = Index Array(array=w867, index #1=0 ("Index")) -> (element #1=w878:dbl, element #2=w877:dbl, element #3=w876:dbl)  [unwired: 2 in]
        n189 = call <vilib>:"compatOverwrite.vi"("overwrite (F)"=TRUE) -> ("overwrite?"=w849:T8)
        n190 = Bundle By Name(cluster=w874, "Drain Start"=w878, "Drain Stop"=w877, "Drain Step"=w876, "Drain Compliance"=w892, "Range mode"=w856, "Range"=w855) -> (w860:T7)
        n191 = call "4155C Transfer-FPP v3.0.vi"("VISA resource name in"=w862, "FPP - Source"=w836, "Gate"=w859, "Drain"=w860, "FPP - Drain"=w834, "Timings"=w890, "error in (no error)"=w863, "FPP - Gate"=w835, "FPP - Probe 1"=w833, "sweep mode"=w884, "FPP - Probe 2"=w832, "Panel Controls"=w906) -> ("VG"=w829:dbl[], "Outparams"=w854:T9, "VISA Resource Name out"=w889:refnum<visa-resource-name>, "Vprobe2"=w851:dbl[], "ID"=w785:dbl[], "IG"=w786:dbl[], "Vprobe1"=w850:dbl[], "error out"=w790:errorcluster)  [unwired: 8 in]
        n192 = Unbundle By Name(w854) -> ("V2 Step"=w853:dbl, "V2 Start"=w852:dbl, "Number of points"=w788:i32)
        n193 = case shown="True" w799 {
          tunnel: w815 -> [w915 w985]
          tunnel: w814 -> [w916 w980]
          tunnel: w820 -> [w909 w976]
          tunnel: w821 -> [w910 w975]
          tunnel: w785 -> [_ w972]
          tunnel: w785 -> [_ w970]
          tunnel: w786 -> [_ w969]
          tunnel: w813 -> [w917 w965]
          tunnel: w812 -> [w918 w964]
          tunnel: w817 -> [w913 w961]
          tunnel: w816 -> [w914 w960]
          tunnel: w819 -> [w908 w957]
          tunnel: w818 -> [w907 w956]
          tunnel: w823 -> [w912 w953]
          tunnel: w822 -> [w911 w952]
          tunnel: w787 -> [_ w945]
          tunnel: [w913 w940] -> w806
          tunnel: w788 -> [_ w939]
          tunnel: [w914 w938] -> w807
          tunnel: [w915 w937] -> w808
          tunnel: [w916 w936] -> w809
          tunnel: [w917 w935] -> w810
          tunnel: [w918 w934] -> w811
          tunnel: [w912 w933] -> w800
          tunnel: [w911 w932] -> w801
          tunnel: [w910 w931] -> w802
          tunnel: [w909 w930] -> w803
          tunnel: [w908 w929] -> w805
          tunnel: [w907 w928] -> w804
          tunnel: w790 -> [w919 w927]
          tunnel: [w919 w923] -> w789
          frame False {
          }
          frame True {
            # "Y1 = Y2 = ID\nY3 = IG"
            # "Adjusts graph colors."
            # "Adjusts graph colors."
            # "Ion will be the middle element of the array. The calculation of the index is done only once, since Is, Id, and Ig have the same dimensions."
            # "abs(Ig)"
            # "abs(Is)"
            # "abs(Id)"
            # "Adjusts graph colors."
            # "Adjusts graph colors."
            # "Adjusts graph colors."
            n194 = Absolute Value(x=w970) -> (abs(x)=w955:dbl[])
            n195 = Absolute Value(x=w972) -> (abs(x)=w971:dbl[])
            n196 = Absolute Value(x=w969) -> (abs(x)=w958:dbl[])
            n197 = Array Size(array=w971) -> (size(s)=w979:i32)
            n198 = Divide(x=w979, y=2) -> (x/y=w922:dbl)
            n199 = Subtract(x=w922, y=1) -> (x-y=w921:dbl)
            n200 = Array Max & Min(array=w955) -> (max value=w962:dbl, min value=w963:dbl)  [unwired: 2 out]
            n201 = Array Max & Min(array=w971) -> (max value=w984:dbl, min value=w968:dbl)  [unwired: 2 out]
            n202 = Array Max & Min(array=w958) -> (max value=w967:dbl, min value=w966:dbl)  [unwired: 2 out]
            n203 = Index Array(array=w955, index=w921) -> (element=w946:dbl)
            n204 = Index Array(array=w955, index=0) -> (element=w947:dbl)
            n205 = Index Array(array=w971, index=w921) -> (element=w948:dbl)
            n206 = Index Array(array=w971, index=0) -> (element=w949:dbl)
            n207 = Index Array(array=w958, index=w921) -> (element=w951:dbl)
            n208 = Index Array(array=w958, index=0) -> (element=w950:dbl)
            n209 = local write "Ig max"(w967) -> ()
            n210 = local write "Ig min"(w966) -> ()
            n211 = local write "Is max"(w962) -> ()
            n212 = local write "Is min"(w963) -> ()
            n213 = local write "Id max"(w984) -> ()
            n214 = local write "Id min"(w968) -> ()
            n215 = Build Array (concatenate)(w961, w962) -> (w940:dbl[])
            n216 = Build Array (concatenate)(w960, w963) -> (w938:dbl[])
            n217 = local write "Is off"(w947) -> ()
            n218 = local write "Is on"(w946) -> ()
            n219 = Build Array (concatenate)(w985, w984) -> (w937:dbl[])
            n220 = Build Array (concatenate)(w980, w968) -> (w936:dbl[])
            n221 = Build Array (concatenate)(w965, w967) -> (w935:dbl[])
            n222 = Build Array (concatenate)(w964, w966) -> (w934:dbl[])
            n223 = Build Array (concatenate)(w953, w946) -> (w933:dbl[])
            n224 = Build Array (concatenate)(w952, w947) -> (w932:dbl[])
            n225 = Build Array (concatenate)(w975, w948) -> (w931:dbl[])
            n226 = Build Array (concatenate)(w976, w949) -> (w930:dbl[])
            n227 = Build Array (concatenate)(w957, w951) -> (w929:dbl[])
            n228 = Build Array (concatenate)(w956, w950) -> (w928:dbl[])
            n229 = local write "Ig off"(w950) -> ()
            n230 = local write "Ig on"(w951) -> ()
            n231 = local write "Id off"(w949) -> ()
            n232 = local write "Id on"(w948) -> ()
            n233 = control-ref of="Imax vs time"() -> (w974:refnum<vi>)
            n234 = control-ref of="Imin vs time"() -> (w973:refnum<vi>)
            n235 = control-ref of="Ion vs time"() -> (w942:refnum<vi>)
            n236 = control-ref of="Ioff vs time"() -> (w941:refnum<vi>)
            n237 = control-ref of="I vs Vg"() -> (w983:refnum<vi>)
            n238 = call "4155C Split array.vi"("Number of VAR2 steps"=w939, "Y2 data in"=w931, "X data in"=w945, "Y1 data in"=w933, "Y3 data in"=w929, "error in (no error)"=w927) -> ("Array of clusters"=w943:cluster{"Y data in":dbl[], "X data in":dbl[]}[], "error out"=w926:errorcluster)  [unwired: 1 in]
            n239 = call "4155C Split array.vi"("Number of VAR2 steps"=w939, "Y2 data in"=w930, "X data in"=w945, "Y1 data in"=w932, "Y3 data in"=w928, "error in (no error)"=w926) -> ("Array of clusters"=w944:cluster{"Y data in":dbl[], "X data in":dbl[]}[], "error out"=w925:errorcluster)  [unwired: 1 in]
            n240 = call "4155C Split array.vi"("Number of VAR2 steps"=w939, "Y2 data in"=w937, "X data in"=w945, "Y1 data in"=w940, "Y3 data in"=w935, "error in (no error)"=w925) -> ("Array of clusters"=w982:cluster{"Y data in":dbl[], "X data in":dbl[]}[], "error out"=w924:errorcluster)  [unwired: 1 in]
            n241 = call "4155C Split array.vi"("Number of VAR2 steps"=w939, "Y2 data in"=w936, "X data in"=w945, "Y1 data in"=w938, "Y3 data in"=w934, "error in (no error)"=w924) -> ("Array of clusters"=w981:cluster{"Y data in":dbl[], "X data in":dbl[]}[], "error out"=w923:errorcluster)  [unwired: 1 in]
            n242 = call "4155C Config Chart Colours.vi"("Numeric"=w939, "XY Graph 2"=w974) -> ()  [unwired: 6 in]
            n243 = call "4155C Config Chart Colours.vi"("Numeric"=w939, "XY Graph 2"=w973) -> ()  [unwired: 6 in]
            n244 = call "4155C Config Chart Colours.vi"("Numeric"=w939, "XY Graph 2"=w942) -> ()  [unwired: 6 in]
            n245 = call "4155C Config Chart Colours.vi"("Numeric"=w939, "XY Graph 2"=w941) -> ()  [unwired: 6 in]
            n246 = call "4155C Config Chart Colours.vi"("Numeric"=w939, "XY Graph 2"=w983) -> ()  [unwired: 6 in]
            n247 = local write "Imax vs time"(w982) -> ()
            n248 = local write "Imin vs time"(w981) -> ()
            n249 = local write "Ion vs time"(w943) -> ()
            n250 = local write "Ioff vs time"(w944) -> ()
          }
        }
        n251 = call "4155C Split array.vi"("Number of VAR2 steps"=w788, "Y2 data in"=w785, "X data in"=w829, "Y1 data in"=w785, "Y3 data in"=w786, "error in (no error)"=w789) -> ("Array of clusters"=w831:cluster{"Y data in":dbl[], "X data in":dbl[]}[], "error out"=w830:errorcluster)  [unwired: 1 in]
        n252 = local write "I vs Vg"(w831) -> ()
        n253 = call "4155C Config Chart Colours.vi"("Numeric"=w788, "XY Graph 2"=w828) -> ()  [unwired: 6 in]
        n254 = Open/Create/Replace File(file path (use dialog)=w893, error in=w830, operation (0:open)=w849) -> (refnum out=w903:refnum<file>, error out=w904:errorcluster)  [unwired: 3 in, 1 out]
        n255 = call "4155C Make Big 2d array FPP.vi"("1D Var1"=w829, "1d ID"=w785, "1d Vp2"=w851, "1d IG"=w786, "1d Vp1"=w850, "VAR2 START"=w852, "Number of VAR2 steps"=w788, "VAR2 STEP"=w853, "VAR1 Name"="Vg", "Decimal places in header"=i8 1, "VAR2 Name"="Vd") -> ("Header array"=w899:string[], "Data array"=w900:dbl[][])  [unwired: 15 in]
        n256 = call "4155C Write array to file.vi"("Byte Stream File Refnum"=w903, "Header"=w899, "Data Array"=w900, "error in (no error)"=w904) -> ("dup refnum"=w901:refnum<file>, "error out"=w902:errorcluster)  [unwired: 1 in]
        n257 = Close File(refnum=w901, error in=w902) -> (error out=w888:errorcluster)  [unwired: 1 out]
      }
      frame "output" {
        n258 = local read "Transfer/Output - Probe 4"() -> (w996:u32)
        n259 = Delete From Array(array=w1101, index=0 ("Index")) -> (deleted portion=w1099:string, array with subset deleted=w1098:string[])  [unwired: 1 in]
        n260 = Bundle By Name(cluster=w1008, "Emergency Stop"=w1110) -> (w1064:T1)
        n261 = Number To Decimal String(number=w1060) -> (decimal integer string=w1059:string)  [unwired: 1 in]
        n262 = case shown="\"d\", Default" w1099 {
          tunnel: [w1195 w1196] -> w1097
          frame "s" {
            w1195 = u16 0 items=["Single", "Double"] ("sweep mode")
          }
          frame "d", Default {
            w1196 = u16 1 items=["Single", "Double"] ("sweep mode")
          }
        }
        n263 = Fract/Exp String To Number(string=w1098) -> (number=w1083:dbl[])  [unwired: 3 in, 1 out]
        n264 = Concatenate Strings(w1108, w1009, w1059, w1057, "_O_1_C_L.txt" ("Suffix (transfer)")) -> (w1109:string)
        n265 = local read "Transfer/Output - Drain"() -> (w998:u32)
        n266 = local read "Transfer/Output - Source/Common"() -> (w999:u32)
        n267 = VISA Write(VISA resource name=w1079, write buffer=":PAGE:CHAN:MODE SWE;" ("write buffer (\"\")"), error in (no error)=w1078) -> (VISA resource name out=w1076:refnum<visa-resource-name>, error out=w1077:errorcluster)  [unwired: 1 out]
        n268 = String To Path(string=w1109) -> (path=w1107:path)
        n269 = local read "Plot output curve extrema vs time"() -> (w1006:bool)
        n270 = Index Array(array=w1083, index #1=0 ("Index")) -> (element #1=w1096:dbl, element #2=w1095:dbl, element #3=w1094:dbl)  [unwired: 2 in]
        n271 = Delete From Array(array=w1083, length=3 ("Length"), index=0 ("Index")) -> (array with subset deleted=w1081:dbl[])  [unwired: 1 out]
        n272 = local read "Transfer/Output - Gate"() -> (w997:u32)
        n273 = case shown="True" w1006 {
          tunnel: w1056 -> [w1112 w1115]
          tunnel: w1053 -> [_ w1114]
          tunnel: [w1112 w1113] -> w1025
          frame False {
          }
          frame True {
            n274 = Build Array (concatenate)(w1115, w1114) -> (w1113:i32[])
          }
        }
        n275 = Bundle By Name(cluster=w1088, "Gate Start"=w1096, "Gate Stop"=w1095, "Gate Step (linear only)"=w1094, "Gate Compliance"=w1105, "Range mode"=w1072, "Range"=w1071) -> (w1073:T6)
        n276 = Index Array(array=w1081, index #1=0 ("Index")) -> (element #1=w1091:dbl, element #2=w1090:dbl, element #3=w1089:dbl)  [unwired: 2 in]
        n277 = call <vilib>:"compatOverwrite.vi"("overwrite (F)"=TRUE) -> ("overwrite?"=w1063:T8)
        n278 = Bundle By Name(cluster=w1087, "Drain Start"=w1091, "Drain Stop"=w1090, "Drain Step"=w1089, "Drain Compliance"=w1106, "Range mode"=w1070, "Range"=w1069) -> (w1074:T7)
        n279 = call "4155C Output v3.0.vi"("VISA resource name in"=w1076, "Source/Common"=w999, 2:"Gate"=w1073, 3:"Drain"=w1074, 4:"Drain"=w998, "Timings"=w1104, "error in (no error)"=w1077, 7:"Probe 4"=w1005, 8:"Gate"=w997, 9:"Probe 4"=w996, "sweep mode"=w1097, "Panel controls"=w1064, "Standby"=w1000) -> ("VD"=w1062:dbl[], "Outparams"=w1068:T9, "VISA Resource Name out"=w1103:refnum<visa-resource-name>, "IS"=w1035:dbl[], "ID"=w1036:dbl[], "IG"=w1034:dbl[], "error out"=w1054:errorcluster, "Probe 4"=w1065:dbl[])  [unwired: 7 in]
        n280 = Unbundle By Name(w1068) -> ("V2 Step"=w1067:dbl, "V2 Start"=w1066:dbl, "Number of points"=w1023:i32)
        n281 = call "4155C Split array.vi"("Number of VAR2 steps"=w1023, "Y2 data in"=w1036, "X data in"=w1062, "Y1 data in"=w1035, "Y3 data in"=w1034, "error in (no error)"=w1054) -> ("Array of clusters"=w1055:cluster{"Y data in":dbl[], "X data in":dbl[]}[], "error out"=w1011:errorcluster)  [unwired: 1 in]
        n282 = case shown="True" "Plot output curve extrema vs time" {
          tunnel: w1061 -> [w1119 w1194]
          tunnel: w1052 -> [w1118 w1189]
          tunnel: w1038 -> [w1124 w1185]
          tunnel: w1037 -> [w1125 w1184]
          tunnel: w1036 -> [_ w1181]
          tunnel: w1035 -> [_ w1179]
          tunnel: w1034 -> [_ w1178]
          tunnel: w1033 -> [w1117 w1174]
          tunnel: w1032 -> [w1116 w1173]
          tunnel: w1031 -> [w1121 w1170]
          tunnel: w1030 -> [w1120 w1169]
          tunnel: w1029 -> [w1123 w1166]
          tunnel: w1028 -> [w1122 w1165]
          tunnel: w1027 -> [w1127 w1162]
          tunnel: w1026 -> [w1126 w1161]
          tunnel: w1025 -> [_ w1154]
          tunnel: [w1121 w1149] -> w1024
          tunnel: w1023 -> [_ w1148]
          tunnel: [w1120 w1147] -> w1022
          tunnel: [w1119 w1146] -> w1021
          tunnel: [w1118 w1145] -> w1020
          tunnel: [w1117 w1144] -> w1019
          tunnel: [w1116 w1143] -> w1018
          tunnel: [w1127 w1142] -> w1017
          tunnel: [w1126 w1141] -> w1016
          tunnel: [w1125 w1140] -> w1015
          tunnel: [w1124 w1139] -> w1014
          tunnel: [w1123 w1138] -> w1013
          tunnel: [w1122 w1137] -> w1012
          tunnel: w1011 -> [w1128 w1136]
          tunnel: [w1128 w1132] -> w1010
          frame False {
          }
          frame True {
            # "Adjusts graph colors."
            # "Adjusts graph colors."
            # "Ion will be the middle element of the array. The calculation of the index is done only once, since Is, Id, and Ig have the same dimensions."
            # "abs(Ig)"
            # "abs(Is)"
            # "Y1: Is\nY2: Id\nY3: Ig"
            # "abs(Id)"
            # "Adjusts graph colors."
            # "Adjusts graph colors."
            # "Adjusts graph colors."
            n283 = Absolute Value(x=w1179) -> (abs(x)=w1164:dbl[])
            n284 = Absolute Value(x=w1181) -> (abs(x)=w1180:dbl[])
            n285 = Absolute Value(x=w1178) -> (abs(x)=w1167:dbl[])
            n286 = Array Size(array=w1180) -> (size(s)=w1188:i32)
            n287 = Divide(x=w1188, y=2) -> (x/y=w1131:dbl)
            n288 = Subtract(x=w1131, y=1) -> (x-y=w1130:dbl)
            n289 = Array Max & Min(array=w1164) -> (max value=w1171:dbl, min value=w1172:dbl)  [unwired: 2 out]
            n290 = Array Max & Min(array=w1180) -> (max value=w1193:dbl, min value=w1177:dbl)  [unwired: 2 out]
            n291 = Array Max & Min(array=w1167) -> (max value=w1176:dbl, min value=w1175:dbl)  [unwired: 2 out]
            n292 = Index Array(array=w1164, index=w1130) -> (element=w1155:dbl)
            n293 = Index Array(array=w1164, index=0) -> (element=w1156:dbl)
            n294 = Index Array(array=w1180, index=w1130) -> (element=w1157:dbl)
            n295 = Index Array(array=w1180, index=0) -> (element=w1158:dbl)
            n296 = Index Array(array=w1167, index=w1130) -> (element=w1160:dbl)
            n297 = Index Array(array=w1167, index=0) -> (element=w1159:dbl)
            n298 = local write "Ig max"(w1176) -> ()
            n299 = local write "Ig min"(w1175) -> ()
            n300 = local write "Is max"(w1171) -> ()
            n301 = local write "Is min"(w1172) -> ()
            n302 = local write "Id max"(w1193) -> ()
            n303 = local write "Id min"(w1177) -> ()
            n304 = Build Array (concatenate)(w1170, w1171) -> (w1149:dbl[])
            n305 = Build Array (concatenate)(w1169, w1172) -> (w1147:dbl[])
            n306 = local write "Is off"(w1156) -> ()
            n307 = local write "Is on"(w1155) -> ()
            n308 = Build Array (concatenate)(w1194, w1193) -> (w1146:dbl[])
            n309 = Build Array (concatenate)(w1189, w1177) -> (w1145:dbl[])
            n310 = Build Array (concatenate)(w1174, w1176) -> (w1144:dbl[])
            n311 = Build Array (concatenate)(w1173, w1175) -> (w1143:dbl[])
            n312 = Build Array (concatenate)(w1162, w1155) -> (w1142:dbl[])
            n313 = Build Array (concatenate)(w1161, w1156) -> (w1141:dbl[])
            n314 = Build Array (concatenate)(w1184, w1157) -> (w1140:dbl[])
            n315 = Build Array (concatenate)(w1185, w1158) -> (w1139:dbl[])
            n316 = Build Array (concatenate)(w1166, w1160) -> (w1138:dbl[])
            n317 = Build Array (concatenate)(w1165, w1159) -> (w1137:dbl[])
            n318 = local write "Ig off"(w1159) -> ()
            n319 = local write "Ig on"(w1160) -> ()
            n320 = local write "Id off"(w1158) -> ()
            n321 = local write "Id on"(w1157) -> ()
            n322 = control-ref of="Imax vs time"() -> (w1183:refnum<vi>)
            n323 = control-ref of="Imin vs time"() -> (w1182:refnum<vi>)
            n324 = control-ref of="Ion vs time"() -> (w1151:refnum<vi>)
            n325 = control-ref of="Ioff vs time"() -> (w1150:refnum<vi>)
            n326 = control-ref of="I vs Vg"() -> (w1192:refnum<vi>)
            n327 = call "4155C Split array.vi"("Number of VAR2 steps"=w1148, "Y2 data in"=w1140, "X data in"=w1154, "Y1 data in"=w1142, "Y3 data in"=w1138, "error in (no error)"=w1136) -> ("Array of clusters"=w1152:cluster{"Y data in":dbl[], "X data in":dbl[]}[], "error out"=w1135:errorcluster)  [unwired: 1 in]
            n328 = call "4155C Split array.vi"("Number of VAR2 steps"=w1148, "Y2 data in"=w1139, "X data in"=w1154, "Y1 data in"=w1141, "Y3 data in"=w1137, "error in (no error)"=w1135) -> ("Array of clusters"=w1153:cluster{"Y data in":dbl[], "X data in":dbl[]}[], "error out"=w1134:errorcluster)  [unwired: 1 in]
            n329 = call "4155C Split array.vi"("Number of VAR2 steps"=w1148, "Y2 data in"=w1146, "X data in"=w1154, "Y1 data in"=w1149, "Y3 data in"=w1144, "error in (no error)"=w1134) -> ("Array of clusters"=w1191:cluster{"Y data in":dbl[], "X data in":dbl[]}[], "error out"=w1133:errorcluster)  [unwired: 1 in]
            n330 = call "4155C Split array.vi"("Number of VAR2 steps"=w1148, "Y2 data in"=w1145, "X data in"=w1154, "Y1 data in"=w1147, "Y3 data in"=w1143, "error in (no error)"=w1133) -> ("Array of clusters"=w1190:cluster{"Y data in":dbl[], "X data in":dbl[]}[], "error out"=w1132:errorcluster)  [unwired: 1 in]
            n331 = call "4155C Config Chart Colours.vi"("Numeric"=w1148, "XY Graph 2"=w1183) -> ()  [unwired: 6 in]
            n332 = call "4155C Config Chart Colours.vi"("Numeric"=w1148, "XY Graph 2"=w1182) -> ()  [unwired: 6 in]
            n333 = call "4155C Config Chart Colours.vi"("Numeric"=w1148, "XY Graph 2"=w1151) -> ()  [unwired: 6 in]
            n334 = call "4155C Config Chart Colours.vi"("Numeric"=w1148, "XY Graph 2"=w1150) -> ()  [unwired: 6 in]
            n335 = call "4155C Config Chart Colours.vi"("Numeric"=w1148, "XY Graph 2"=w1192) -> ()  [unwired: 6 in]
            n336 = local write "Imax vs time"(w1191) -> ()
            n337 = local write "Imin vs time"(w1190) -> ()
            n338 = local write "Ion vs time"(w1152) -> ()
            n339 = local write "Ioff vs time"(w1153) -> ()
          }
        }
        n340 = local write "I vs Vd"(w1055) -> ()
        n341 = Open/Create/Replace File(file path (use dialog)=w1107, error in=w1010, operation (0:open)=w1063) -> (refnum out=w1050:refnum<file>, error out=w1048:errorcluster)  [unwired: 3 in, 1 out]
        n342 = call "4155C Make Big 2d array.vi"("1D Var1"=w1062, "1d IS"=w1035, "1d ID"=w1036, "1d IG"=w1034, "1d SMU4"=w1065, "SMU4"=w1005, "VAR2 START"=w1066, "Number of VAR2 steps"=w1023, "VAR2 STEP"=w1067, "VAR1 Name"="Vd", "Decimal places in header"=i8 1, "VAR2 Name"="Vg") -> ("Header array"=w1051:string[], "Data array"=w1049:dbl[][])  [unwired: 14 in]
        n343 = call "4155C Write array to file.vi"("Byte Stream File Refnum"=w1050, "Header"=w1051, "Data Array"=w1049, "error in (no error)"=w1048) -> ("dup refnum"=w1047:refnum<file>, "error out"=w1046:errorcluster)  [unwired: 1 in]
        n344 = Close File(refnum=w1047, error in=w1046) -> (error out=w1102:errorcluster)  [unwired: 1 out]
      }
      frame "output-fpp" {
        # "Y1 = Y2 = ID\nY3 = IG"
        # "Adjusts graph colors."
        # "Adjusts graph colors."
        # "Y1 = Vp2\nY2 = Y3 = Vp1"
        n345 = local read "Plot output curve extrema vs time"() -> (w1213:bool)
        n346 = local read "FPP - Gate"() -> (w1251:u32)
        n347 = local read "FPP - Probe 1"() -> (w1250:u32)
        n348 = local read "FPP - Probe 2"() -> (w1249:u32)
        n349 = Number To Decimal String(number=w1264) -> (decimal integer string=w1308:string)  [unwired: 1 in]
        n350 = Bundle By Name(cluster=w1286, "Emergency Stop"=w1311) -> (w1321:T1)
        n351 = local read "Plot output curve extrema vs time"() -> (w1238:bool)
        n352 = Delete From Array(array=w1237, index=0 ("Index")) -> (deleted portion=w1299:string, array with subset deleted=w1298:string[])  [unwired: 1 in]
        n353 = VISA Write(VISA resource name=w1277, write buffer=":PAGE:CHAN:MODE SWE;" ("write buffer (\"\")"), error in (no error)=w1274) -> (VISA resource name out=w1276:refnum<visa-resource-name>, error out=w1275:errorcluster)  [unwired: 1 out]
        n354 = Concatenate Strings(w1307, "-outputfpp-" ("Substring"), w1308, w1263, ".txt" ("Substring")) -> (w1310:string)
        n355 = case shown="\"d\", Default" w1299 {
          tunnel: [w1405 w1406] -> w1297
          frame "s" {
            w1405 = u16 0 items=["Single", "Double"] ("sweep mode")
          }
          frame "d", Default {
            w1406 = u16 1 items=["Single", "Double"] ("sweep mode")
          }
        }
        n356 = Fract/Exp String To Number(string=w1298) -> (number=w1280:dbl[])  [unwired: 3 in, 1 out]
        n357 = String To Path(string=w1310) -> (path=w1306:path)
        n358 = Index Array(array=w1280, index #1=0 ("Index")) -> (element #1=w1296:dbl, element #2=w1295:dbl, element #3=w1294:dbl)  [unwired: 2 in]
        n359 = Delete From Array(array=w1280, length=3 ("Length"), index=0 ("Index")) -> (array with subset deleted=w1279:dbl[])  [unwired: 1 out]
        n360 = local read "FPP - Source"() -> (w1253:u32)
        n361 = case shown="True" w1238 {
          tunnel: w1239 -> [w1401 w1404]
          tunnel: w1240 -> [_ w1403]
          tunnel: [w1401 w1402] -> w1200
          frame False {
          }
          frame True {
            n362 = Build Array (concatenate)(w1404, w1403) -> (w1402:i32[])
          }
        }
        n363 = local read "FPP - Drain"() -> (w1252:u32)
        n364 = Bundle By Name(cluster=w1288, "Gate Start"=w1296, "Gate Stop"=w1295, "Gate Step (linear only)"=w1294, "Gate Compliance"=w1304, "Range mode"=w1272, "Range"=w1271) -> (w1320:T6)
        n365 = Index Array(array=w1279, index #1=0 ("Index")) -> (element #1=w1291:dbl, element #2=w1290:dbl, element #3=w1289:dbl)  [unwired: 2 in]
        n366 = call <vilib>:"compatOverwrite.vi"("overwrite (F)"=TRUE) -> ("overwrite?"=w1266:T8)
        n367 = control-ref of="I vs Vd"() -> (w1242:refnum<vi>)
        n368 = control-ref of="Vp vs Vg (FPP)"() -> (w1241:refnum<vi>)
        n369 = Bundle By Name(cluster=w1287, "Drain Start"=w1291, "Drain Stop"=w1290, "Drain Step"=w1289, "Drain Compliance"=w1305, "Range mode"=w1270, "Range"=w1273) -> (w1319:T7)
        n370 = call "4155C Output-FPP v3.0.vi"("VISA resource name in"=w1276, "FPP - Source"=w1253, "Gate"=w1320, "Drain"=w1319, "FPP - Drain"=w1252, "Timings"=w1303, "error in (no error)"=w1275, "FPP - Gate"=w1251, "FPP - Probe 1"=w1250, "sweep mode"=w1297, "FPP - Probe 2"=w1249, "Panel controls"=w1321) -> ("VD"=w1245:dbl[], "Outparams"=w1268:T9, "VISA Resource Name out"=w1302:refnum<visa-resource-name>, "Vprobe2"=w1244:dbl[], "ID"=w1199:dbl[], "IG"=w1198:dbl[], "Vprobe1"=w1243:dbl[], "error out"=w1212:errorcluster)  [unwired: 8 in]
        n371 = Unbundle By Name(w1268) -> ("V2 Step"=w1269:dbl, "V2 Start"=w1267:dbl, "Number of points"=w1201:i32)
        n372 = case shown="True" w1213 {
          tunnel: w1197 -> [w1325 w1400]
          tunnel: w1230 -> [w1324 w1395]
          tunnel: w1220 -> [w1330 w1391]
          tunnel: w1221 -> [w1331 w1390]
          tunnel: w1199 -> [_ w1387]
          tunnel: w1199 -> [_ w1385]
          tunnel: w1198 -> [_ w1384]
          tunnel: w1236 -> [w1323 w1380]
          tunnel: w1235 -> [w1322 w1379]
          tunnel: w1228 -> [w1327 w1376]
          tunnel: w1229 -> [w1326 w1375]
          tunnel: w1222 -> [w1329 w1372]
          tunnel: w1223 -> [w1328 w1371]
          tunnel: w1218 -> [w1333 w1368]
          tunnel: w1219 -> [w1332 w1367]
          tunnel: w1200 -> [_ w1360]
          tunnel: [w1327 w1355] -> w1227
          tunnel: w1201 -> [_ w1354]
          tunnel: [w1326 w1353] -> w1226
          tunnel: [w1325 w1352] -> w1231
          tunnel: [w1324 w1351] -> w1232
          tunnel: [w1323 w1350] -> w1233
          tunnel: [w1322 w1349] -> w1234
          tunnel: [w1333 w1348] -> w1214
          tunnel: [w1332 w1347] -> w1215
          tunnel: [w1331 w1346] -> w1216
          tunnel: [w1330 w1345] -> w1217
          tunnel: [w1329 w1344] -> w1225
          tunnel: [w1328 w1343] -> w1224
          tunnel: w1212 -> [w1334 w1342]
          tunnel: [w1334 w1338] -> w1211
          frame False {
          }
          frame True {
            # "Y1 = Y2 = ID\nY3 = IG"
            # "Adjusts graph colors."
            # "Adjusts graph colors."
            # "Ion will be the middle element of the array. The calculation of the index is done only once, since Is, Id, and Ig have the same dimensions."
            # "abs(Ig)"
            # "abs(Is)"
            # "abs(Id)"
            # "Adjusts graph colors."
            # "Adjusts graph colors."
            # "Adjusts graph colors."
            n373 = Absolute Value(x=w1385) -> (abs(x)=w1370:dbl[])
            n374 = Absolute Value(x=w1387) -> (abs(x)=w1386:dbl[])
            n375 = Absolute Value(x=w1384) -> (abs(x)=w1373:dbl[])
            n376 = Array Size(array=w1386) -> (size(s)=w1394:i32)
            n377 = Divide(x=w1394, y=2) -> (x/y=w1337:dbl)
            n378 = Subtract(x=w1337, y=1) -> (x-y=w1336:dbl)
            n379 = Array Max & Min(array=w1370) -> (max value=w1377:dbl, min value=w1378:dbl)  [unwired: 2 out]
            n380 = Array Max & Min(array=w1386) -> (max value=w1399:dbl, min value=w1383:dbl)  [unwired: 2 out]
            n381 = Array Max & Min(array=w1373) -> (max value=w1382:dbl, min value=w1381:dbl)  [unwired: 2 out]
            n382 = Index Array(array=w1370, index=w1336) -> (element=w1361:dbl)
            n383 = Index Array(array=w1370, index=0) -> (element=w1362:dbl)
            n384 = Index Array(array=w1386, index=w1336) -> (element=w1363:dbl)
            n385 = Index Array(array=w1386, index=0) -> (element=w1364:dbl)
            n386 = Index Array(array=w1373, index=w1336) -> (element=w1366:dbl)
            n387 = Index Array(array=w1373, index=0) -> (element=w1365:dbl)
            n388 = local write "Ig max"(w1382) -> ()
            n389 = local write "Ig min"(w1381) -> ()
            n390 = local write "Is max"(w1377) -> ()
            n391 = local write "Is min"(w1378) -> ()
            n392 = local write "Id max"(w1399) -> ()
            n393 = local write "Id min"(w1383) -> ()
            n394 = Build Array (concatenate)(w1376, w1377) -> (w1355:dbl[])
            n395 = Build Array (concatenate)(w1375, w1378) -> (w1353:dbl[])
            n396 = local write "Is off"(w1362) -> ()
            n397 = local write "Is on"(w1361) -> ()
            n398 = Build Array (concatenate)(w1400, w1399) -> (w1352:dbl[])
            n399 = Build Array (concatenate)(w1395, w1383) -> (w1351:dbl[])
            n400 = Build Array (concatenate)(w1380, w1382) -> (w1350:dbl[])
            n401 = Build Array (concatenate)(w1379, w1381) -> (w1349:dbl[])
            n402 = Build Array (concatenate)(w1368, w1361) -> (w1348:dbl[])
            n403 = Build Array (concatenate)(w1367, w1362) -> (w1347:dbl[])
            n404 = Build Array (concatenate)(w1390, w1363) -> (w1346:dbl[])
            n405 = Build Array (concatenate)(w1391, w1364) -> (w1345:dbl[])
            n406 = Build Array (concatenate)(w1372, w1366) -> (w1344:dbl[])
            n407 = Build Array (concatenate)(w1371, w1365) -> (w1343:dbl[])
            n408 = local write "Ig off"(w1365) -> ()
            n409 = local write "Ig on"(w1366) -> ()
            n410 = local write "Id off"(w1364) -> ()
            n411 = local write "Id on"(w1363) -> ()
            n412 = control-ref of="Imax vs time"() -> (w1389:refnum<vi>)
            n413 = control-ref of="Imin vs time"() -> (w1388:refnum<vi>)
            n414 = control-ref of="Ion vs time"() -> (w1357:refnum<vi>)
            n415 = control-ref of="Ioff vs time"() -> (w1356:refnum<vi>)
            n416 = control-ref of="I vs Vg"() -> (w1398:refnum<vi>)
            n417 = call "4155C Split array.vi"("Number of VAR2 steps"=w1354, "Y2 data in"=w1346, "X data in"=w1360, "Y1 data in"=w1348, "Y3 data in"=w1344, "error in (no error)"=w1342) -> ("Array of clusters"=w1358:cluster{"Y data in":dbl[], "X data in":dbl[]}[], "error out"=w1341:errorcluster)  [unwired: 1 in]
            n418 = call "4155C Split array.vi"("Number of VAR2 steps"=w1354, "Y2 data in"=w1345, "X data in"=w1360, "Y1 data in"=w1347, "Y3 data in"=w1343, "error in (no error)"=w1341) -> ("Array of clusters"=w1359:cluster{"Y data in":dbl[], "X data in":dbl[]}[], "error out"=w1340:errorcluster)  [unwired: 1 in]
            n419 = call "4155C Split array.vi"("Number of VAR2 steps"=w1354, "Y2 data in"=w1352, "X data in"=w1360, "Y1 data in"=w1355, "Y3 data in"=w1350, "error in (no error)"=w1340) -> ("Array of clusters"=w1397:cluster{"Y data in":dbl[], "X data in":dbl[]}[], "error out"=w1339:errorcluster)  [unwired: 1 in]
            n420 = call "4155C Split array.vi"("Number of VAR2 steps"=w1354, "Y2 data in"=w1351, "X data in"=w1360, "Y1 data in"=w1353, "Y3 data in"=w1349, "error in (no error)"=w1339) -> ("Array of clusters"=w1396:cluster{"Y data in":dbl[], "X data in":dbl[]}[], "error out"=w1338:errorcluster)  [unwired: 1 in]
            n421 = call "4155C Config Chart Colours.vi"("Numeric"=w1354, "XY Graph 2"=w1389) -> ()  [unwired: 6 in]
            n422 = call "4155C Config Chart Colours.vi"("Numeric"=w1354, "XY Graph 2"=w1388) -> ()  [unwired: 6 in]
            n423 = call "4155C Config Chart Colours.vi"("Numeric"=w1354, "XY Graph 2"=w1357) -> ()  [unwired: 6 in]
            n424 = call "4155C Config Chart Colours.vi"("Numeric"=w1354, "XY Graph 2"=w1356) -> ()  [unwired: 6 in]
            n425 = call "4155C Config Chart Colours.vi"("Numeric"=w1354, "XY Graph 2"=w1398) -> ()  [unwired: 6 in]
            n426 = local write "Imax vs time"(w1397) -> ()
            n427 = local write "Imin vs time"(w1396) -> ()
            n428 = local write "Ion vs time"(w1358) -> ()
            n429 = local write "Ioff vs time"(w1359) -> ()
          }
        }
        n430 = call "4155C Split array.vi"("Number of VAR2 steps"=w1201, "Y2 data in"=w1243, "X data in"=w1245, "Y1 data in"=w1244, "Y3 data in"=w1243, "error in (no error)"=w1211) -> ("Array of clusters"=w1246:cluster{"Y data in":dbl[], "X data in":dbl[]}[], "error out"=w1210:errorcluster)  [unwired: 1 in]
        n431 = call "4155C Split array.vi"("Number of VAR2 steps"=w1201, "Y2 data in"=w1199, "X data in"=w1245, "Y1 data in"=w1199, "Y3 data in"=w1198, "error in (no error)"=w1210) -> ("Array of clusters"=w1248:cluster{"Y data in":dbl[], "X data in":dbl[]}[], "error out"=w1247:errorcluster)  [unwired: 1 in]
        n432 = local write "I vs Vd"(w1248) -> ()
        n433 = local write "Vp vs Vg (FPP)"(w1246) -> ()
        n434 = Open/Create/Replace File(file path (use dialog)=w1306, error in=w1247, operation (0:open)=w1266) -> (refnum out=w1316:refnum<file>, error out=w1317:errorcluster)  [unwired: 3 in, 1 out]
        n435 = call "4155C Make Big 2d array FPP.vi"("1D Var1"=w1245, "1d ID"=w1199, "1d Vp2"=w1244, "1d IG"=w1198, "1d Vp1"=w1243, "VAR2 START"=w1267, "Number of VAR2 steps"=w1201, "VAR2 STEP"=w1269, "VAR1 Name"="Vd", "Decimal places in header"=i8 1, "VAR2 Name"="Vg") -> ("Header array"=w1312:string[], "Data array"=w1313:dbl[][])  [unwired: 15 in]
        n436 = call "4155C Write array to file.vi"("Byte Stream File Refnum"=w1316, "Header"=w1312, "Data Array"=w1313, "error in (no error)"=w1317) -> ("dup refnum"=w1314:refnum<file>, "error out"=w1315:errorcluster)  [unwired: 1 in]
        n437 = call "4155C Config Chart Colours.vi"("Numeric"=w1201, "XY Graph 2"=w1242) -> ()  [unwired: 6 in]
        n438 = call "4155C Config Chart Colours.vi"("Numeric"=w1201, "XY Graph 2"=w1241) -> ()  [unwired: 6 in]
        n439 = Close File(refnum=w1314, error in=w1315) -> (error out=w1301:errorcluster)  [unwired: 1 out]
      }
      frame "itime" {
        n440 = Delete From Array(array=w1418, index=1) -> (deleted portion=w1417:string)  [unwired: 1 in, 1 out]
        n441 = Delete From Array(array=w1418, index=0 ("Index")) -> (deleted portion=w1452:string)  [unwired: 1 in, 1 out]
        n442 = Fract/Exp String To Number(string=w1417) -> (number=w1416:dbl)  [unwired: 3 in, 1 out]
        n443 = case shown="\"l\"" w1452 {
          tunnel: w1451 -> [w1457 w1459 w1463]
          tunnel: [w1456 w1458 w1462] -> w1444
          tunnel: w1416 -> [w1454 _ w1461]
          frame "s" {
            w1455 = u32 0 items=["short  ", "medium  ", "long  "] ("integration time 2")
            n444 = Bundle By Name(cluster=w1457, "integration time"=w1455, "Short/Long integration time"=w1454) -> (w1456:T5)
          }
          frame "m", Default {
            w1460 = u32 1 items=["short  ", "medium  ", "long  "] ("integration time 2")
            n445 = Bundle By Name(cluster=w1459, "integration time"=w1460) -> (w1458:T5)
          }
          frame "l" {
            w1464 = u32 2 items=["short  ", "medium  ", "long  "] ("integration time 2")
            n446 = Bundle By Name(cluster=w1463, "integration time"=w1464, "Short/Long integration time"=w1461) -> (w1462:T5)
          }
        }
      }
      frame "pulsed" {
        n447 = Delete From Array(array=w1507, index=0 ("Index")) -> (deleted portion=w1508:string, array with subset deleted=w1495:string[])  [unwired: 1 in]
        n448 = case shown="\"on\", Default" w1508 {
          tunnel: w1506 -> [w1518 w1521]
          tunnel: [w1517 w1520] -> w1499
          tunnel: w1495 -> [w1515 _]
          frame "on", Default {
            w1516 = u16 1 items=["Continuous", "Pulsed"] ("sweep method")
            n449 = Fract/Exp String To Number(string=w1515) -> (number=w1513:dbl[])  [unwired: 3 in, 1 out]
            n450 = Index Array(array=w1513, index #1=0 ("Index")) -> (element #1=w1512:dbl, element #2=w1511:dbl, element #3=w1510:dbl)  [unwired: 2 in]
            n451 = Bundle By Name(cluster=w1518, "sweep method"=w1516, "Pulse period"=w1512, "Base voltage"=w1511, "Pulse width"=w1510) -> (w1517:T5)
          }
          frame "off" {
            w1519 = u16 0 items=["Continuous", "Pulsed"] ("sweep method")
            n452 = Bundle By Name(cluster=w1521, "sweep method"=w1519) -> (w1520:T5)
          }
        }
      }
      frame "gaterangemode" {
        n453 = Delete From Array(array=w1562, index=0 ("Index")) -> (deleted portion=w1563:string)  [unwired: 1 in, 1 out]
        n454 = case shown="\"f\"" w1563 {
          tunnel: [w1565 w1566 w1567] -> w1552
          frame "a", Default {
            w1565 = u16 0 items=["Auto", "Limited", "Fixed"] ("Gate Range\nmode 2")
          }
          frame "f" {
            w1566 = u16 2 items=["Auto", "Limited", "Fixed"] ("Gate Range\nmode 2")
          }
          frame "l" {
            w1567 = u16 1 items=["Auto", "Limited", "Fixed"] ("Gate Range\nmode 2")
          }
        }
      }
      frame "gaterange" {
        (unwired) u8 11 items=["10fA  ", "100fA  ", "1nA  ", "10nA", "100nA", "1uA", "10uA", "100uA", "1mA", "10mA", "100mA", "1A"] ("Gate Range 2")
        n455 = Delete From Array(array=w1615, index=0 ("Index")) -> (deleted portion=w1605:string)  [unwired: 1 in, 1 out]
        n456 = Scan Value(string=w1605, format string="") -> (value=w1603:dbl)  [unwired: 1 in, 1 out]
        n457 = Logarithm Base 10(1:w1603) -> (0:w1602:dbl)
        n458 = Round To Nearest(number=w1602) -> (nearest integer value=w1601:dbl)
        n459 = Add(x=w1601, y=11.0) -> (x+y=w1599:dbl)
        n460 = To Unsigned Byte Integer(number=w1599) -> (unsigned 8bit integer=w1598:u8)
      }
      frame "drainrange" {
        (unwired) u8 11 items=["10fA  ", "100fA  ", "1nA  ", "10nA", "100nA", "1uA", "10uA", "100uA", "1mA", "10mA", "100mA", "1A"] ("Gate Range 2")
        n461 = Delete From Array(array=w1664, index=0 ("Index")) -> (deleted portion=w1655:string)  [unwired: 1 in, 1 out]
        n462 = Scan Value(string=w1655, format string="") -> (value=w1653:dbl)  [unwired: 1 in, 1 out]
        n463 = Logarithm Base 10(1:w1653) -> (0:w1652:dbl)
        n464 = Round To Nearest(number=w1652) -> (nearest integer value=w1651:dbl)
        n465 = Add(x=w1651, y=11.0) -> (x+y=w1649:dbl)
        n466 = To Unsigned Byte Integer(number=w1649) -> (unsigned 8bit integer=w1648:u8)
      }
      frame "drainrangemode" {
        n467 = Delete From Array(array=w1706, index=0 ("Index")) -> (deleted portion=w1707:string)  [unwired: 1 in, 1 out]
        n468 = case shown="\"f\"" w1707 {
          tunnel: [w1709 w1710 w1711] -> w1696
          frame "a", Default {
            w1709 = u16 0 items=["Auto", "Limited", "Fixed"] ("Gate Range\nmode 2")
          }
          frame "f" {
            w1710 = u16 2 items=["Auto", "Limited", "Fixed"] ("Gate Range\nmode 2")
          }
          frame "l" {
            w1711 = u16 1 items=["Auto", "Limited", "Fixed"] ("Gate Range\nmode 2")
          }
        }
      }
      frame "Error", Default {
      }
      frame "logfile" {
        n469 = Number To Decimal String(number=w1782) -> (decimal integer string=w1817:string)  [unwired: 1 in]
        n470 = Concatenate Strings(w1816, "logfile" ("Substring"), w1817, w1780, ".txt" ("Substring")) -> (w1814:string)
        n471 = String To Path(string=w1814) -> (path=w1787:path)
        n472 = Unbundle(w1813) -> ("integration time"=w1812:u32, "Short/Long integration time"=w1811:dbl, "hold time (sec)"=w1810:dbl, "delay time (sec)"=w1809:dbl, "Step Time (0 disables)"=w1808:dbl, "sweep method"=w1807:u16, "Pulse period"=w1806:dbl, "Base voltage"=w1805:dbl, "Pulse width"=w1804:dbl)
        n473 = Build Array(w1812, w1811, w1810, w1809, w1808, w1807, w1806, w1805, w1804, w1798, w1799, w1800, w1801, w1802, w1803) -> (w1791:dbl[])
        n474 = Insert Into Array(array=dbl[][] [] ("Input Array"), new element=w1791) -> (w1790:dbl[][])  [unwired: 2 in]
        n475 = call <vilib>:"compatOverwrite.vi"("overwrite (F)"=TRUE) -> ("overwrite?"=w1785:T8)
        n476 = Open/Create/Replace File(file path (use dialog)=w1787, error in=w1789, operation (0:open)=w1785) -> (refnum out=w1795:refnum<file>, error out=w1794:errorcluster)  [unwired: 3 in, 1 out]
        n477 = call "4155C Write array to file.vi"("Byte Stream File Refnum"=w1795, "Header"=string[] ["Int Time", "Short/Long Itime", "Hold time", "Delay time", "Step time", "Sweep method", "Pulse period", "Base Voltage", "Pulse width", "Drain compliance", "Gate compliance", "Gate range mode", "Gate range", "S/D range mode", "S/D range"], "Data Array"=w1790, "error in (no error)"=w1794) -> ("dup refnum"=w1797:refnum<file>, "error out"=w1796:errorcluster)  [unwired: 1 in]
        n478 = Close File(refnum=w1797, error in=w1796) -> (error out=w1788:errorcluster)  [unwired: 1 out]
      }
      frame "sample" {
        w1859 = 1
        # "The suffix is Vg_Vd_Time."
        # "Add a time offset (elapsed time) to the time axis."
        # "Adjusts graph colors."
        n479 = Number To Decimal String(number=w1893) -> (decimal integer string=w1931:string)  [unwired: 1 in]
        n480 = local read "Sample - Drain"() -> (w1827:u32)
        n481 = Fract/Exp String To Number(string=w1929) -> (number=w1897:dbl[])  [unwired: 3 in, 1 out]
        n482 = Index Array(array=w1897, index=0 ("Index")) -> (element=w1851:dbl)
        n483 = Index Array(array=w1897, index=2 ("Index")) -> (element=w1925:dbl)
        n484 = Index Array(array=w1897, index=3 ("Index")) -> (element=w1848:dbl)
        n485 = Index Array(array=w1897, index=4 ("Index")) -> (element=w1896:dbl)
        n486 = Index Array(array=w1897, index=1 ("Index")) -> (element=w1853:dbl)
        n487 = local read "Sample - Probe 4"() -> (w1830:u32)
        n488 = local read "Sample - Source/Common"() -> (w1828:u32)
        n489 = local read "Time Units"() -> (w1823:u16)
        n490 = local read "Sample - Gate"() -> (w1829:u32)
        n491 = call "4155C Config Sampling Measurements v3.0.vi"("VISA session"=w1934, "Num Points"=w1925, "Sample - Drain"=w1827, "Display on/off"=TRUE, "Gate Compliance"=w1912, "Sampling interval"=w1896, "Sample - Source/Common"=w1828, "Sample - Probe 4"=w1830, "Drain Compliance"=w1932, "Standby"=w1831, "error in (no error)"=w1933, "Timings"=w1904, "Sample - Gate"=w1829, "Sample time"=w1848) -> ("dup VISA resource name"=w1936:refnum<visa-resource-name>, "error out"=w1935:errorcluster)
        n492 = local read "Plot sample extrema vs time"() -> (w1861:bool)
        n493 = Number To Decimal String(number=w1853) -> (decimal integer string=w1854:string)  [unwired: 1 in]
        n494 = Number To Decimal String(number=w1851) -> (decimal integer string=w1850:string)  [unwired: 1 in]
        n495 = Number To Decimal String(number=w1848) -> (decimal integer string=w1847:string)  [unwired: 1 in]
        n496 = call "4155C Take Sample v3.0.vi"("VISA resource name in"=w1936, "Emergency Stop"=w1909, "Sample - Gate"=w1829, "Vg"=w1851, "Sample - Drain"=w1827, "Vd"=w1853, "error in (no error)"=w1935) -> ("Time"=w1824:dbl[], "VISA Resource Name out"=w1906:refnum<visa-resource-name>, "Ig"=w1841:dbl[], "Id"=w1842:dbl[], "Is"=w1843:dbl[], "error out"=w1869:errorcluster)  [unwired: 3 in]
        n497 = Insert Into Array(array=w1835, new element=w1842) -> (w1838:dbl[])  [unwired: 1 in]
        n498 = case shown="2" w1823 {
          tunnel: [w1939 w1940 w1943] -> w1826
          tunnel: w1824 -> [w1938 w1940 w1942]
          frame 2 {
            n499 = Divide(x=w1938, y=3600.0) -> (x/y=w1939:dbl[])
          }
          frame 0, Default {
          }
          frame 1 {
            n500 = Divide(x=w1942, y=60.0) -> (x/y=w1943:dbl[])
          }
        }
        n501 = Insert Into Array(array=w1834, new element=w1843) -> (w1840:dbl[])  [unwired: 1 in]
        n502 = Insert Into Array(array=w1836, new element=w1841) -> (w1839:dbl[])  [unwired: 1 in]
        n503 = Concatenate Strings(w1854, "_" ("Substring"), w1850, "_" ("Substring"), w1847, ".txt" ("Substring")) -> (w1845:string)
        n504 = Concatenate Strings(w1856, w1855, w1931, w1891, "_S_" ("Substring"), w1845) -> (w1930:string)
        n505 = String To Path(string=w1930) -> (path=w1915:path)
        n506 = Add(x=w1826, y=w1825) -> (x+y=w1844:dbl[])
        n507 = Insert Into Array(array=w1833, new element=w1844) -> (w1837:dbl[])  [unwired: 1 in]
        n508 = case shown="True" w1861 {
          tunnel: w1844 -> [_ w1946]
          tunnel: [w1944 w1947] -> w1858
          tunnel: w1862 -> [w1944 w1945]
          frame False {
          }
          frame True {
            n509 = Insert Into Array(array=w1945, new element=w1946) -> (w1947:i32[])  [unwired: 1 in]
          }
        }
        n510 = case shown="True" "Plot sample extrema vs time" {
          tunnel: w1843 -> [_ w1976]
          tunnel: w1842 -> [_ w1977]
          tunnel: w1841 -> [_ w1978]
          tunnel: [w1954 w1964] -> w1832
          tunnel: w1869 -> [w1954 w1969]
          tunnel: w1875 -> [w1953 w1981]
          tunnel: w1874 -> [w1952 w1980]
          tunnel: w1873 -> [w1951 w1982]
          tunnel: w1872 -> [w1950 w1979]
          tunnel: w1871 -> [w1949 w1984]
          tunnel: w1870 -> [w1948 w1983]
          tunnel: [w1953 w1968] -> w1868
          tunnel: [w1952 w1962] -> w1867
          tunnel: [w1951 w1966] -> w1866
          tunnel: [w1950 w1961] -> w1865
          tunnel: [w1949 w1967] -> w1864
          tunnel: [w1948 w1960] -> w1863
          tunnel: w1858 -> [_ w1958]
          frame False {
          }
          frame True {
            w1963 = 1
            # "Number of VAR2 steps is 1."
            # "abs(Ig)"
            # "abs(Is)"
            # "abs(Id)"
            # "Adjusts graph colors."
            n511 = Absolute Value(x=w1978) -> (abs(x)=w1955:dbl[])
            n512 = Absolute Value(x=w1977) -> (abs(x)=w1956:dbl[])
            n513 = Absolute Value(x=w1976) -> (abs(x)=w1957:dbl[])
            n514 = Array Max & Min(array=w1957) -> (max value=w1975:dbl, min value=w1972:dbl)  [unwired: 2 out]
            n515 = Array Max & Min(array=w1956) -> (max value=w1974:dbl, min value=w1971:dbl)  [unwired: 2 out]
            n516 = Array Max & Min(array=w1955) -> (max value=w1973:dbl, min value=w1970:dbl)  [unwired: 2 out]
            n517 = local write "Id max"(w1974) -> ()
            n518 = local write "Id min"(w1971) -> ()
            n519 = local write "Ig max"(w1973) -> ()
            n520 = local write "Ig min"(w1970) -> ()
            n521 = Insert Into Array(array=w1984, new element=w1955) -> (w1967:dbl[])  [unwired: 1 in]
            n522 = Insert Into Array(array=w1983, new element=w1955) -> (w1960:dbl[])  [unwired: 1 in]
            n523 = local write "Is max"(w1975) -> ()
            n524 = local write "Is min"(w1972) -> ()
            n525 = Insert Into Array(array=w1982, new element=w1956) -> (w1966:dbl[])  [unwired: 1 in]
            n526 = Insert Into Array(array=w1979, new element=w1956) -> (w1961:dbl[])  [unwired: 1 in]
            n527 = Insert Into Array(array=w1981, new element=w1957) -> (w1968:dbl[])  [unwired: 1 in]
            n528 = Insert Into Array(array=w1980, new element=w1957) -> (w1962:dbl[])  [unwired: 1 in]
            n529 = control-ref of="Imax vs time"() -> (w1985:refnum<vi>)
            n530 = call "4155C Config Chart Colours.vi"("Numeric"=w1963, "XY Graph 2"=w1985) -> ()  [unwired: 6 in]
            n531 = call "4155C Split array.vi"("Number of VAR2 steps"=w1963, "Y2 data in"=w1966, "X data in"=w1958, "Y1 data in"=w1968, "Y3 data in"=w1967, "error in (no error)"=w1969) -> ("Array of clusters"=w1986:cluster{"Y data in":dbl[], "X data in":dbl[]}[], "error out"=w1965:errorcluster)  [unwired: 1 in]
            n532 = call "4155C Split array.vi"("Number of VAR2 steps"=w1963, "Y2 data in"=w1961, "X data in"=w1958, "Y1 data in"=w1962, "Y3 data in"=w1960, "error in (no error)"=w1965) -> ("Array of clusters"=w1959:cluster{"Y data in":dbl[], "X data in":dbl[]}[], "error out"=w1964:errorcluster)  [unwired: 1 in]
            n533 = local write "Imax vs time"(w1986) -> ()
            n534 = local write "Imin vs time"(w1959) -> ()
          }
        }
        n535 = control-ref of="I vs time (Bias Stress)"() -> (w1857:refnum<vi>)
        n536 = call "4155C Split array.vi"("Number of VAR2 steps"=w1859, "Y2 data in"=w1838, "X data in"=w1837, "Y1 data in"=w1840, "Y3 data in"=w1839) -> ("Array of clusters"=w1860:cluster{"Y data in":dbl[], "X data in":dbl[]}[])  [unwired: 2 in, 1 out]
        n537 = local write "I vs time (Bias Stress)"(w1860) -> ()
        n538 = call "4155C Config Chart Colours.vi"("Numeric"=w1859, "XY Graph 2"=w1857) -> ()  [unwired: 6 in]
        n539 = Insert Into Array(array=dbl[][] [] ("Input Array"), new element=w1844) -> (w1919:dbl[][])  [unwired: 2 in]
        n540 = Insert Into Array(array=w1919, new element=w1841) -> (w1918:dbl[][])  [unwired: 2 in]
        n541 = VISA Write(VISA resource name=w1906, write buffer=":DISP ON" ("write buffer (\"\")"), error in (no error)=w1832) -> (VISA resource name out=w1905:refnum<visa-resource-name>, error out=w1907:errorcluster)  [unwired: 1 out]
        n542 = Insert Into Array(array=w1918, new element=w1842) -> (w1917:dbl[][])  [unwired: 2 in]
        n543 = Insert Into Array(array=w1917, new element=w1843) -> (w1911:dbl[][])  [unwired: 2 in]
        n544 = call <vilib>:"compatOverwrite.vi"("overwrite (F)"=TRUE) -> ("overwrite?"=w1894:T8)
        n545 = Open/Create/Replace File(file path (use dialog)=w1915, error in=w1907, operation (0:open)=w1894) -> (refnum out=w1922:refnum<file>, error out=w1921:errorcluster)  [unwired: 3 in, 1 out]
        n546 = Transpose 2D Array(2D array=w1911) -> (transposed array=w1910:dbl[][])
        n547 = call "4155C Write array to file.vi"("Byte Stream File Refnum"=w1922, "Header"=string[] ["Time /Units", "Ig /A", "Id /A", "Is /A"], "Data Array"=w1910, "error in (no error)"=w1921) -> ("dup refnum"=w1924:refnum<file>, "error out"=w1923:errorcluster)  [unwired: 1 in]
        n548 = Close File(refnum=w1924, error in=w1923) -> (error out=w1913:errorcluster)  [unwired: 1 out]
      }
      frame "samplei" {
        w1999 = 1
        # "Adjusts graph colors."
        # "Add a time offset (elapsed time) to the time axis."
        n549 = Number To Decimal String(number=w2040) -> (decimal integer string=w2088:string)  [unwired: 1 in]
        n550 = local read "Sample I - Probe 4 (Disabled)"() -> (w2014:u32)
        n551 = local read "Sample I - Source/Common"() -> (w2011:u32)
        n552 = Concatenate Strings(w2069, "-samplei-" ("Substring"), w2088, w2039, ".txt" ("Substring")) -> (w2086:string)
        n553 = Fract/Exp String To Number(string=w2085) -> (number=w2054:dbl[])  [unwired: 3 in, 1 out]
        n554 = String To Path(string=w2086) -> (path=w2072:path)
        n555 = Index Array(array=w2054, index=4 ("Index")) -> (element=w2048:dbl)
        n556 = Index Array(array=w2054, index=3 ("Index")) -> (element=w2049:dbl)
        n557 = Index Array(array=w2054, index=1 ("Index")) -> (element=w2051:dbl)
        n558 = Index Array(array=w2054, index=0 ("Index")) -> (element=w2052:dbl)
        n559 = local read "Sample I - Drain/Gate"() -> (w2013:u32)
        n560 = Index Array(array=w2054, index=2 ("Index")) -> (element=w2050:dbl)
        n561 = local read "Plot sample extrema vs time"() -> (w2008:bool)
        n562 = local read "Time Units"() -> (w2005:u16)
        n563 = local read "Sample I - Probe 3 (Disabled)"() -> (w2012:u32)
        n564 = call "4155C Config SamplingI Measurements v3.0.vi"("VISA session"=w2091, "Num Points"=w2051, "Sample I - Probe 3 (Disabled)"=w2012, "Display on/off"=TRUE, "Sample I - Source/Common"=w2011, "Sample I - Drain/Gate"=w2013, "Sampling interval"=w2049, "Standby"=w2015, "error in (no error)"=w2090, "Timings"=w2061, "Sample I - Probe 4 (Disabled)"=w2014, "Sample time"=w2050) -> ("dup VISA resource name"=w2093:refnum<visa-resource-name>, "error out"=w2092:errorcluster)  [unwired: 2 in]
        n565 = call "4155C Take SampleI v3.0.vi"("Sample I - Drain/Gate"=w2013, "Emergency Stop"=w2066, "error in (no error)"=w2092, "Idg 2"=w2052, "Vdg compliance 2"=w2048, "VISA resource name in"=w2093) -> ("error out"=w2064:errorcluster, "Idg"=w1991:dbl[], "Vdg"=w1992:dbl[], "VISA Resource Name out"=w2062:refnum<visa-resource-name>, "Is"=w1988:dbl[], "Time"=w2003:dbl[])
        n566 = case shown="2" w2005 {
          tunnel: [w2096 w2097 w2100] -> w2004
          tunnel: w2003 -> [w2095 w2097 w2099]
          frame 2 {
            n567 = Divide(x=w2095, y=3600.0) -> (x/y=w2096:dbl[])
          }
          frame 0, Default {
          }
          frame 1 {
            n568 = Divide(x=w2099, y=60.0) -> (x/y=w2100:dbl[])
          }
        }
        n569 = control-ref of="Vdg vs time (Bias Stress)"() -> (w2000:refnum<vi>)
        n570 = Add(x=w2004, y=w2002) -> (x+y=w1997:dbl[])
        n571 = Insert Into Array(array=w1998, new element=w1997) -> (w1996:dbl[])  [unwired: 1 in]
        n572 = case shown="True" w2008 {
          tunnel: w1997 -> [_ w2103]
          tunnel: [w2101 w2104] -> w2006
          tunnel: w2007 -> [w2101 w2102]
          frame False {
          }
          frame True {
            n573 = Insert Into Array(array=w2102, new element=w2103) -> (w2104:i32[])  [unwired: 1 in]
          }
        }
        n574 = Insert Into Array(array=w1993, new element=w1992) -> (w1987:dbl[])  [unwired: 1 in]
        n575 = call "4155C Split array.vi"("Number of VAR2 steps"=w1999, "X data in"=w1996, "Y1 data in"=w1987) -> ("Array of clusters"=w2001:cluster{"Y data in":dbl[], "X data in":dbl[]}[])  [unwired: 4 in, 1 out]
        n576 = local write "Vdg vs time (Bias Stress)"(w2001) -> ()
        n577 = Insert Into Array(array=dbl[][] [] ("Input Array"), new element=w1997) -> (w2076:dbl[][])  [unwired: 2 in]
        n578 = call "4155C Config Chart Colours.vi"("Numeric"=w1999, "XY Graph 2"=w2000) -> ()  [unwired: 6 in]
        n579 = Insert Into Array(array=w1995, new element=w1991) -> (w1994:dbl[])  [unwired: 1 in]
        n580 = Insert Into Array(array=w2076, new element=w1992) -> (w2075:dbl[][])  [unwired: 2 in]
        n581 = Insert Into Array(array=w1990, new element=w1988) -> (w1989:dbl[])  [unwired: 1 in]
        n582 = Insert Into Array(array=w2075, new element=w1991) -> (w2074:dbl[][])  [unwired: 2 in]
        n583 = VISA Write(VISA resource name=w2062, write buffer=":DISP ON" ("write buffer (\"\")"), error in (no error)=w2064) -> (VISA resource name out=w2047:refnum<visa-resource-name>, error out=w2063:errorcluster)  [unwired: 1 out]
        n584 = Insert Into Array(array=w2074, new element=w1988) -> (w2068:dbl[][])  [unwired: 2 in]
        n585 = call <vilib>:"compatOverwrite.vi"("overwrite (F)"=TRUE) -> ("overwrite?"=w2042:T8)
        n586 = Open/Create/Replace File(file path (use dialog)=w2072, error in=w2063, operation (0:open)=w2042) -> (refnum out=w2079:refnum<file>, error out=w2078:errorcluster)  [unwired: 3 in, 1 out]
        n587 = Transpose 2D Array(2D array=w2068) -> (transposed array=w2067:dbl[][])
        n588 = call "4155C Write array to file.vi"("Byte Stream File Refnum"=w2079, "Header"=string[] ["Time /s", "Vdg /V", "Idg /A", "Is /A"], "Data Array"=w2067, "error in (no error)"=w2078) -> ("dup refnum"=w2081:refnum<file>, "error out"=w2080:errorcluster)  [unwired: 1 in]
        n589 = Close File(refnum=w2081, error in=w2080) -> (error out=w2045:errorcluster)  [unwired: 1 out]
        n590 = VISA Write(VISA resource name=w2047, write buffer=";:PAGE:SCON:STAN OFF;:PAGE:CHAN:VSU2:DIS;" ("write buffer (\"\")"), error in (no error)=w2045) -> (VISA resource name out=w2043:refnum<visa-resource-name>, error out=w2044:errorcluster)  [unwired: 1 out]
      }
      frame "#" {
        n591 = VISA Write(VISA resource name=w2139, write buffer=":DISP ON" ("write buffer (\"\")"), error in (no error)=w2138) -> (VISA resource name out=w2137:refnum<visa-resource-name>, error out=w2136:errorcluster)  [unwired: 1 out]
      }
      frame "stressV" {
        n592 = Number To Decimal String(number=w2180) -> (decimal integer string=w2221:string)  [unwired: 1 in]
        n593 = Concatenate Strings(w2205, "-stressV-" ("Substring"), w2221, w2179, ".txt" ("Substring")) -> (w2219:string)
        n594 = Fract/Exp String To Number(string=w2218) -> (number=w2191:dbl[])  [unwired: 3 in, 1 out]
        n595 = local read "Stress V - Source/Common"() -> (w2154:u32)
        n596 = String To Path(string=w2219) -> (path=w2209:path)
        n597 = Index Array(array=w2191, index=3 ("Index")) -> (element=w2188:dbl)
        n598 = Index Array(array=w2191, index=1 ("Index")) -> (element=w2186:dbl)
        n599 = Index Array(array=w2191, index=0 ("Index")) -> (element=w2185:dbl)
        n600 = Index Array(array=w2191, index=4 ("Index")) -> (element=w2190:dbl)
        n601 = Index Array(array=w2191, index=2 ("Index")) -> (element=w2187:dbl)
        n602 = local read "Stress V - Drain"() -> (w2153:u32)
        n603 = local read "Stress V - Gate"() -> (w2152:u32)
        n604 = call "4155C Config V Stress v3.0.vi"("Display on/off"=TRUE, "Stress V - Gate"=w2152, "Stress V - Drain"=w2153, "Stress V - Source/Common"=w2154, "IG compliance"=w2187, "ID compliance"=w2188, "error in (no error)"=w2223, "VG"=w2185, "VD"=w2186, "VISA session"=w2224) -> ("error out"=w2225:errorcluster, "dup VISA resource name"=w2226:refnum<visa-resource-name>)
        n605 = call "4155C Apply Stress.vi"("error in (no error)"=w2225, "Duration"=w2190, "Emergency Stop"=w2204, "VISA resource name in"=w2226) -> ("error out"=w2202:errorcluster, "VISA Resource Name out"=w2200:refnum<visa-resource-name>)
        n606 = VISA Write(VISA resource name=w2200, write buffer=":DISP ON" ("write buffer (\"\")"), error in (no error)=w2202) -> (VISA resource name out=w2199:refnum<visa-resource-name>, error out=w2201:errorcluster)  [unwired: 1 out]
        n607 = call <vilib>:"compatOverwrite.vi"("overwrite (F)"=TRUE) -> ("overwrite?"=w2184:T8)
        n608 = Open/Create/Replace File(file path (use dialog)=w2209, error in=w2201, operation (0:open)=w2184) -> (refnum out=w2212:refnum<file>, error out=w2211:errorcluster)  [unwired: 3 in, 1 out]
        n609 = call "4155C Write array to file.vi"("Byte Stream File Refnum"=w2212, "Header"=string[] ["V stress completed successfully", ""], "error in (no error)"=w2211) -> ("dup refnum"=w2214:refnum<file>, "error out"=w2213:errorcluster)  [unwired: 2 in]
        n610 = Close File(refnum=w2214, error in=w2213) -> (error out=w2207:errorcluster)  [unwired: 1 out]
      }
      frame "stressI" {
        n611 = local read "Stress I - Source/Common"() -> (w2231:u32)
        n612 = Number To Decimal String(number=w2258) -> (decimal integer string=w2295:string)  [unwired: 1 in]
        n613 = Concatenate Strings(w2279, "-stressI-" ("Substring"), w2295, w2257, ".txt" ("Substring")) -> (w2293:string)
        n614 = Fract/Exp String To Number(string=w2292) -> (number=w2267:dbl[])  [unwired: 3 in, 1 out]
        n615 = Index Array(array=w2267, index=1 ("Index")) -> (element=w2263:dbl)
        n616 = Index Array(array=w2267, index=0 ("Index")) -> (element=w2264:dbl)
        n617 = Index Array(array=w2267, index=2 ("Index")) -> (element=w2265:dbl)
        n618 = String To Path(string=w2293) -> (path=w2283:path)
        n619 = local read "Stress I - Drain/Gate"() -> (w2232:u32)
        n620 = call "4155C Config I Stress v3.0.vi"("Stress I - Drain/Gate"=w2232, "Stress I - Source/Common"=w2231, "Display on/off"=TRUE, "error in (no error)"=w2297, "VDG compliance"=w2263, "IDG"=w2264, "VISA session"=w2298) -> ("error out"=w2299:errorcluster, "dup VISA resource name"=w2300:refnum<visa-resource-name>)  [unwired: 1 in]
        n621 = call "4155C Apply Stress.vi"("error in (no error)"=w2299, "Duration"=w2265, "Emergency Stop"=w2278, "VISA resource name in"=w2300) -> ("error out"=w2276:errorcluster, "VISA Resource Name out"=w2274:refnum<visa-resource-name>)
        n622 = VISA Write(VISA resource name=w2274, write buffer=":DISP ON" ("write buffer (\"\")"), error in (no error)=w2276) -> (VISA resource name out=w2273:refnum<visa-resource-name>, error out=w2275:errorcluster)  [unwired: 1 out]
        n623 = call <vilib>:"compatOverwrite.vi"("overwrite (F)"=TRUE) -> ("overwrite?"=w2262:T8)
        n624 = Open/Create/Replace File(file path (use dialog)=w2283, error in=w2275, operation (0:open)=w2262) -> (refnum out=w2286:refnum<file>, error out=w2285:errorcluster)  [unwired: 3 in, 1 out]
        n625 = call "4155C Write array to file.vi"("Byte Stream File Refnum"=w2286, "Header"=string[] ["I stress completed successfully", ""], "error in (no error)"=w2285) -> ("dup refnum"=w2288:refnum<file>, "error out"=w2287:errorcluster)  [unwired: 2 in]
        n626 = Close File(refnum=w2288, error in=w2287) -> (error out=w2281:errorcluster)  [unwired: 1 out]
      }
      frame "vsu2pulse" {
        n627 = Number To Decimal String(number=w2331) -> (decimal integer string=w2366:string)  [unwired: 1 in]
        n628 = Concatenate Strings(w2351, "-vsu2-" ("Substring"), w2366, w2330, ".txt" ("Substring")) -> (w2364:string)
        n629 = Fract/Exp String To Number(string=w2363) -> (number=w2339:dbl[])  [unwired: 3 in, 1 out]
        n630 = String To Path(string=w2364) -> (path=w2355:path)
        n631 = Index Array(array=w2339, index=1 ("Index")) -> (element=w2338:dbl)
        n632 = Index Array(array=w2339, index=0 ("Index")) -> (element=w2336:dbl)
        n633 = local read "VSU2 Stress - Source/Common"() -> (w2305:u32)
        n634 = call "4155C Config VSU2 Stress v3.0.vi"("VISA session"=w2369, "Display on/off"=TRUE, "VSU2"=w2336, "error in (no error)"=w2368, "VSU2 Stress - Source/Common"=w2305) -> ("dup VISA resource name"=w2371:refnum<visa-resource-name>, "error out"=w2370:errorcluster)
        n635 = call "4155C Apply Stress.vi"("error in (no error)"=w2370, "Duration"=w2338, "Emergency Stop"=w2350, "VISA resource name in"=w2371) -> ("error out"=w2348:errorcluster, "VISA Resource Name out"=w2346:refnum<visa-resource-name>)
        n636 = VISA Write(VISA resource name=w2346, write buffer=":DISP ON" ("write buffer (\"\")"), error in (no error)=w2348) -> (VISA resource name out=w2345:refnum<visa-resource-name>, error out=w2347:errorcluster)  [unwired: 1 out]
        n637 = call <vilib>:"compatOverwrite.vi"("overwrite (F)"=TRUE) -> ("overwrite?"=w2335:T8)
        n638 = Open/Create/Replace File(file path (use dialog)=w2355, error in=w2347, operation (0:open)=w2335) -> (refnum out=w2358:refnum<file>, error out=w2357:errorcluster)  [unwired: 3 in, 1 out]
        n639 = call "4155C Write array to file.vi"("Byte Stream File Refnum"=w2358, "Header"=string[] ["VSU2 pulse completed successfully", ""], "error in (no error)"=w2357) -> ("dup refnum"=w2360:refnum<file>, "error out"=w2359:errorcluster)  [unwired: 2 in]
        n640 = Close File(refnum=w2360, error in=w2359) -> (error out=w2353:errorcluster)  [unwired: 1 out]
      }
      frame "sample-fpp" {
        w2382 = 1
        w2447 = string[] ["Time /s", "Id VgVd /A", "Ig VgVd /A", "Vp1 VgVd /V", "Vp2 VgVd /V"] ("Header")
        w2451 = "%d" ("format string")
        # "Y1 = Y2 = ID\nY3 = IG"
        # "Y1 = Vp2\nY2 = Y3 = Vp1"
        # "Add a time offset (elapsed time) to the time axis."
        n641 = local read "Plot sample extrema vs time"() -> (w2391:bool)
        n642 = Number To Decimal String(number=w2439) -> (decimal integer string=w2493:string)  [unwired: 1 in]
        n643 = Fract/Exp String To Number(string=w2490) -> (number=w2478:dbl[])  [unwired: 3 in, 1 out]
        n644 = local read "Plot sample extrema vs time"() -> (w2394:bool)
        n645 = Concatenate Strings(w2484, "-samplefpp-" ("Substring"), w2493, w2438, ".txt" ("Substring")) -> (w2491:string)
        n646 = local read "FPP - Source"() -> (w2417:u32)
        n647 = local read "FPP - Drain"() -> (w2418:u32)
        n648 = local read "FPP - Gate"() -> (w2419:u32)
        n649 = local read "FPP - Probe 1"() -> (w2420:u32)
        n650 = control-ref of="I vs time (Bias Stress)"() -> (w2411:refnum<vi>)
        n651 = String To Path(string=w2491) -> (path=w2459:path)
        n652 = Index Array(array=w2478, index=0 ("Index")) -> (element=w2446:dbl)
        n653 = Index Array(array=w2478, index=1 ("Index")) -> (element=w2445:dbl)
        n654 = local read "Time Units"() -> (w2407:u16)
        n655 = Index Array(array=w2478, index=2 ("Index")) -> (element=w2486:dbl)
        n656 = Index Array(array=w2478, index=3 ("Index")) -> (element=w2476:dbl)
        n657 = Number To Decimal String(number=w2446) -> (decimal integer string=w2467:string)  [unwired: 1 in]
        n658 = local read "FPP - Probe 2"() -> (w2421:u32)
        n659 = call "4155C Config Sampling Measurements FPP v3.0.vi"("VISA session"=w2496, "Gate Compliance"=w2485, "FPP - Source"=w2417, "FPP - Drain"=w2418, "Drain Compliance"=w2494, "error in (no error)"=w2495, "Num Points"=w2486, "Timings"=w2483, "FPP - Gate"=w2419, "FPP - Probe 1"=w2420, "Vg"=w2446, "Vd"=w2445, "Display on/off"=TRUE, "Sample time"=w2476, "FPP - Probe 2"=w2421, "Standby"=w2422) -> ("dup VISA resource name"=w2461:refnum<visa-resource-name>, "error out"=w2460:errorcluster)  [unwired: 2 in]
        n660 = call "4155C Take Sample FPP.vi"("VISA resource name in"=w2461, "error in (no error)"=w2460, "Emergency Stop"=w2462) -> ("Time"=w2410:dbl[], "Vp1"=w2377:dbl[], "VISA Resource Name out"=w2443:refnum<visa-resource-name>, "Ig"=w2388:dbl[], "Id"=w2387:dbl[], "Vp2"=w2376:dbl[], "error out"=w2390:errorcluster)  [unwired: 10 in]
        n661 = Insert Into Array(array=w2415, new element=w2387) -> (w2374:dbl[])  [unwired: 1 in]
        n662 = Insert Into Array(array=w2416, new element=w2388) -> (w2413:dbl[])  [unwired: 1 in]
        n663 = Number To Decimal String(number=w2445) -> (decimal integer string=w2465:string)  [unwired: 1 in]
        n664 = call "4155C Config Chart Colours.vi"("Numeric"=w2382, "XY Graph 2"=w2411) -> ()  [unwired: 6 in]
        n665 = case shown="2" w2407 {
          tunnel: [w2536 w2537 w2540] -> w2409
          tunnel: w2410 -> [w2535 w2537 w2539]
          frame 2 {
            n666 = Divide(x=w2535, y=3600.0) -> (x/y=w2536:dbl[])
          }
          frame 0, Default {
          }
          frame 1 {
            n667 = Divide(x=w2539, y=60.0) -> (x/y=w2540:dbl[])
          }
        }
        n668 = Concatenate Strings("(Vg = " ("Substring"), w2467, "V, Vd = " ("Substring"), w2465, "V)" ("Substring")) -> (w2463:string)
        n669 = Add(x=w2409, y=w2408) -> (x+y=w2381:dbl[])
        n670 = case shown="True" w2391 {
          tunnel: w2381 -> [_ w2499]
          tunnel: [w2497 w2500] -> w2392
          tunnel: w2393 -> [w2497 w2498]
          frame False {
          }
          frame True {
            n671 = Insert Into Array(array=w2498, new element=w2499) -> (w2500:i32[])  [unwired: 1 in]
          }
        }
        n672 = case shown="True" w2394 {
          tunnel: w2387 -> [_ w2527]
          tunnel: w2388 -> [_ w2528]
          tunnel: [w2507 w2519] -> w2389
          tunnel: w2390 -> [w2507 w2522]
          tunnel: w2406 -> [w2506 w2512]
          tunnel: w2405 -> [w2505 w2511]
          tunnel: w2404 -> [w2504 w2530]
          tunnel: w2403 -> [w2503 w2529]
          tunnel: w2402 -> [w2502 w2531]
          tunnel: [w2506 w2512] -> w2400
          tunnel: [w2505 w2511] -> w2399
          tunnel: [w2504 w2508] -> w2398
          tunnel: [w2503 w2509] -> w2397
          tunnel: [w2502 w2521] -> w2396
          tunnel: [w2501 w2517] -> w2395
          tunnel: w2392 -> [_ w2515]
          tunnel: w2401 -> [w2501 w2510]
          frame False {
          }
          frame True {
            w2518 = 1
            # "Y1 = Y2 = ID\nY3 = IG"
            # "Number of VAR2 steps is 1."
            # "abs(Ig)"
            # "abs(Id)"
            # "Adjusts graph colors."
            n673 = Absolute Value(x=w2528) -> (abs(x)=w2513:dbl[])
            n674 = Absolute Value(x=w2527) -> (abs(x)=w2514:dbl[])
            n675 = Array Max & Min(array=w2514) -> (max value=w2526:dbl, min value=w2524:dbl)  [unwired: 2 out]
            n676 = Array Max & Min(array=w2513) -> (max value=w2525:dbl, min value=w2523:dbl)  [unwired: 2 out]
            n677 = Insert Into Array(array=w2531, new element=w2513) -> (w2521:dbl[])  [unwired: 1 in]
            n678 = local write "Id max"(w2526) -> ()
            n679 = local write "Id min"(w2524) -> ()
            n680 = local write "Ig max"(w2525) -> ()
            n681 = local write "Ig min"(w2523) -> ()
            n682 = Insert Into Array(array=w2510, new element=w2513) -> (w2517:dbl[])  [unwired: 1 in]
            n683 = Insert Into Array(array=w2530, new element=w2514) -> (w2508:dbl[])  [unwired: 1 in]
            n684 = Insert Into Array(array=w2529, new element=w2514) -> (w2509:dbl[])  [unwired: 1 in]
            n685 = control-ref of="Imax vs time"() -> (w2532:refnum<vi>)
            n686 = call "4155C Config Chart Colours.vi"("Numeric"=w2518, "XY Graph 2"=w2532) -> ()  [unwired: 6 in]
            n687 = call "4155C Split array.vi"("Number of VAR2 steps"=w2518, "Y2 data in"=w2508, "X data in"=w2515, "Y1 data in"=w2508, "Y3 data in"=w2521, "error in (no error)"=w2522) -> ("Array of clusters"=w2533:cluster{"Y data in":dbl[], "X data in":dbl[]}[], "error out"=w2520:errorcluster)  [unwired: 1 in]
            n688 = call "4155C Split array.vi"("Number of VAR2 steps"=w2518, "Y2 data in"=w2509, "X data in"=w2515, "Y1 data in"=w2509, "Y3 data in"=w2517, "error in (no error)"=w2520) -> ("Array of clusters"=w2516:cluster{"Y data in":dbl[], "X data in":dbl[]}[], "error out"=w2519:errorcluster)  [unwired: 1 in]
            n689 = local write "Imax vs time"(w2533) -> ()
            n690 = local write "Imin vs time"(w2516) -> ()
          }
        }
        n691 = Insert Into Array(array=w2414, new element=w2381) -> (w2383:dbl[])  [unwired: 1 in]
        n692 = call "4155C Split array.vi"("Number of VAR2 steps"=w2382, "Y2 data in"=w2374, "X data in"=w2383, "Y1 data in"=w2374, "Y3 data in"=w2413) -> ("Array of clusters"=w2412:cluster{"Y data in":dbl[], "X data in":dbl[]}[])  [unwired: 2 in, 1 out]
        n693 = local write "I vs time (Bias Stress)"(w2412) -> ()
        n694 = Insert Into Array(array=w2380, new element=w2377) -> (w2375:dbl[])  [unwired: 1 in]
        n695 = Insert Into Array(array=w2379, new element=w2376) -> (w2378:dbl[])  [unwired: 1 in]
        n696 = Insert Into Array(array=dbl[][] [] ("Input Array"), new element=w2381) -> (w2474:dbl[][])  [unwired: 2 in]
        n697 = control-ref of="Vp vs time (FPP Bias Stress)"() -> (w2384:refnum<vi>)
        n698 = Insert Into Array(array=w2474, new element=w2387) -> (w2473:dbl[][])  [unwired: 2 in]
        n699 = call <vilib>:"compatOverwrite.vi"("overwrite (F)"=TRUE) -> ("overwrite?"=w2441:T8)
        n700 = Open/Create/Replace File(file path (use dialog)=w2459, error in=w2389, operation (0:open)=w2441) -> (refnum out=w2456:refnum<file>, error out=w2457:errorcluster)  [unwired: 3 in, 1 out]
        n701 = Array To Spreadsheet String(array=w2447, 3:w2451) -> (spreadsheet string=w2453:string)  [unwired: 1 in]
        n702 = call "4155C Split array.vi"("Number of VAR2 steps"=w2382, "Y2 data in"=w2375, "X data in"=w2383, "Y1 data in"=w2378, "Y3 data in"=w2375) -> ("Array of clusters"=w2385:cluster{"Y data in":dbl[], "X data in":dbl[]}[])  [unwired: 2 in, 1 out]
        n703 = Insert Into Array(array=w2473, new element=w2388) -> (w2472:dbl[][])  [unwired: 2 in]
        n704 = Search and Replace String(replace all?=TRUE ("replace all? (F)"), input string=w2453, search string="VgVd", replace string=w2463) -> (result string=w2449:string)  [unwired: 4 in, 3 out]
        n705 = local write "Vp vs time (FPP Bias Stress)"(w2385) -> ()
        n706 = Insert Into Array(array=w2472, new element=w2377) -> (w2470:dbl[][])  [unwired: 2 in]
        n707 = call "4155C Config Chart Colours.vi"("Numeric"=w2382, "XY Graph 2"=w2384) -> ()  [unwired: 6 in]
        n708 = Spreadsheet String To Array(format string=w2451, spreadsheet string=w2449, array type (2D Dbl)=w2447) -> (array=w2448:string[])  [unwired: 1 in]
        n709 = Insert Into Array(array=w2470, new element=w2376) -> (w2444:dbl[][])  [unwired: 2 in]
        n710 = Transpose 2D Array(2D array=w2444) -> (transposed array=w2469:dbl[][])
        n711 = call "4155C Write array to file.vi"("Byte Stream File Refnum"=w2456, "Header"=w2448, "Data Array"=w2469, "error in (no error)"=w2457) -> ("dup refnum"=w2454:refnum<file>, "error out"=w2455:errorcluster)  [unwired: 1 in]
        n712 = Close File(refnum=w2454, error in=w2455) -> (error out=w2442:errorcluster)  [unwired: 1 out]
      }
      frame "resample-fpp" {
        w2551 = 1
        w2613 = string[] ["Time /s", "Id VgVd /A", "Ig VgVd /A", "Vp1 VgVd /V", "Vp2 VgVd /V"] ("Header")
        w2617 = "%d" ("format string")
        # "Y1 = Y2 = ID\nY3 = IG"
        # "Y1 = Vp2\nY2 = Y3 = Vp1"
        # "Add a time offset (elapsed time) to the time axis."
        n713 = Number To Decimal String(number=w2601) -> (decimal integer string=w2651:string)  [unwired: 1 in]
        n714 = local read "Plot sample extrema vs time"() -> (w2560:bool)
        n715 = Fract/Exp String To Number(string=w2648) -> (number=w2606:dbl[])  [unwired: 3 in, 1 out]
        n716 = Concatenate Strings(w2644, "-resamplefpp-" ("Substring"), w2651, w2602, ".txt" ("Substring")) -> (w2649:string)
        n717 = local read "Plot sample extrema vs time"() -> (w2563:bool)
        n718 = String To Path(string=w2649) -> (path=w2625:path)
        n719 = local read "Time Units"() -> (w2576:u16)
        n720 = Index Array(array=w2606, index=0 ("Index")) -> (element=w2612:dbl)
        n721 = Index Array(array=w2606, index=1 ("Index")) -> (element=w2611:dbl)
        n722 = Number To Decimal String(number=w2612) -> (decimal integer string=w2631:string)  [unwired: 1 in]
        n723 = call "4155C Take Sample FPP.vi"("VISA resource name in"=w2608, "error in (no error)"=w2607, "Emergency Stop"=w2626) -> ("Time"=w2577:dbl[], "Vp1"=w2546:dbl[], "VISA Resource Name out"=w2610:refnum<visa-resource-name>, "Ig"=w2557:dbl[], "Id"=w2556:dbl[], "Vp2"=w2545:dbl[], "error out"=w2559:errorcluster)  [unwired: 10 in]
        n724 = Insert Into Array(array=w2584, new element=w2556) -> (w2543:dbl[])  [unwired: 1 in]
        n725 = case shown="1" w2576 {
          tunnel: [w2692 w2693 w2696] -> w2579
          tunnel: w2577 -> [w2691 w2693 w2695]
          frame 2 {
            n726 = Divide(x=w2691, y=3600.0) -> (x/y=w2692:dbl[])
          }
          frame 0, Default {
          }
          frame 1 {
            n727 = Divide(x=w2695, y=60.0) -> (x/y=w2696:dbl[])
          }
        }
        n728 = Insert Into Array(array=w2585, new element=w2557) -> (w2582:dbl[])  [unwired: 1 in]
        n729 = Number To Decimal String(number=w2611) -> (decimal integer string=w2629:string)  [unwired: 1 in]
        n730 = Add(x=w2579, y=w2578) -> (x+y=w2550:dbl[])
        n731 = case shown="True" w2560 {
          tunnel: w2550 -> [_ w2655]
          tunnel: [w2653 w2656] -> w2561
          tunnel: w2562 -> [w2653 w2654]
          frame False {
          }
          frame True {
            n732 = Insert Into Array(array=w2654, new element=w2655) -> (w2656:i32[])  [unwired: 1 in]
          }
        }
        n733 = case shown="True" w2563 {
          tunnel: w2556 -> [_ w2682]
          tunnel: w2557 -> [_ w2683]
          tunnel: [w2663 w2674] -> w2558
          tunnel: w2559 -> [w2663 w2677]
          tunnel: w2575 -> [w2662 w2667]
          tunnel: w2573 -> [w2661 w2666]
          tunnel: w2571 -> [w2660 w2685]
          tunnel: w2570 -> [w2659 w2684]
          tunnel: w2569 -> [w2658 w2687]
          tunnel: w2568 -> [w2657 w2686]
          tunnel: [w2662 w2667] -> w2574
          tunnel: [w2661 w2666] -> w2572
          tunnel: [w2660 w2665] -> w2567
          tunnel: [w2659 w2664] -> w2566
          tunnel: [w2658 w2676] -> w2565
          tunnel: [w2657 w2672] -> w2564
          tunnel: w2561 -> [_ w2670]
          frame False {
          }
          frame True {
            w2673 = 1
            # "Y1 = Y2 = ID\nY3 = IG"
            # "Number of VAR2 steps is 1."
            # "abs(Ig)"
            # "abs(Id)"
            # "Adjusts graph colors."
            n734 = Absolute Value(x=w2683) -> (abs(x)=w2668:dbl[])
            n735 = Absolute Value(x=w2682) -> (abs(x)=w2669:dbl[])
            n736 = Array Max & Min(array=w2669) -> (max value=w2681:dbl, min value=w2679:dbl)  [unwired: 2 out]
            n737 = Array Max & Min(array=w2668) -> (max value=w2680:dbl, min value=w2678:dbl)  [unwired: 2 out]
            n738 = local write "Id max"(w2681) -> ()
            n739 = local write "Id min"(w2679) -> ()
            n740 = local write "Ig max"(w2680) -> ()
            n741 = local write "Ig min"(w2678) -> ()
            n742 = Insert Into Array(array=w2687, new element=w2668) -> (w2676:dbl[])  [unwired: 1 in]
            n743 = Insert Into Array(array=w2686, new element=w2668) -> (w2672:dbl[])  [unwired: 1 in]
            n744 = Insert Into Array(array=w2685, new element=w2669) -> (w2665:dbl[])  [unwired: 1 in]
            n745 = Insert Into Array(array=w2684, new element=w2669) -> (w2664:dbl[])  [unwired: 1 in]
            n746 = control-ref of="Imax vs time"() -> (w2688:refnum<vi>)
            n747 = call "4155C Config Chart Colours.vi"("Numeric"=w2673, "XY Graph 2"=w2688) -> ()  [unwired: 6 in]
            n748 = call "4155C Split array.vi"("Number of VAR2 steps"=w2673, "Y2 data in"=w2665, "X data in"=w2670, "Y1 data in"=w2665, "Y3 data in"=w2676, "error in (no error)"=w2677) -> ("Array of clusters"=w2689:cluster{"Y data in":dbl[], "X data in":dbl[]}[], "error out"=w2675:errorcluster)  [unwired: 1 in]
            n749 = call "4155C Split array.vi"("Number of VAR2 steps"=w2673, "Y2 data in"=w2664, "X data in"=w2670, "Y1 data in"=w2664, "Y3 data in"=w2672, "error in (no error)"=w2675) -> ("Array of clusters"=w2671:cluster{"Y data in":dbl[], "X data in":dbl[]}[], "error out"=w2674:errorcluster)  [unwired: 1 in]
            n750 = local write "Imax vs time"(w2689) -> ()
            n751 = local write "Imin vs time"(w2671) -> ()
          }
        }
        n752 = Insert Into Array(array=w2583, new element=w2550) -> (w2552:dbl[])  [unwired: 1 in]
        n753 = Concatenate Strings("(Vg = " ("Substring"), w2631, "V, Vd = " ("Substring"), w2629, "V)" ("Substring")) -> (w2627:string)
        n754 = control-ref of="I vs time (Bias Stress)"() -> (w2580:refnum<vi>)
        n755 = call "4155C Split array.vi"("Number of VAR2 steps"=w2551, "Y2 data in"=w2543, "X data in"=w2552, "Y1 data in"=w2543, "Y3 data in"=w2582) -> ("Array of clusters"=w2581:cluster{"Y data in":dbl[], "X data in":dbl[]}[])  [unwired: 2 in, 1 out]
        n756 = local write "I vs time (Bias Stress)"(w2581) -> ()
        n757 = call "4155C Config Chart Colours.vi"("Numeric"=w2551, "XY Graph 2"=w2580) -> ()  [unwired: 6 in]
        n758 = Insert Into Array(array=dbl[][] [] ("Input Array"), new element=w2550) -> (w2638:dbl[][])  [unwired: 2 in]
        n759 = Insert Into Array(array=w2549, new element=w2546) -> (w2544:dbl[])  [unwired: 1 in]
        n760 = Insert Into Array(array=w2638, new element=w2556) -> (w2637:dbl[][])  [unwired: 2 in]
        n761 = call <vilib>:"compatOverwrite.vi"("overwrite (F)"=TRUE) -> ("overwrite?"=w2604:T8)
        n762 = Open/Create/Replace File(file path (use dialog)=w2625, error in=w2558, operation (0:open)=w2604) -> (refnum out=w2622:refnum<file>, error out=w2623:errorcluster)  [unwired: 3 in, 1 out]
        n763 = Array To Spreadsheet String(array=w2613, 3:w2617) -> (spreadsheet string=w2619:string)  [unwired: 1 in]
        n764 = Insert Into Array(array=w2637, new element=w2557) -> (w2636:dbl[][])  [unwired: 2 in]
        n765 = Insert Into Array(array=w2548, new element=w2545) -> (w2547:dbl[])  [unwired: 1 in]
        n766 = Search and Replace String(replace all?=TRUE ("replace all? (F)"), input string=w2619, search string="VgVd", replace string=w2627) -> (result string=w2615:string)  [unwired: 4 in, 3 out]
        n767 = Insert Into Array(array=w2636, new element=w2546) -> (w2634:dbl[][])  [unwired: 2 in]
        n768 = Spreadsheet String To Array(format string=w2617, spreadsheet string=w2615, array type (2D Dbl)=w2613) -> (array=w2614:string[])  [unwired: 1 in]
        n769 = Insert Into Array(array=w2634, new element=w2545) -> (w2605:dbl[][])  [unwired: 2 in]
        n770 = control-ref of="Vp vs time (FPP Bias Stress)"() -> (w2553:refnum<vi>)
        n771 = Transpose 2D Array(2D array=w2605) -> (transposed array=w2633:dbl[][])
        n772 = call "4155C Write array to file.vi"("Byte Stream File Refnum"=w2622, "Header"=w2614, "Data Array"=w2633, "error in (no error)"=w2623) -> ("dup refnum"=w2620:refnum<file>, "error out"=w2621:errorcluster)  [unwired: 1 in]
        n773 = Close File(refnum=w2620, error in=w2621) -> (error out=w2609:errorcluster)  [unwired: 1 out]
        n774 = call "4155C Split array.vi"("Number of VAR2 steps"=w2551, "Y2 data in"=w2544, "X data in"=w2552, "Y1 data in"=w2547, "Y3 data in"=w2544) -> ("Array of clusters"=w2554:cluster{"Y data in":dbl[], "X data in":dbl[]}[])  [unwired: 2 in, 1 out]
        n775 = local write "Vp vs time (FPP Bias Stress)"(w2554) -> ()
        n776 = call "4155C Config Chart Colours.vi"("Numeric"=w2551, "XY Graph 2"=w2553) -> ()  [unwired: 6 in]
      }
      frame "serial" {
        n777 = local read "Termination char\n(0xA = '\\n' = LF)\n(0xD = '\\r' = CR)"() -> (w2732:u8)
        n778 = local read "Enable Termination\nChar (T)"() -> (w2733:bool)
        n779 = Index Array(array=w2740, index=0 ("Index")) -> (element=w2739:string)
        n780 = local read "parity"() -> (w2723:u16)
        n781 = local read "Delay before read (ms)"() -> (w2734:u32)
        n782 = local read "byte count"() -> (w2731:u32)
        n783 = local read "VISA resource name"() -> (w2727:refnum<visa-resource-name>)
        n784 = local read "baud rate"() -> (w2726:u32)
        n785 = local read "Serial End Mode for Reads"() -> (w2725:u16)
        n786 = local read "Timeout (ms)"() -> (w2730:u32)
        n787 = local read "data bits"() -> (w2724:u16)
        n788 = local read "stop bits"() -> (w2729:u16)
        n789 = local read "flow control"() -> (w2728:u16)
        n790 = call "Serial write and read v0.5.vi"("Delay before read (ms)"=w2734, "Termination char\n(0xA = '\\n' = LF)\n(0xD = '\\r' = CR)"=w2732, "Enable Termination\nChar (T)"=w2733, "parity"=w2723, "stop bits"=w2729, "string to write"=w2739, "flow control"=w2728, "byte count"=w2731, "Serial Settings:Serial End Mode for Reads"=w2725, "Timeout (ms)"=w2730, "error in (no error)"=w2745, "VISA resource name"=w2727, "baud rate"=w2726, "data bits"=w2724) -> ("Serial port output"=w2735:string, "error out"=w2744:errorcluster)
        n791 = Build Array (concatenate)(w2735, w2736) -> (w2737:string[])
      }
      frame "pump" {
        # "Time array for valve position"
        # "Time array for absolute plunger position"
        # "Valve position"
        # "Absolute plunger position"
        # "Remove \"_\""
        # "Check if pump is idle. Else halt."
        n792 = Index Array(array=w2817, index=0 ("Index")) -> (element=w2798:string)
        n793 = local read "Hard stop pump"() -> (w2757:bool)
        n794 = local read "Halt pump"() -> (w2758:bool)
        n795 = local read "Serial End Mode for Reads"() -> (w2805:u16)
        n796 = local read "flow control"() -> (w2808:u16)
        n797 = local read "stop bits"() -> (w2809:u16)
        n798 = local read "parity"() -> (w2803:u16)
        n799 = local read "Delay before read (ms)"() -> (w2814:u32)
        n800 = local read "byte count"() -> (w2811:u32)
        n801 = local read "VISA resource name"() -> (w2807:refnum<visa-resource-name>)
        n802 = local read "baud rate"() -> (w2806:u32)
        n803 = local read "Timeout (ms)"() -> (w2810:u32)
        n804 = local read "Termination char\n(0xA = '\\n' = LF)\n(0xD = '\\r' = CR)"() -> (w2812:u8)
        n805 = local read "Enable Termination\nChar (T)"() -> (w2813:bool)
        n806 = case shown="\"Internal failure\"" w2797 {
          tunnel: w2798 -> [w2853 _ w2855 w2856 w2857 w2858 _ _ w2861 w2862 _]
          tunnel: [w2853 "/1H" w2855 w2856 w2857 w2858 "/1H" "/1H" w2861 w2862 "/1H"] -> w2759
          frame "No error", Default {
          }
          frame "Initialization" {
          }
          frame "Invalid command" {
          }
          frame "Invalid operand" {
          }
          frame "Device not initialized" {
          }
          frame "Internal failure" {
          }
          frame "Plunger overload" {
          }
          frame "Valve overload" {
          }
          frame "Plunger move not allowed" {
          }
          frame "A/D converter failure" {
          }
          frame "Command overflow" {
          }
        }
        n807 = local read "data bits"() -> (w2804:u16)
        n808 = String Subset(string=w2793, offset (0)=1) -> (substring=w2791:string)  [unwired: 1 in]
        n809 = call "SPM Pump v0.7.vi"("Termination char\n(0xA = '\\n' = LF)\n(0xD = '\\r' = CR)"=w2812, "Enable Termination\nChar (T)"=w2813, "Timeout (ms)"=w2810, "Serial Settings:Serial End Mode for Reads"=w2805, "byte count"=w2811, "Delay before read (ms)"=w2814, "Time <input>"=w2796, "error in (no error)"=w2822, "Serial port input"=w2759, "VISA resource name"=w2807, "parity"=w2803, "baud rate"=w2806, "stop bits"=w2809, "data bits"=w2804, "flow control"=w2808, "Time units <input>"=w2791, "Hard stop pump"=w2757, "Halt pump"=w2758) -> ("Input command"=w2790:string, "Serial port data"=w2780:string[], "Pump status"=w2786:string, "Valve position"=w2788:i32, "Absolute plunger position"=w2799:i32, "Serial port"=w2795:string, "error out"=w2821:errorcluster)  [unwired: 2 in, 1 out]
        n810 = case shown="\"?6\"" w2790 {
          tunnel: [w2834 w2842 w2848] -> w2802
          tunnel: w2801 -> [w2834 w2841 w2848]
          tunnel: w2799 -> [_ w2840 _]
          tunnel: w2787 -> [w2833 w2839 w2849]
          tunnel: [w2833 w2839 w2851] -> w2789
          tunnel: w2788 -> [_ _ w2850]
          tunnel: w2785 -> [_ w2838 w2846]
          tunnel: w2784 -> [w2832 w2837 w2847]
          tunnel: [w2832 w2836 w2847] -> w2783
          tunnel: [w2831 w2835 w2845] -> w2782
          tunnel: w2781 -> [w2831 w2835 w2844]
          frame "Q", Default {
          }
          frame "?" {
            n811 = Build Array (concatenate)(w2841, w2840) -> (w2842:i32[])
            n812 = Build Array (concatenate)(w2837, w2838) -> (w2836:i32[])
            n813 = call "4155C Split array.vi"("X data in"=w2836, "Y1 data in"=w2842) -> ("Array of clusters"=w2843:cluster{"Y data in":dbl[], "X data in":dbl[]}[])  [unwired: 5 in, 1 out]
            n814 = local write "Absolute plunger position vs time"(w2843) -> ()
          }
          frame "?6" {
            n815 = Build Array (concatenate)(w2849, w2850) -> (w2851:i32[])
            n816 = Build Array (concatenate)(w2844, w2846) -> (w2845:i32[])
            n817 = call "4155C Split array.vi"("X data in"=w2845, "Y1 data in"=w2851) -> ("Array of clusters"=w2852:cluster{"Y data in":dbl[], "X data in":dbl[]}[])  [unwired: 5 in, 1 out]
            n818 = local write "Valve position vs time"(w2852) -> ()
          }
        }
        n819 = Build Array (concatenate)(w2778, w2780) -> (w2779:string[][])
        n820 = Build Array (concatenate)(w2794, w2795) -> (w2815:string[])
      }
      frame "filename" {
        n821 = Index Array(array=w2874, index=0 ("Index")) -> (element=w2873:string)
      }
    }
    "Probe 4 Indicator" <- w79
    "Timings Indicator" <- w78
    n822 = local read "Time Units"() -> (w112:u16)
    n823 = case shown="0" w112 {
      tunnel: ["Time (Seconds)" ("element") "Time (Minutes)" ("element") "Time (Hours)" ("element")] -> w80
      frame 0 {
      }
      frame 1, Default {
      }
      frame 2 {
      }
    }
    n824 = Build Array(w186, w119, w129, w128, w127, w126, w125, w124, w123, w122, w121, w120, w118) -> (w224:dbl[][])
    n825 = Transpose 2D Array(2D array=w224) -> (transposed array=w223:dbl[][])
    n826 = Concatenate Strings(w87, w86, "I-vs-time.txt" ("Suffix (Imax,Imin,Ion,Ioff)")) -> (w234:string)
    n827 = Build Array(w80, "Is max (A)" ("VAR2 Name"), "Is min (A)" ("VAR2 Name"), "Id max (A)" ("VAR2 Name"), "Id min (A)" ("VAR2 Name"), "Ig max (A)" ("VAR2 Name"), "Ig min (A)" ("VAR2 Name"), "Is on (A)" ("VAR2 Name"), "Is off (A)" ("VAR2 Name"), "Id on (A)" ("VAR2 Name"), "Id off (A)" ("VAR2 Name"), "Ig on (A)" ("VAR2 Name"), "Ig off (A)" ("VAR2 Name")) -> (w229:string[])
    n828 = Array To Spreadsheet String(array=w223, 3:"%e" ("format string")) -> (spreadsheet string=w227:string)  [unwired: 1 in]
    n829 = Array To Spreadsheet String(array=w229, 3:"" ("format string")) -> (spreadsheet string=w228:string)  [unwired: 1 in]
    n830 = String To Path(string=w234) -> (path=w233:path)
    n831 = Build Array(w228, w227) -> (w226:string[])
    n832 = Write to Text File(file (use dialog)=w233, text=w226, error in=w183) -> (refnum out=w235:refnum<file>, error out=w225:errorcluster)  [unwired: 1 in, 1 out]
    n833 = Close File(refnum=w235, error in=w225) -> (error out=w167:errorcluster)  [unwired: 1 out]
    n834 = Build Array(w164, w187) -> (w192:i32[][])
    n835 = Build Array(w80, "Absolute plunger position" ("VAR2 Name")) -> (w195:string[])
    n836 = Transpose 2D Array(2D array=w192) -> (transposed array=w185:i32[][])
    n837 = Array To Spreadsheet String(array=w195, 3:"" ("format string")) -> (spreadsheet string=w194:string)  [unwired: 1 in]
    n838 = Array To Spreadsheet String(array=w185, 3:"%e" ("format string")) -> (spreadsheet string=w191:string)  [unwired: 1 in]
    n839 = Build Array(w194, w191) -> (w197:string[])
    n840 = Concatenate Strings(w87, w86, "plunger.txt" ("Suffix (plunger)")) -> (w189:string)
    n841 = String To Path(string=w189) -> (path=w188:path)
    n842 = Write to Text File(file (use dialog)=w188, text=w197, error in=w167) -> (refnum out=w190:refnum<file>, error out=w199:errorcluster)  [unwired: 1 in, 1 out]
    n843 = Close File(refnum=w190, error in=w199) -> (error out=w166:errorcluster)  [unwired: 1 out]
    n844 = Concatenate Strings(w87, w86, "serial-port.txt" ("Suffix (serial port log)")) -> (w205:string)
    n845 = String To Path(string=w205) -> (path=w204:path)
    n846 = Build Array(w80, "Serial port input" ("VAR2 Name"), "Pump status" ("VAR2 Name"), "Serial port output: ") -> (w154:string[])
    n847 = Array To Spreadsheet String(array=w160, 3:"" ("format string")) -> (spreadsheet string=w151:string)  [unwired: 1 in]
    n848 = Array To Spreadsheet String(array=w154, 3:"" ("format string")) -> (spreadsheet string=w152:string)  [unwired: 1 in]
    n849 = Array To Spreadsheet String(array=w159, 3:"" ("format string")) -> (spreadsheet string=w210:string)  [unwired: 1 in]
    n850 = Build Array(w152, w151) -> (w153:string[])
    n851 = Write to Text File(file (use dialog)=w204, text=w153, error in=w166) -> (refnum out=w206:refnum<file>, error out=w207:errorcluster)  [unwired: 1 in, 1 out]
    n852 = local write "Serial port data"(w210) -> ()
    n853 = Close File(refnum=w206, error in=w207) -> (error out=w165:errorcluster)  [unwired: 1 out]
    n854 = Build Array(w163, w169) -> (w175:i32[][])
    n855 = Build Array(w80, "Valve port" ("VAR2 Name")) -> (w178:string[])
    n856 = Transpose 2D Array(2D array=w175) -> (transposed array=w170:i32[][])
    n857 = Array To Spreadsheet String(array=w178, 3:"" ("format string")) -> (spreadsheet string=w177:string)  [unwired: 1 in]
    n858 = Array To Spreadsheet String(array=w170, 3:"%e" ("format string")) -> (spreadsheet string=w174:string)  [unwired: 1 in]
    n859 = Build Array(w177, w174) -> (w180:string[])
    n860 = Concatenate Strings(w87, w86, "valve-port.txt" ("Suffix (valve)")) -> (w172:string)
    n861 = String To Path(string=w172) -> (path=w171:path)
    n862 = Write to Text File(file (use dialog)=w171, text=w180, error in=w165) -> (refnum out=w173:refnum<file>, error out=w182:errorcluster)  [unwired: 1 in, 1 out]
    n863 = Close File(refnum=w173, error in=w182) -> (error out=w88:errorcluster)  [unwired: 1 out]
    n864 = Build Array(w85, w84, w83, w82) -> (w97:dbl[][])
    n865 = Build Array(w80, "Is (A)" ("VAR2 Name"), "Id (A)" ("VAR2 Name"), "Ig (A)" ("VAR2 Name")) -> (w93:string[])
    n866 = Transpose 2D Array(2D array=w97) -> (transposed array=w96:dbl[][])
    n867 = Concatenate Strings(w87, w86, "sample.txt" ("Suffix (Imax,Imin,Ion,Ioff)")) -> (w103:string)
    n868 = Array To Spreadsheet String(array=w93, 3:"" ("format string")) -> (spreadsheet string=w92:string)  [unwired: 1 in]
    n869 = Array To Spreadsheet String(array=w96, 3:"%e" ("format string")) -> (spreadsheet string=w100:string)  [unwired: 1 in]
    n870 = local write "Hard stop pump"(w72) -> ()
    n871 = String To Path(string=w103) -> (path=w102:path)
    n872 = local write "Halt pump"(w72) -> ()
    n873 = Build Array(w92, w100) -> (w99:string[])
    n874 = Write to Text File(file (use dialog)=w102, text=w99, error in=w88) -> (refnum out=w104:refnum<file>, error out=w98:errorcluster)  [unwired: 1 in, 1 out]
    n875 = Close File(refnum=w104, error in=w98) -> (error out=w77:errorcluster)  [unwired: 1 out]
    "error out" <- w77
  }
  "Is max" <- w17
  "Id max" <- w17
  "Ig max" <- w17
  "Imax vs time" <- w4
  "I vs Vg" <- w4
  "Imin vs time" <- w4
  "I vs Vd" <- w4
  "Serial port data" <- "" ("Serial port data")
  "Absolute plunger position vs time" <- w4
  "Valve position vs time" <- cluster{"Y data in":dbl[], "X data in":dbl[]}[] [] ("Valve position vs time")
  "Is min" <- w16
  "Id min" <- w16
  "Ig min" <- w16
  "Ion vs time" <- w4
  "Ioff vs time" <- w4
  "Is on" <- w15
  "Id on" <- w15
  "Ig on" <- w15
  "Is off" <- w14
  "Id off" <- w14
  "Ig off" <- w14
  "I vs time (Bias Stress)" <- w4
  "Vp1" <- w5
  "Vp2" <- w5
  "Vp vs time (FPP Bias Stress)" <- w4
  "Vp vs Vg (FPP)" <- w4
  "Vdg vs time (Bias Stress)" <- w4
